vi "Run.vi"(8 "error in (no error)":errorcluster, 11 "Channel in":refnum<class "Channel.lvclass">) -> (0 "error out":errorcluster, 3 "Channel out":refnum<class "Channel.lvclass">)   [LabVIEW 2018, in "Channel.lvclass"]
uses:
  Channel.lvclass
  C:/Users/devstaff/sparc4/s4gui/Versao ZeroMQ REQ-REP/SPARC4_GUI -v1.0.9 - novo comportamento aba TEST/Device/Device.lvclass
  Channel.lvclass/Channel.ctl
  Interface/Interface.lvclass/Interface.ctl
  Device/Device.lvclass/Device.ctl
  StateMachine/State Machine.lvclass
  Interface/Interface.lvclass
  Device/Device.lvclass
panel:
  out "resp RESUME":string
  out "resp PAUSE":string
  out "x = y?":T1
  out "resposta do STATUS":string
  out "resp INIT":string
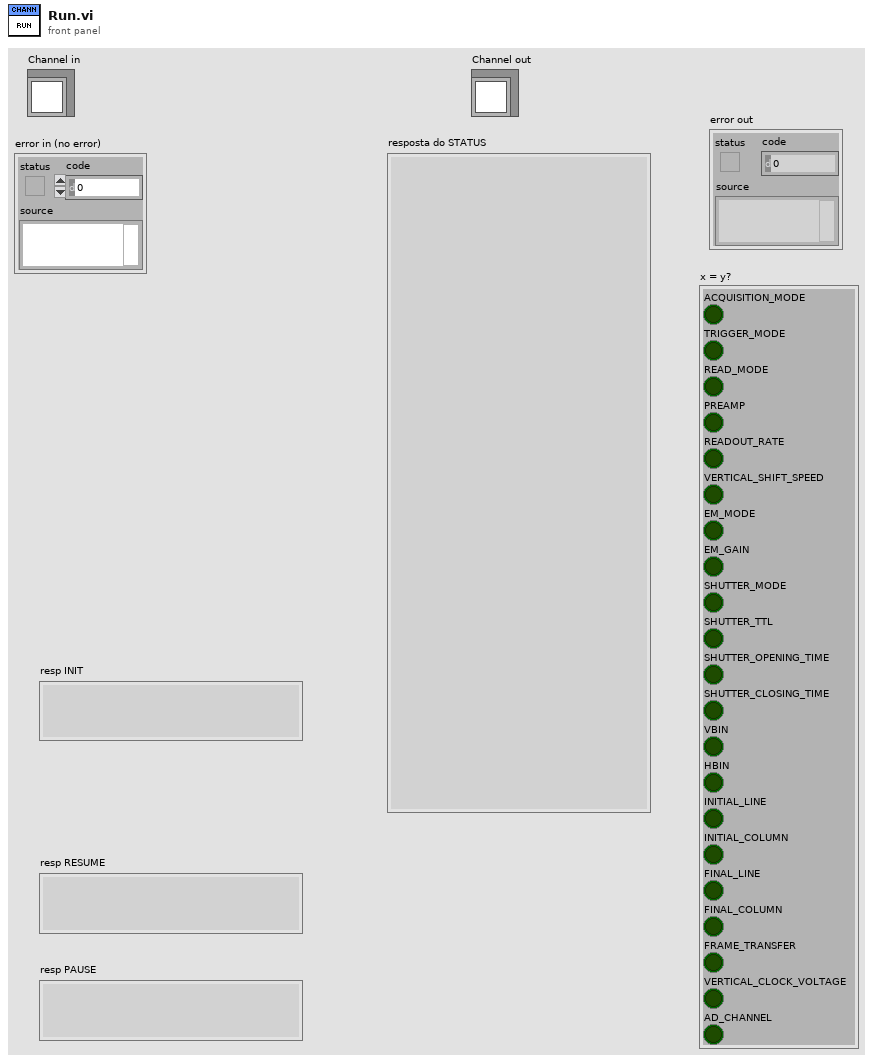
[diagram p1: front panel]
types:
  T1 = cluster{"ACQUISITION_MODE":bool, "TRIGGER_MODE":bool, "READ_MODE":bool, "PREAMP":bool, "READOUT_RATE":bool, "VERTICAL_SHIFT_SPEED":bool, "EM_MODE":bool, "EM_GAIN":bool, "SHUTTER_MODE":bool, "SHUTTER_TTL":bool, "SHUTTER_OPENING_TIME":bool, "SHUTTER_CLOSING_TIME":bool, "VBIN":bool, "HBIN":bool, "INITIAL_LINE":bool, "INITIAL_COLUMN":bool, "FINAL_LINE":bool, "FINAL_COLUMN":bool, "FRAME_TRANSFER":bool, "VERTICAL_CLOCK_VOLTAGE":bool, "AD_CHANNEL":bool}
  T2 = cluster{"TEMP":dbl, "EXPTIME":dbl, "#FRAMES":u32, "#CYCLES":u32, "#SEQS":u32, "WAVEPLATE_POS":u32, "COOLER_POWER_STATUS":dbl, "suffix":string}
  T3 = cluster{"ACQUISITION_MODE":u8, "TRIGGER_MODE":u8, "READ_MODE":u8, "PREAMP":u8, "READOUT_RATE":u8, "VERTICAL_SHIFT_SPEED":u8, "EM_MODE":u8, "EM_GAIN":u16, "SHUTTER_MODE":u8, "SHUTTER_TTL":u8, "SHUTTER_OPENING_TIME":u16, "SHUTTER_CLOSING_TIME":u16, "VBIN":u16, "HBIN":u16, "INITIAL_LINE":u16, "INITIAL_COLUMN":u16, "FINAL_LINE":u16, "FINAL_COLUMN":u16, "FRAME_TRANSFER":bool, "VERTICAL_CLOCK_VOLTAGE":u8, "AD_CHANNEL":u32}
  T4 = cluster{"Image Name":string, "Image Path":string, "#FRAMES":u32, "EXPTIME":dbl, "PREAMP":u8, "READOUT_RATE":u8, "VERTICAL_SHIFT_SPEED":u8, "ACQUISITION_MODE":u8, "READ_MODE":u8, "EM_MODE":u8, "EM_GAIN":u16, "SHUTTER_MODE":u8, "SHUTTER_TTL":u8, "SHUTTER_OPENNING_TIME":u16, "SHUTTER_CLOSING_TIME":u16, "VBIN":u16, "HBIN":u16, "INITIAL_LINE":u16, "INITIAL_COLUMN":u16, "FINAL_LINE":u16, "FINAL_COLUMN":u16, "Cooler ON/OFF":u16, "Set temperature":i8, "Exposições realizadas":u16, "Kinetic Serie Length":u32, "Number of Accumulations":u32, "Kinetic Cycle Time":u32, "FRAME_TRANSFER":bool, "VERTICAL_CLOCK_VOLTAGE":u8, "TRIGGER_MODE":u8, "Number of exp":u32, "AD_CHANNEL":u32}
  T5 = cluster{"OBSERVER":string, "OBJECT":string, "CTRLINTE":string, "PROJID":string, "SYNCMODE":string, "INSTMODE":string, "FILTER":string, "OBSTYPE":string, "CHANNEL 1":bool, "CHANNEL 2":bool, "CHANNEL 3":bool, "CHANNEL 4":bool, "TCSMODE":bool, "COMMENT":string, "broker":string, "GUIVRSN":string, "timestamp":string}
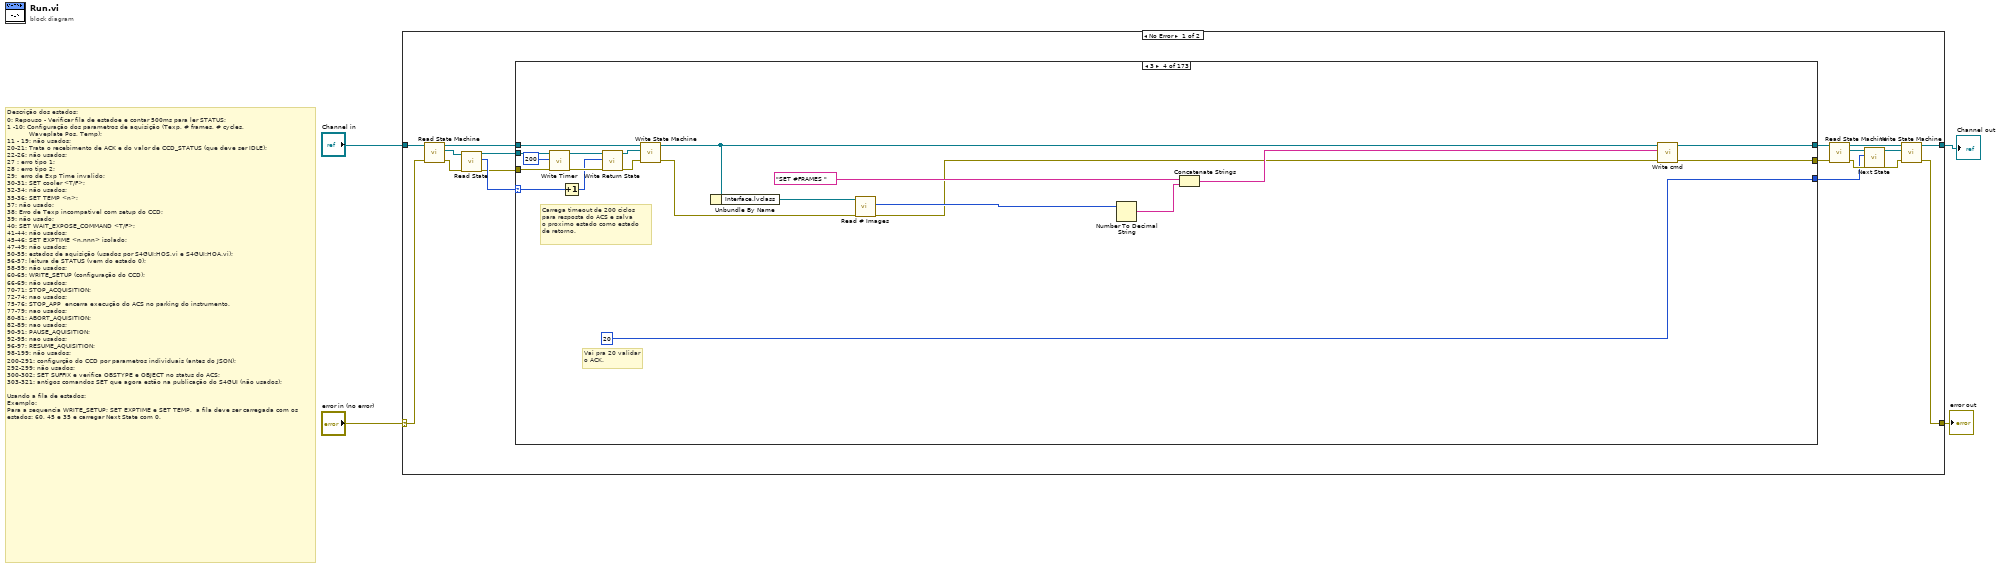
[diagram p0: block diagram]
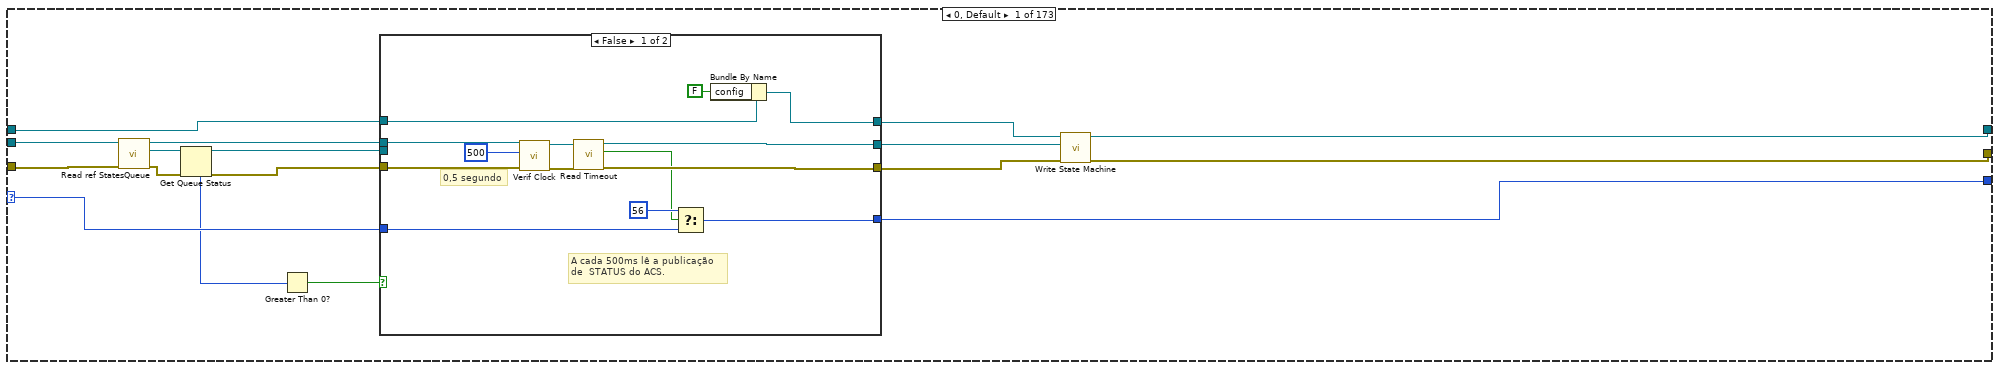
[diagram p2: hidden frame]
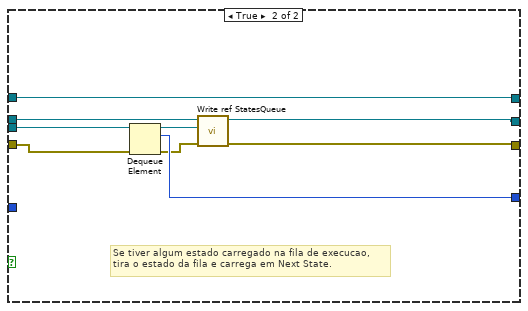
[diagram p3: hidden frame]
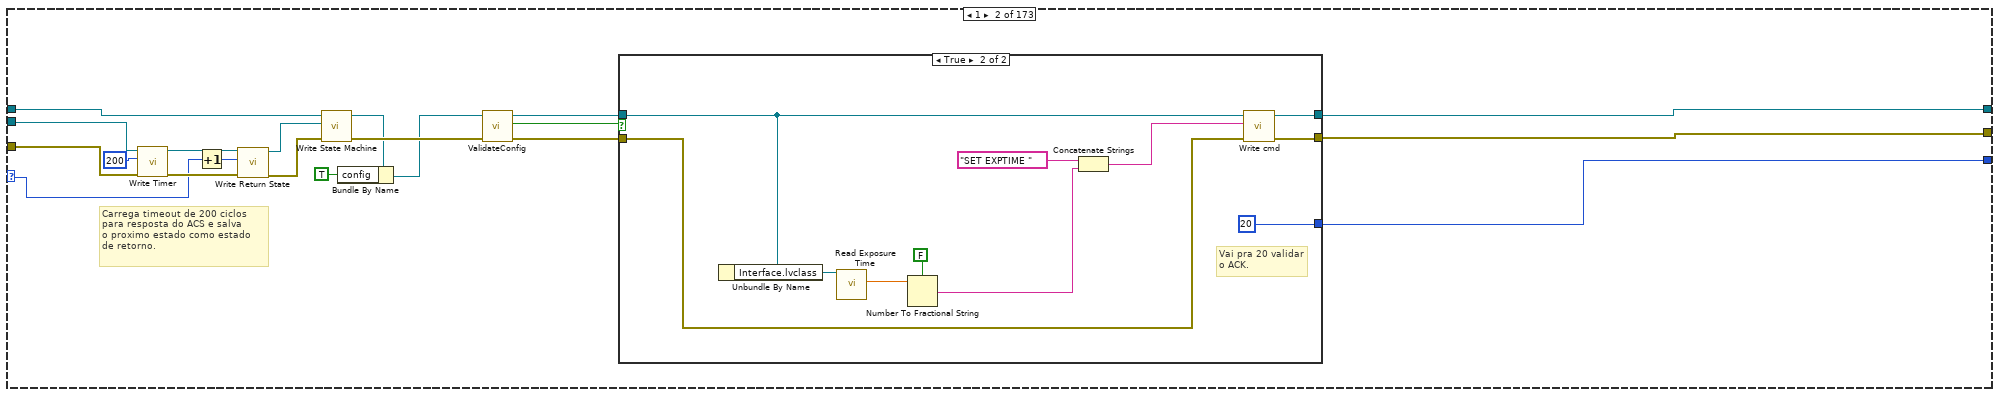
[diagram p4: hidden frame]
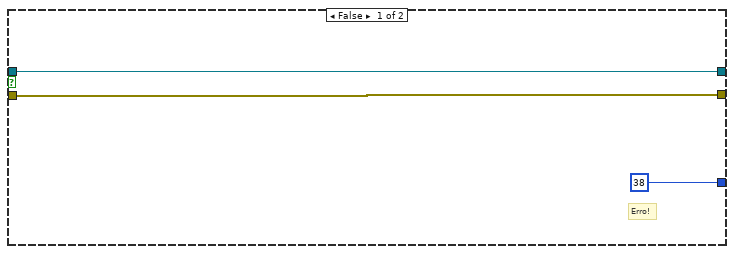
[diagram p5: hidden frame]
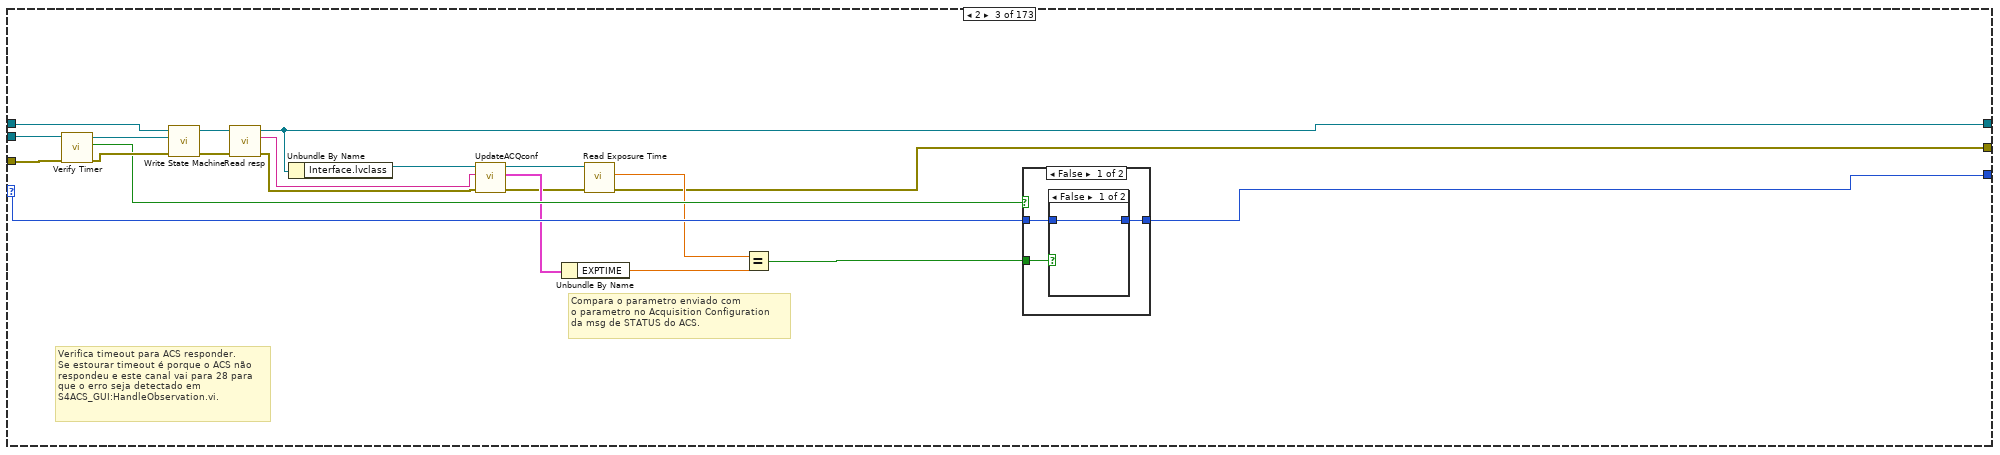
[diagram p6: hidden frame]
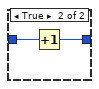
[diagram p7: hidden frame]
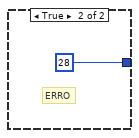
[diagram p8: hidden frame]
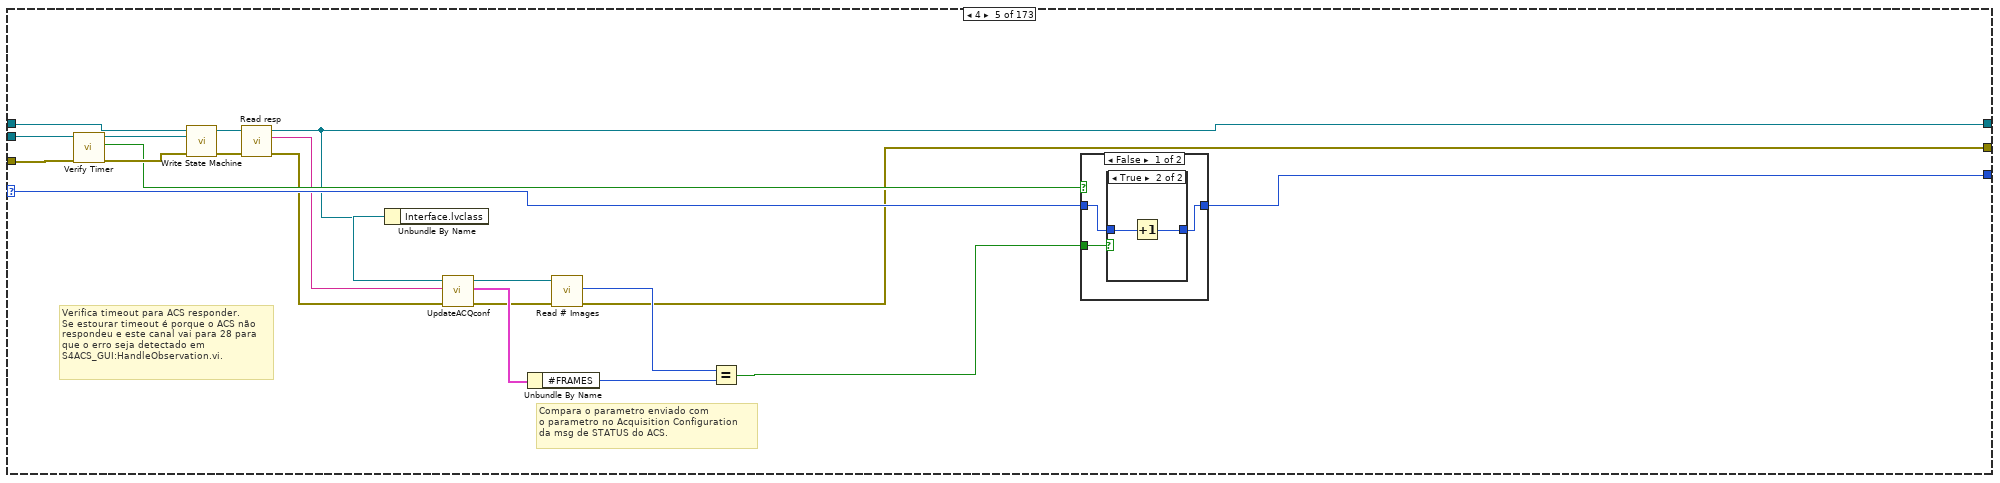
[diagram p9: hidden frame]
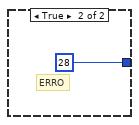
[diagram p11: hidden frame]
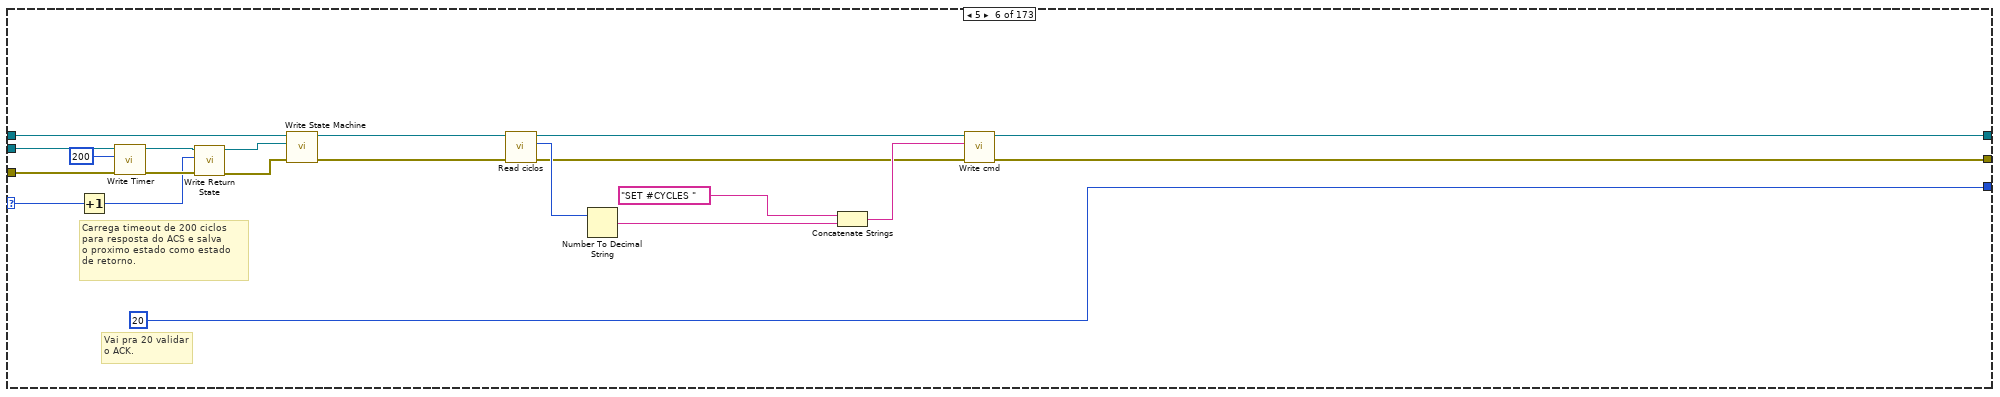
[diagram p12: hidden frame]
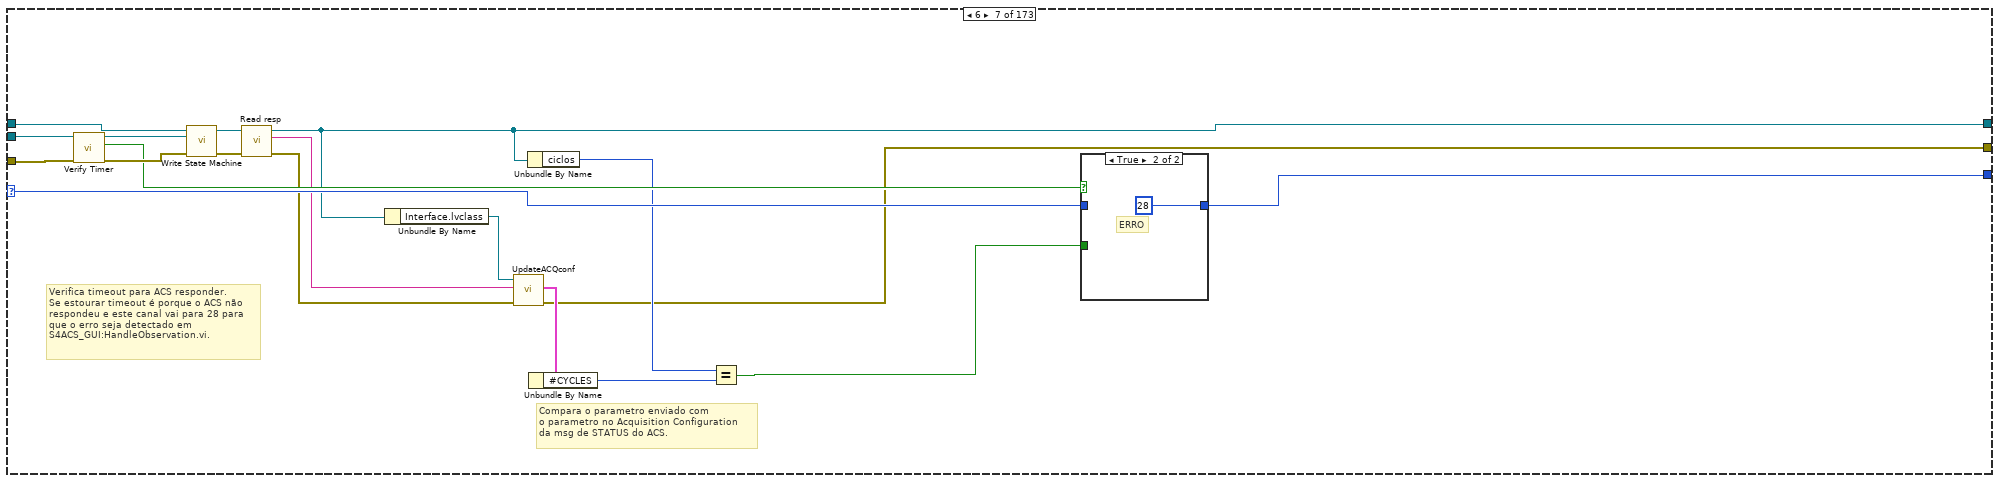
[diagram p13: hidden frame]
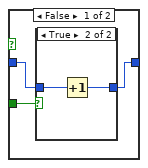
[diagram p14: hidden frame]
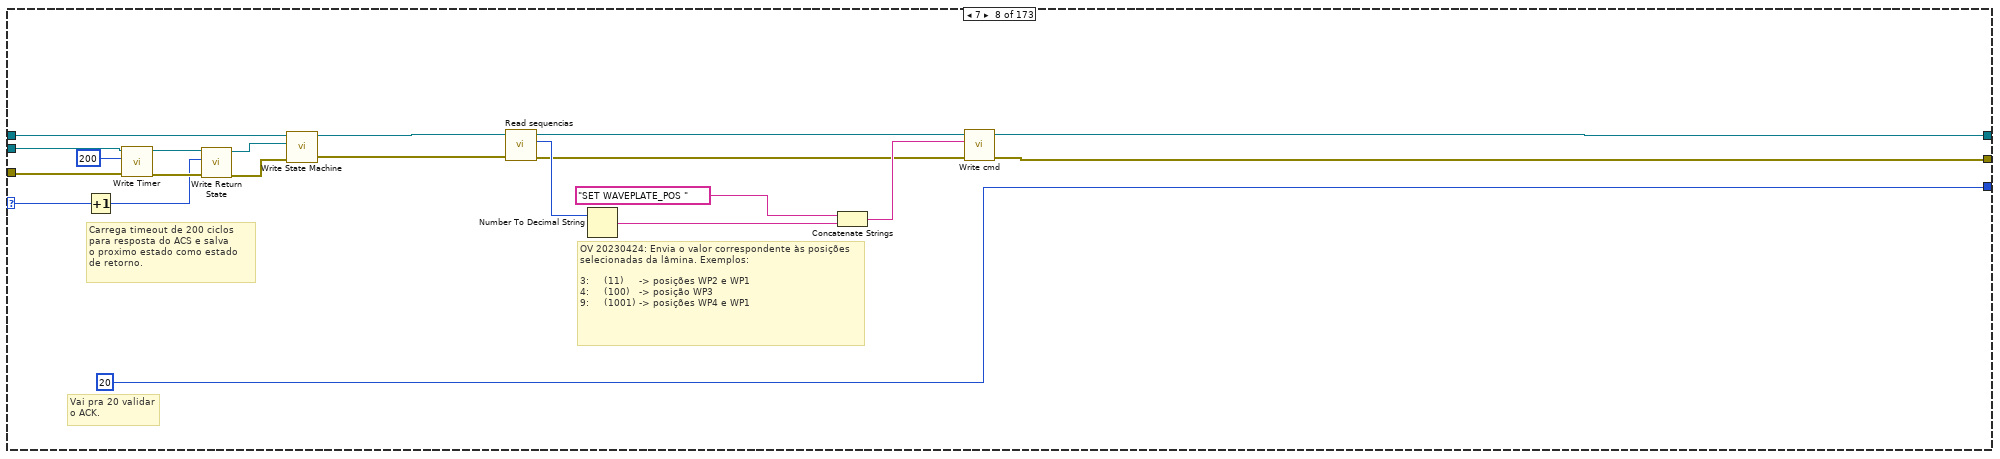
[diagram p16: hidden frame]
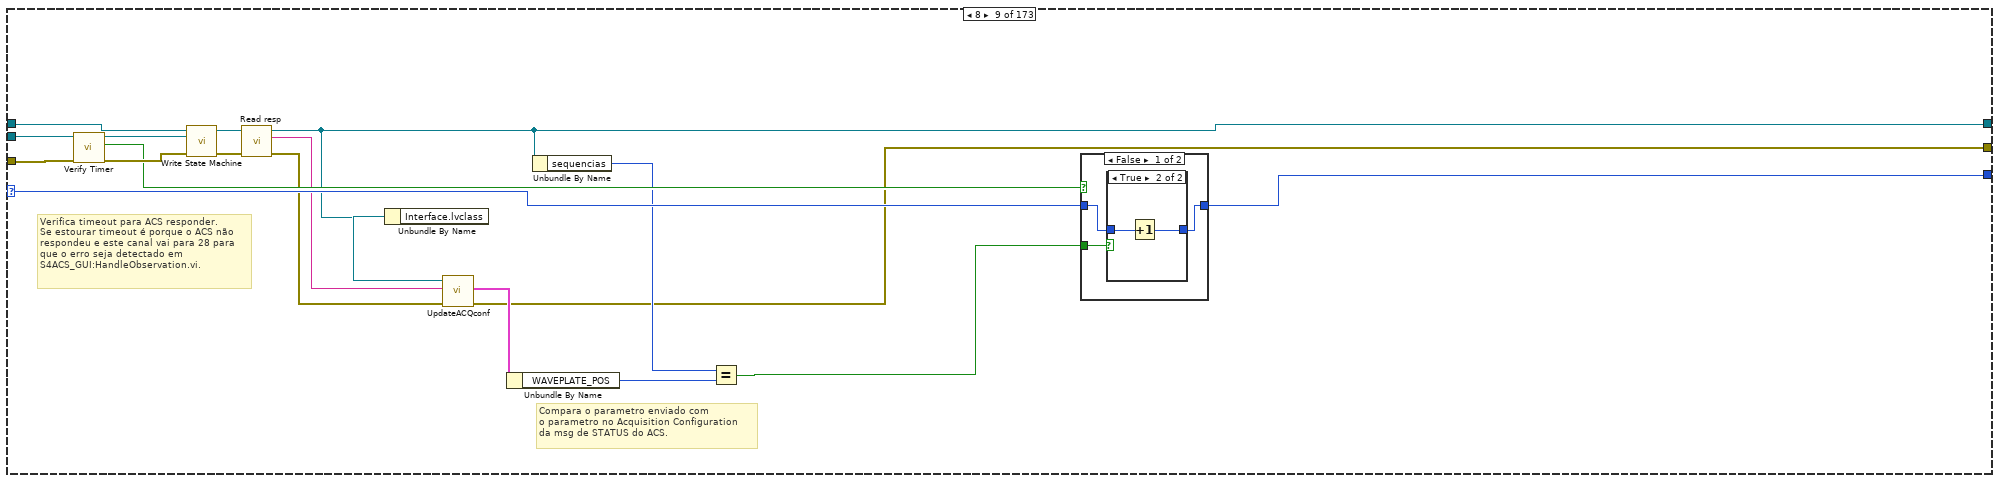
[diagram p17: hidden frame]
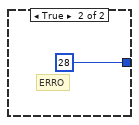
[diagram p19: hidden frame]
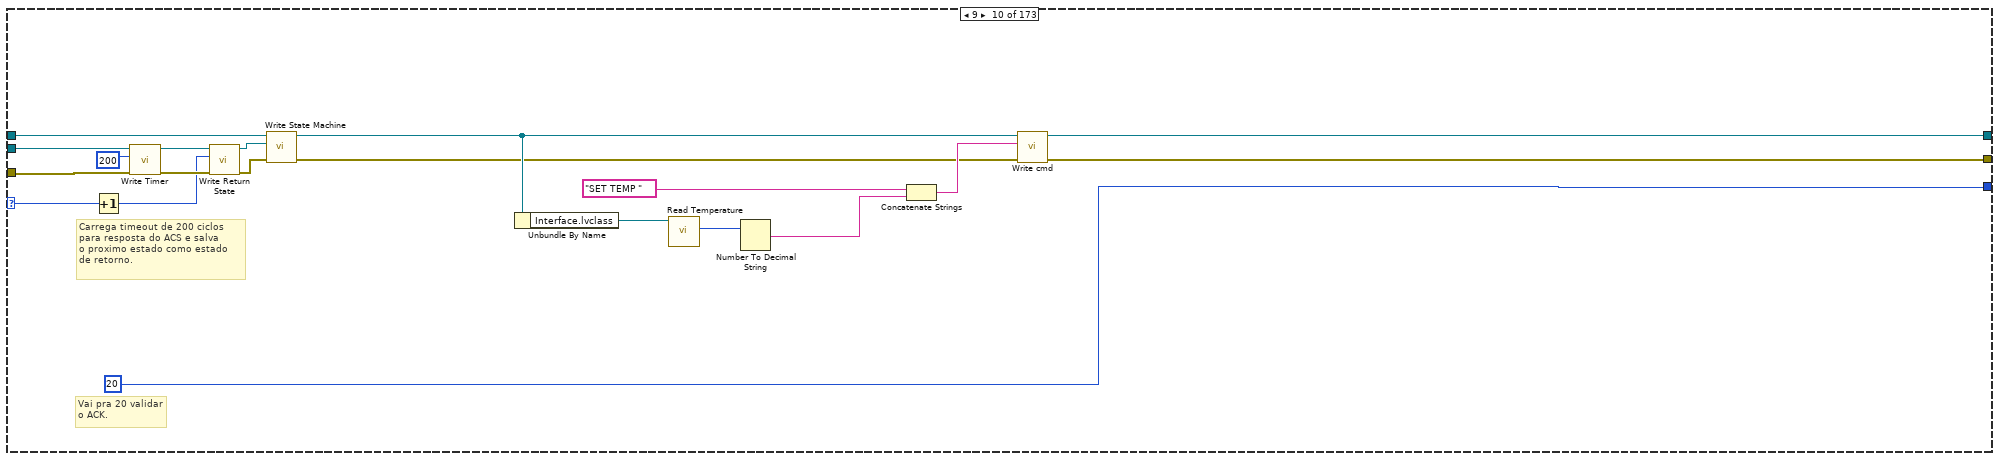
[diagram p20: hidden frame]
diagram:
  # "Descrição dos estados:\n0: Repouso - Verificar fila de estadoe e contar 500ms para ler STATUS;\n1 -10: Configuração dos parametros de aquisição (Texp, # frames, # cycles,\n           Waveplate Pos, Temp);\n11 - 19: não usados;\n20-21: Trata o recebimento de ACK e do valor de CCD_STATUS (que deve ser IDLE);\n22-26: não usados;\n27 : erro tipo 1;\n28 : erro tipo 2;\n29:  erro de Exp Time invalido;\n30-31: SET cooler <T/F>;\n32-34: não usados;\n35-36: SET TEMP <n>;\n37: não usado;\n38: Erro de Texp incompativel com setup do CCD;\n39: não usado;\n40: SET WAIT_EXPOSE_COMMAND <T/F>;\n41-44: não usados;\n45-46: SET EXPTIME <n.nnn> isolado;\n47-49: não usados;\n50-55: estados de aquisição (usados por S4GUI:HOS.vi e S4GUI:HOA.vi);\n56-57: leitura de STATUS (vem do estado 0);\n58-59: não usados;\n60-65: WRITE_SETUP (configuração do CCD);\n66-69: não usados;\n70-71: STOP_ACQUISITION;\n72-74: nao usados;\n75-76: STOP_APP  encerra execução do ACS no parking do instrumento.\n77-79: nao usados;\n80-81: ABORT_AQUISITION;\n82-89: nao usados;\n90-91: PAUSE_AQUISITION;\n92-95: nao usados;\n96-97: RESUME_AQUISITION;\n98-199: não usados;\n200-291: configurção do CCD por parametros individuais (antes do JSON);\n292-299: não usados;\n300-302: SET SUFFIX e verifica OBSTYPE e OBJECT no status do ACS;\n303-321: antigos comandos SET que agora estão na publicação do S4GUI (não usados);\n\nUsando a fila de estados:\nExemplo:\nPara a sequencia WRITE_SETUP; SET EXPTIME e SET TEMP,  a fila deve ser carregada com os \nestados: 60, 45 e 35 e carregar Next State com 0."
  n1 = case shown="No Error" "error in (no error)" {
    selector: "error in (no error)" -> [w21 w3263]
    tunnel: [w6 w3263] -> w3
    tunnel: [w11 w3262] -> w1
    tunnel: "Channel in" -> [w22 w3262]
    frame No Error {
      n2 = call-dynamic "Read State Machine.vi"("error in (no error)"=w21, "Device in"=w22) -> ("error out"=w18:errorcluster, "State Machine.lvclass"=w20:refnum<class "State Machine.lvclass">, "Device out"=w16:refnum<class "Channel.lvclass">)  [unwired: 7 in]
      n3 = call-dynamic "Read State.vi"("error in (no error)"=w18, "State Machine in"=w20) -> ("error out"=w17:errorcluster, "State"=w19:i32, "State Machine out"=w5:refnum<class "State Machine.lvclass">)  [unwired: 7 in]
      n4 = case shown="3" w19 {
        selector: w19 -> [w39 w64 w110 w127 w158 w176 w205 w221 w252 w269 w308 w330 w364 w442 w485 w528 w543 w571 w590 w603 w649 w678 _ w751 _ w790 w824 w850 w879 w890 w951 w972 w1046 w1086 w1154 _ _ w1262 w1293 w1314 w1352 w1365 w1381 w1447 w1481 w1506 w1514 w1558 w1564 w1586 w1592 w1635 _ w1660 _ w1679 w1690 w1710 w1730 w1750 w1770 w1790 w1810 w1830 w1850 _ w1870 w1878 w1891 w1904 w1920 w1928 w1941 w1955 w1967 w1975 w1988 w2001 w2013 w2021 w2034 w2047 w2059 w2067 w2080 w2093 w2105 w2113 w2126 w2139 w2151 w2159 w2172 w2185 w2197 w2205 w2218 w2231 w2243 w2251 w2264 w2277 w2293 w2301 w2314 w2327 w2339 w2347 w2360 w2373 w2385 w2393 w2406 w2419 w2431 w2439 w2452 w2465 w2477 w2485 w2498 w2511 w2523 w2531 w2544 w2557 w2569 w2577 w2590 w2603 w2615 w2623 w2636 w2649 w2661 w2669 w2682 w2695 w2707 w2715 w2728 w2741 w2753 w2761 w2774 w2787 w2803 w2811 w2824 w2837 w2849 w2859 w2872 w2885 w2899 w2907 w2920 w2933 w2953 w2986 w3007 w3025 w3054 w3079 w3092 w3121 w3127 w3153 w3165 w3190 w3202 w3227 w3239]
        tunnel: w17 -> [w32 w79 w114 w135 w161 w190 w208 w224 w255 w274 w307 w329 w363 w403 w446 w489 w535 w570 w585 w597 w647 w677 w702 w712 w765 w789 w828 w847 w872 w888 w912 w969 w1011 w1079 w1128 w1188 w1227 w1269 w1281 w1310 w1347 w1359 w1395 w1444 w1476 w1492 w1510 w1551 w1568 w1574 w1603 w1637 w1651 w1662 w1676 w1683 w1694 w1705 w1725 w1745 w1765 w1785 w1805 w1825 w1845 w1863 w1876 w1885 w1895 w1907 w1926 w1935 w1945 w1958 w1973 w1982 w1992 w2004 w2019 w2028 w2038 w2050 w2065 w2074 w2084 w2096 w2111 w2120 w2130 w2142 w2157 w2166 w2176 w2188 w2203 w2212 w2222 w2234 w2249 w2258 w2268 w2280 w2299 w2308 w2318 w2330 w2345 w2354 w2364 w2376 w2391 w2400 w2410 w2422 w2437 w2446 w2456 w2468 w2483 w2492 w2502 w2514 w2529 w2538 w2548 w2560 w2575 w2584 w2594 w2606 w2621 w2630 w2640 w2652 w2667 w2676 w2686 w2698 w2713 w2722 w2732 w2744 w2759 w2768 w2778 w2790 w2809 w2818 w2828 w2840 w2855 w2866 w2876 w2888 w2905 w2914 w2924 w2936 w2946 w2990 w3014 w3037 w3058 w3073 w3098 w3115 w3133 w3155 w3167 w3192 w3204 w3229 w3241]
        tunnel: [w35 w81 w97 w144 w146 w193 w195 w240 w242 w287 w290 w316 w359 w400 w443 w486 w547 w551 w592 w605 w657 w660 w707 w709 w769 w792 w811 w842 w866 w892 w943 w957 w1021 w1074 w1129 w1200 w1238 w1268 w1294 w1315 w1344 w1367 w1382 w1449 w1463 w1494 w1512 w1539 w1565 w1582 w1590 w1632 w1649 w1657 w1671 w1682 w1691 w1705 w1725 w1745 w1765 w1785 w1805 w1825 w1845 w1863 w1875 w1879 w1894 w1905 w1925 w1929 w1944 w1956 w1972 w1976 w1991 w2002 w2018 w2022 w2037 w2048 w2064 w2068 w2083 w2094 w2110 w2114 w2129 w2140 w2156 w2160 w2175 w2186 w2202 w2206 w2221 w2232 w2248 w2252 w2267 w2278 w2298 w2302 w2317 w2328 w2344 w2348 w2363 w2374 w2390 w2394 w2409 w2420 w2436 w2440 w2455 w2466 w2482 w2486 w2501 w2512 w2528 w2532 w2547 w2558 w2574 w2578 w2593 w2604 w2620 w2624 w2639 w2650 w2666 w2670 w2685 w2696 w2712 w2716 w2731 w2742 w2758 w2762 w2777 w2788 w2808 w2812 w2827 w2838 w2854 w2860 w2875 w2886 w2904 w2908 w2923 w2934 w2957 w2972 w3010 w3039 w3041 w3082 w3101 w3123 w3136 w3161 w3174 w3198 w3211 w3235 w3248] -> w7
        tunnel: w16 -> [w24 w77 w117 w136 w165 w191 w212 w239 w259 w280 w306 w321 w356 w402 w445 w488 w538 w569 w587 w600 w646 w676 w705 w711 w766 w787 w831 w841 w878 w889 w925 w965 w1020 w1081 w1122 w1199 w1237 w1263 w1285 w1308 w1348 w1360 w1396 w1443 w1479 w1491 w1511 w1552 w1569 w1576 w1601 w1629 w1652 w1654 w1677 w1681 w1695 w1703 w1723 w1743 w1763 w1783 w1803 w1823 w1843 w1865 w1874 w1886 w1893 w1908 w1924 w1936 w1943 w1959 w1971 w1983 w1990 w2005 w2017 w2029 w2036 w2051 w2063 w2075 w2082 w2097 w2109 w2121 w2128 w2143 w2155 w2167 w2174 w2189 w2201 w2213 w2220 w2235 w2247 w2259 w2266 w2281 w2297 w2309 w2316 w2331 w2343 w2355 w2362 w2377 w2389 w2401 w2408 w2423 w2435 w2447 w2454 w2469 w2481 w2493 w2500 w2515 w2527 w2539 w2546 w2561 w2573 w2585 w2592 w2607 w2619 w2631 w2638 w2653 w2665 w2677 w2684 w2699 w2711 w2723 w2730 w2745 w2757 w2769 w2776 w2791 w2807 w2819 w2826 w2841 w2853 w2867 w2874 w2889 w2903 w2915 w2922 w2937 w2947 w2993 w3013 w3035 w3061 w3075 w3099 w3117 w3134 w3156 w3171 w3193 w3208 w3230 w3245]
        tunnel: [w38 w82 w106 w145 w149 w194 w197 w241 w244 w281 w292 w322 w360 w441 w484 w527 w548 w552 w593 w608 w650 w662 w708 w750 w755 w793 w820 w843 w867 w893 w950 w958 w1045 w1075 w1153 w1201 w1239 w1270 w1295 w1316 w1345 w1368 w1392 w1450 w1461 w1500 w1508 w1545 w1566 w1581 w1588 w1631 w1650 w1656 w1675 w1684 w1687 w1707 w1727 w1747 w1767 w1787 w1807 w1827 w1847 w1865 w1877 w1880 w1896 w1903 w1927 w1930 w1946 w1954 w1974 w1977 w1993 w2000 w2020 w2023 w2039 w2046 w2066 w2069 w2085 w2092 w2112 w2115 w2131 w2138 w2158 w2161 w2177 w2184 w2204 w2207 w2223 w2230 w2250 w2253 w2269 w2276 w2300 w2303 w2319 w2326 w2346 w2349 w2365 w2372 w2392 w2395 w2411 w2418 w2438 w2441 w2457 w2464 w2484 w2487 w2503 w2510 w2530 w2533 w2549 w2556 w2576 w2579 w2595 w2602 w2622 w2625 w2641 w2648 w2668 w2671 w2687 w2694 w2714 w2717 w2733 w2740 w2760 w2763 w2779 w2786 w2810 w2813 w2829 w2836 w2856 w2861 w2877 w2884 w2906 w2909 w2925 w2932 w2958 w2983 w3009 w3040 w3050 w3083 w3102 w3124 w3137 w3162 w3175 w3199 w3212 w3236 w3249] -> w14
        tunnel: [w34 w80 w109 u32 20 w157 u32 20 w204 u32 20 w251 u32 20 w309 w331 w365 w442 w485 w528 w544 w572 w591 w604 w651 w679 31 ("State") w751 w762 w791 w823 w848 w880 w891 w952 w973 w1047 w1087 w1155 0 ("State") 54 ("State") w1261 w1296 w1313 w1353 w1366 w1380 w1448 w1482 w1507 w1528 w1559 w1567 w1587 w1614 w1636 0 ("State") w1661 0 ("State") w1680 w1692 w1702 w1722 w1742 w1762 w1782 w1802 w1822 w1842 u8 0 ("State") w1871 w1881 w1892 w1906 w1921 w1931 w1942 w1957 w1968 w1978 w1989 w2003 w2014 w2024 w2035 w2049 w2060 w2070 w2081 w2095 w2106 w2116 w2127 w2141 w2152 w2162 w2173 w2187 w2198 w2208 w2219 w2233 w2244 w2254 w2265 w2279 w2294 w2304 w2315 w2329 w2340 w2350 w2361 w2375 w2386 w2396 w2407 w2421 w2432 w2442 w2453 w2467 w2478 w2488 w2499 w2513 w2524 w2534 w2545 w2559 w2570 w2580 w2591 w2605 w2616 w2626 w2637 w2651 w2662 w2672 w2683 w2697 w2708 w2718 w2729 w2743 w2754 w2764 w2775 w2789 w2804 w2814 w2825 w2839 w2850 w2862 w2873 w2887 w2900 w2910 w2921 w2935 w2954 w2985 w3008 u32 20 w3053 w3080 w3090 w3122 w3125 w3160 w3166 w3197 w3203 w3234 w3237] -> w8
        tunnel: w5 -> [w33 w78 w116 w137 w166 w189 w213 w227 w260 w271 w304 w328 w362 _ _ _ w537 w567 w586 w601 w645 w674 w704 _ w767 w788 w830 w846 w876 _ w915 w970 w1013 w1083 w1127 w1189 w1228 w1265 w1286 w1311 w1349 w1362 w1397 w1445 w1480 _ _ w1553 _ w1578 w1604 _ _ _ _ _ _ _ _ _ _ _ _ _ _ _ _ _ _ _ _ _ _ _ _ _ _ _ _ _ _ _ _ _ _ _ _ _ _ _ _ _ _ _ _ _ _ _ _ _ _ _ _ _ _ _ _ _ _ _ _ _ _ _ _ _ _ _ _ _ _ _ _ _ _ _ _ _ _ _ _ _ _ _ _ _ _ _ _ _ _ _ _ _ _ _ _ _ _ _ _ _ _ _ _ _ _ _ w2949 w2992 w3015 w3036 w3060 w3071 w3096 w3114 w3131 w3154 w3168 w3191 w3205 w3228 w3242]
        frame 0, Default {
          n5 = call-dynamic "Read ref StatesQueue.vi"("error in (no error)"=w32, "State Machine in"=w33) -> ("error out"=w27:errorcluster, "ref StatesQueue"=w30:refnum<queue>, "State Machine out"=w31:refnum<class "State Machine.lvclass">)  [unwired: 7 in]
          n6 = Get Queue Status(queue=w30, error in (no error)=w27) -> (queue out=w25:refnum<queue>, error out=w26:errorcluster, # elements in queue=w29:i32)  [unwired: 1 in, 5 out]
          n7 = Greater Than 0?(x=w29) -> (x > 0?=w28:bool)
          n8 = case shown="False" w28 {
            tunnel: w39 -> [w49 _]
            tunnel: w31 -> [w48 w59]
            tunnel: w26 -> [w47 w61]
            tunnel: [w46 w55] -> w37
            tunnel: [w45 w56] -> w36
            tunnel: [w43 w60] -> w34
            tunnel: w25 -> [_ w62]
            tunnel: [w41 w54] -> w23
            tunnel: w24 -> [w42 w54]
            frame False {
              # "A cada 500ms lê a publicação \nde  STATUS do ACS."
              # "0,5 segundo"
              n9 = call-dynamic "Verif Clock.vi"("error in (no error)"=w47, "period (ms)"=u32 500 ("period"), "State Machine in"=w48) -> ("error out"=w52:errorcluster, "State Machine out"=w51:refnum<class "State Machine.lvclass">)  [unwired: 6 in, 1 out]
              n10 = call-dynamic "Read Timeout.vi"("error in (no error)"=w52, "State Machine in"=w51) -> ("error out"=w46:errorcluster, "Timeout"=w44:bool, "State Machine out"=w45:refnum<class "State Machine.lvclass">)  [unwired: 7 in]
              n11 = Select(t=56 ("State"), s=w44, f=w49) -> (s? t:f=w43:i32)
              n12 = Bundle By Name(cluster=w42, "config"=FALSE) -> (w41:refnum<class "Channel.lvclass">)
            }
            frame True {
              # "Se tiver algum estado carregado na fila de execucao,\ntira o estado da fila e carrega em Next State."
              n13 = Dequeue Element(queue=w62, error in (no error)=w61) -> (queue out=w58:refnum<queue>, element=w60:u32, error out=w57:errorcluster)  [unwired: 1 in, 1 out]
              n14 = call-dynamic "Write ref StatesQueue.vi"("error in (no error)"=w57, "ref StatesQueue"=w58, "State Machine in"=w59) -> ("error out"=w55:errorcluster, "State Machine out"=w56:refnum<class "State Machine.lvclass">)  [unwired: 7 in]
            }
          }
          n15 = call-dynamic "Write State Machine.vi"("error in (no error)"=w37, "State Machine.lvclass"=w36, "Device in"=w23) -> ("error out"=w35:errorcluster, "Device out"=w38:refnum<class "Channel.lvclass">)  [unwired: 7 in]
        }
        frame 1 {
          # "Carrega timeout de 200 ciclos\npara resposta do ACS e salva\no proximo estado como estado \nde retorno."
          n16 = call-dynamic "Write Timer.vi"("error in (no error)"=w79, "Timer"=u32 200, "State Machine in"=w78) -> ("error out"=w66:errorcluster, "State Machine out"=w68:refnum<class "State Machine.lvclass">)  [unwired: 7 in]
          n17 = Increment(x=w64) -> (x+1=w63:i32)
          n18 = call-dynamic "Write Return State.vi"("error in (no error)"=w66, "Return State"=w63, "State Machine in"=w68) -> ("error out"=w65:errorcluster, "State Machine out"=w67:refnum<class "State Machine.lvclass">)  [unwired: 7 in]
          n19 = call-dynamic "Write State Machine.vi"("error in (no error)"=w65, "State Machine.lvclass"=w67, "Device in"=w77) -> ("error out"=w75:errorcluster, "Device out"=w71:refnum<class "Channel.lvclass">)  [unwired: 7 in]
          n20 = Bundle By Name(cluster=w71, "config"=TRUE) -> (w70:refnum<class "Channel.lvclass">)
          n21 = call-dynamic "ValidateConfig.vi"("error in (no error)"=w75, "Channel in"=w70) -> ("error out"=w73:errorcluster, "valid?"=w72:bool, "Channel out"=w74:refnum<class "Channel.lvclass">)  [unwired: 7 in]
          n22 = case shown="True" w72 {
            tunnel: [w85 w96] -> w82
            tunnel: [w84 w95] -> w81
            tunnel: [38 u32 20] -> w80
            tunnel: w74 -> [w85 w88]
            tunnel: w73 -> [w84 w87]
            frame False {
              # "Erro!"
            }
            frame True {
              # "Vai pra 20 validar\no ACK."
              n23 = Unbundle By Name(w88) -> ("Interface.lvclass"=w94:refnum<class "Interface.lvclass">)
              n24 = call "Read Exposure Time.vi"("Interface in"=w94) -> ("Exposure Time"=w93:dbl)  [unwired: 8 in, 2 out]
              n25 = Number To Fractional String(use system decimal point (T)=FALSE, number=w93) -> (F-format string=w92:string)  [unwired: 2 in]
              n26 = Concatenate Strings("SET EXPTIME " ("cmd"), w92) -> (w91:string)
              n27 = call-dynamic "Write cmd.vi"("error in (no error)"=w87, "cmd"=w91, "Device in"=w88) -> ("error out"=w95:errorcluster, "Device out"=w96:refnum<class "Channel.lvclass">)  [unwired: 7 in]
            }
          }
        }
        frame 2 {
          # "Compara o parametro enviado com\no parametro no Acquisition Configuration\nda msg de STATUS do ACS."
          # "Verifica timeout para ACS responder.\nSe estourar timeout é porque o ACS não \nrespondeu e este canal vai para 28 para \nque o erro seja detectado em\nS4ACS_GUI:HandleObservation.vi."
          n28 = call "Verify Timer.vi"("error in (no error)"=w114, "State Machine in"=w116) -> ("error out"=w113:errorcluster, "timeout"=w111:bool, "State Machine out"=w115:refnum<class "State Machine.lvclass">)  [unwired: 7 in]
          n29 = call-dynamic "Write State Machine.vi"("error in (no error)"=w113, "State Machine.lvclass"=w115, "Device in"=w117) -> ("error out"=w112:errorcluster, "Device out"=w108:refnum<class "Channel.lvclass">)  [unwired: 7 in]
          n30 = call-dynamic "Read resp.vi"("error in (no error)"=w112, "Device in"=w108) -> ("error out"=w99:errorcluster, "resp"=w107:string, "Device out"=w106:refnum<class "Channel.lvclass">)  [unwired: 7 in]
          n31 = Unbundle By Name(w106) -> ("Interface.lvclass"=w105:refnum<class "Interface.lvclass">)
          n32 = call-dynamic "UpdateACQconf.vi"("error in (no error)"=w99, "status"=w107, "Interface in"=w105) -> ("error out"=w98:errorcluster, "ACQ conf rx"=w103:T2, "Interface out"=w104:refnum<class "Interface.lvclass">)  [unwired: 6 in]
          n33 = Unbundle By Name(w103) -> ("EXPTIME"=w101:dbl)
          n34 = call "Read Exposure Time.vi"("error in (no error)"=w98, "Interface in"=w104) -> ("error out"=w97:errorcluster, "Exposure Time"=w102:dbl)  [unwired: 7 in, 1 out]
          n35 = Equal?(x=w102, y=w101) -> (x = y?=w100:bool)
          n36 = case shown="False" w111 {
            tunnel: [w119 28] -> w109
            tunnel: w110 -> [w120 _]
            tunnel: w100 -> [w118 _]
            frame False {
              n37 = case shown="False" w118 {
                tunnel: [w121 w122] -> w119
                tunnel: w120 -> [w121 w123]
                frame False {
                }
                frame True {
                  n38 = Increment(x=w123) -> (x+1=w122:i32)
                }
              }
            }
            frame True {
              # "ERRO"
            }
          }
        }
        frame 3 {
          # "Vai pra 20 validar\no ACK."
          # "Carrega timeout de 200 ciclos\npara resposta do ACS e salva\no proximo estado como estado \nde retorno."
          n39 = call-dynamic "Write Timer.vi"("error in (no error)"=w135, "Timer"=u32 200, "State Machine in"=w137) -> ("error out"=w131:errorcluster, "State Machine out"=w129:refnum<class "State Machine.lvclass">)  [unwired: 7 in]
          n40 = Increment(x=w127) -> (x+1=w126:i32)
          n41 = call-dynamic "Write Return State.vi"("error in (no error)"=w131, "Return State"=w126, "State Machine in"=w129) -> ("error out"=w130:errorcluster, "State Machine out"=w128:refnum<class "State Machine.lvclass">)  [unwired: 7 in]
          n42 = call-dynamic "Write State Machine.vi"("error in (no error)"=w130, "State Machine.lvclass"=w128, "Device in"=w136) -> ("error out"=w133:errorcluster, "Device out"=w134:refnum<class "Channel.lvclass">)  [unwired: 7 in]
          n43 = Unbundle By Name(w134) -> ("Interface.lvclass"=w143:refnum<class "Interface.lvclass">)
          n44 = call-dynamic "Read # Images.vi"("error in (no error)"=w133, "Interface in"=w143) -> ("error out"=w132:errorcluster, "# Images"=w142:u32)  [unwired: 7 in, 1 out]
          n45 = Number To Decimal String(number=w142) -> (decimal integer string=w141:string)  [unwired: 1 in]
          n46 = Concatenate Strings("SET #FRAMES " ("cmd"), w141) -> (w140:string)
          n47 = call-dynamic "Write cmd.vi"("error in (no error)"=w132, "cmd"=w140, "Device in"=w134) -> ("error out"=w144:errorcluster, "Device out"=w145:refnum<class "Channel.lvclass">)  [unwired: 7 in]
        }
        frame 4 {
          # "Verifica timeout para ACS responder.\nSe estourar timeout é porque o ACS não \nrespondeu e este canal vai para 28 para \nque o erro seja detectado em\nS4ACS_GUI:HandleObservation.vi."
          # "Compara o parametro enviado com\no parametro no Acquisition Configuration\nda msg de STATUS do ACS."
          n48 = call "Verify Timer.vi"("error in (no error)"=w161, "State Machine in"=w166) -> ("error out"=w160:errorcluster, "timeout"=w159:bool, "State Machine out"=w162:refnum<class "State Machine.lvclass">)  [unwired: 7 in]
          n49 = call-dynamic "Write State Machine.vi"("error in (no error)"=w160, "State Machine.lvclass"=w162, "Device in"=w165) -> ("error out"=w163:errorcluster, "Device out"=w164:refnum<class "Channel.lvclass">)  [unwired: 7 in]
          n50 = call-dynamic "Read resp.vi"("error in (no error)"=w163, "Device in"=w164) -> ("error out"=w147:errorcluster, "resp"=w148:string, "Device out"=w149:refnum<class "Channel.lvclass">)  [unwired: 7 in]
          n51 = Unbundle By Name(w149) -> ("Interface.lvclass"=w156:refnum<class "Interface.lvclass">)
          n52 = call-dynamic "UpdateACQconf.vi"("error in (no error)"=w147, "status"=w148, "Interface in"=w156) -> ("error out"=w151:errorcluster, "ACQ conf rx"=w154:T2, "Interface out"=w155:refnum<class "Interface.lvclass">)  [unwired: 6 in]
          n53 = Unbundle By Name(w154) -> ("#FRAMES"=w152:u32)
          n54 = call-dynamic "Read # Images.vi"("error in (no error)"=w151, "Interface in"=w155) -> ("error out"=w146:errorcluster, "# Images"=w153:u32)  [unwired: 7 in, 1 out]
          n55 = Equal?(x=w153, y=w152) -> (x = y?=w150:bool)
          n56 = case shown="False" w159 {
            tunnel: [w168 28] -> w157
            tunnel: w158 -> [w169 _]
            tunnel: w150 -> [w167 _]
            frame False {
              n57 = case shown="True" w167 {
                tunnel: [w170 w171] -> w168
                tunnel: w169 -> [w170 w172]
                frame False {
                }
                frame True {
                  n58 = Increment(x=w172) -> (x+1=w171:i32)
                }
              }
            }
            frame True {
              # "ERRO"
            }
          }
        }
        frame 5 {
          # "Carrega timeout de 200 ciclos\npara resposta do ACS e salva\no proximo estado como estado \nde retorno."
          # "Vai pra 20 validar\no ACK."
          n59 = Increment(x=w176) -> (x+1=w175:i32)
          n60 = call-dynamic "Write Timer.vi"("error in (no error)"=w190, "Timer"=u32 200, "State Machine in"=w189) -> ("error out"=w178:errorcluster, "State Machine out"=w180:refnum<class "State Machine.lvclass">)  [unwired: 7 in]
          n61 = call-dynamic "Write Return State.vi"("error in (no error)"=w178, "Return State"=w175, "State Machine in"=w180) -> ("error out"=w177:errorcluster, "State Machine out"=w179:refnum<class "State Machine.lvclass">)  [unwired: 7 in]
          n62 = call-dynamic "Write State Machine.vi"("error in (no error)"=w177, "State Machine.lvclass"=w179, "Device in"=w191) -> ("error out"=w187:errorcluster, "Device out"=w188:refnum<class "Channel.lvclass">)  [unwired: 7 in]
          n63 = call-dynamic "Read ciclos.vi"("error in (no error)"=w187, "Channel in"=w188) -> ("error out"=w181:errorcluster, "ciclos"=w185:u32, "Channel out"=w186:refnum<class "Channel.lvclass">)  [unwired: 7 in]
          n64 = Number To Decimal String(number=w185) -> (decimal integer string=w183:string)  [unwired: 1 in]
          n65 = Concatenate Strings("SET #CYCLES " ("cmd"), w183) -> (w182:string)
          n66 = call-dynamic "Write cmd.vi"("error in (no error)"=w181, "cmd"=w182, "Device in"=w186) -> ("error out"=w193:errorcluster, "Device out"=w194:refnum<class "Channel.lvclass">)  [unwired: 7 in]
        }
        frame 6 {
          # "Verifica timeout para ACS responder.\nSe estourar timeout é porque o ACS não \nrespondeu e este canal vai para 28 para \nque o erro seja detectado em\nS4ACS_GUI:HandleObservation.vi."
          # "Compara o parametro enviado com\no parametro no Acquisition Configuration\nda msg de STATUS do ACS."
          n67 = call "Verify Timer.vi"("error in (no error)"=w208, "State Machine in"=w213) -> ("error out"=w207:errorcluster, "timeout"=w206:bool, "State Machine out"=w209:refnum<class "State Machine.lvclass">)  [unwired: 7 in]
          n68 = call-dynamic "Write State Machine.vi"("error in (no error)"=w207, "State Machine.lvclass"=w209, "Device in"=w212) -> ("error out"=w210:errorcluster, "Device out"=w211:refnum<class "Channel.lvclass">)  [unwired: 7 in]
          n69 = call-dynamic "Read resp.vi"("error in (no error)"=w210, "Device in"=w211) -> ("error out"=w198:errorcluster, "resp"=w199:string, "Device out"=w197:refnum<class "Channel.lvclass">)  [unwired: 7 in]
          n70 = Unbundle By Name(w197) -> ("Interface.lvclass"=w203:refnum<class "Interface.lvclass">)
          n71 = call-dynamic "UpdateACQconf.vi"("error in (no error)"=w198, "status"=w199, "Interface in"=w203) -> ("error out"=w195:errorcluster, "ACQ conf rx"=w202:T2)  [unwired: 6 in, 1 out]
          n72 = Unbundle By Name(w197) -> ("ciclos"=w196:u32)
          n73 = Unbundle By Name(w202) -> ("#CYCLES"=w201:u32)
          n74 = Equal?(x=w196, y=w201) -> (x = y?=w200:bool)
          n75 = case shown="True" w206 {
            tunnel: [w215 28] -> w204
            tunnel: w205 -> [w216 _]
            tunnel: w200 -> [w214 _]
            frame False {
              n76 = case shown="True" w214 {
                tunnel: [w217 w218] -> w215
                tunnel: w216 -> [w217 w219]
                frame False {
                }
                frame True {
                  n77 = Increment(x=w219) -> (x+1=w218:i32)
                }
              }
            }
            frame True {
              # "ERRO"
            }
          }
        }
        frame 7 {
          # "Vai pra 20 validar\no ACK."
          # "Carrega timeout de 200 ciclos\npara resposta do ACS e salva\no proximo estado como estado \nde retorno."
          # "OV 20230424: Envia o valor correspondente às posições\nselecionadas da lâmina. Exemplos:\n\n3:     (11)     -> posições WP2 e WP1\n4:     (100)   -> posição WP3\n9:     (1001) -> posições WP4 e WP1"
          n78 = Increment(x=w221) -> (x+1=w228:i32)
          n79 = call-dynamic "Write Timer.vi"("error in (no error)"=w224, "Timer"=u32 200, "State Machine in"=w227) -> ("error out"=w229:errorcluster, "State Machine out"=w226:refnum<class "State Machine.lvclass">)  [unwired: 7 in]
          n80 = call-dynamic "Write Return State.vi"("error in (no error)"=w229, "Return State"=w228, "State Machine in"=w226) -> ("error out"=w223:errorcluster, "State Machine out"=w225:refnum<class "State Machine.lvclass">)  [unwired: 7 in]
          n81 = call-dynamic "Write State Machine.vi"("error in (no error)"=w223, "State Machine.lvclass"=w225, "Device in"=w239) -> ("error out"=w237:errorcluster, "Device out"=w238:refnum<class "Channel.lvclass">)  [unwired: 7 in]
          n82 = call-dynamic "Read sequencias.vi"("error in (no error)"=w237, "Channel in"=w238) -> ("error out"=w231:errorcluster, "sequencias"=w235:u32, "Channel out"=w236:refnum<class "Channel.lvclass">)  [unwired: 7 in]
          n83 = Number To Decimal String(number=w235) -> (decimal integer string=w233:string)  [unwired: 1 in]
          n84 = Concatenate Strings("SET WAVEPLATE_POS " ("cmd"), w233) -> (w232:string)
          n85 = call-dynamic "Write cmd.vi"("error in (no error)"=w231, "cmd"=w232, "Device in"=w236) -> ("error out"=w240:errorcluster, "Device out"=w241:refnum<class "Channel.lvclass">)  [unwired: 7 in]
        }
        frame 8 {
          # "Verifica timeout para ACS responder.\nSe estourar timeout é porque o ACS não \nrespondeu e este canal vai para 28 para \nque o erro seja detectado em\nS4ACS_GUI:HandleObservation.vi."
          # "Compara o parametro enviado com\no parametro no Acquisition Configuration\nda msg de STATUS do ACS."
          n86 = call "Verify Timer.vi"("error in (no error)"=w255, "State Machine in"=w260) -> ("error out"=w254:errorcluster, "timeout"=w253:bool, "State Machine out"=w256:refnum<class "State Machine.lvclass">)  [unwired: 7 in]
          n87 = call-dynamic "Write State Machine.vi"("error in (no error)"=w254, "State Machine.lvclass"=w256, "Device in"=w259) -> ("error out"=w257:errorcluster, "Device out"=w258:refnum<class "Channel.lvclass">)  [unwired: 7 in]
          n88 = call-dynamic "Read resp.vi"("error in (no error)"=w257, "Device in"=w258) -> ("error out"=w245:errorcluster, "resp"=w246:string, "Device out"=w244:refnum<class "Channel.lvclass">)  [unwired: 7 in]
          n89 = Unbundle By Name(w244) -> ("Interface.lvclass"=w250:refnum<class "Interface.lvclass">)
          n90 = call-dynamic "UpdateACQconf.vi"("error in (no error)"=w245, "status"=w246, "Interface in"=w250) -> ("error out"=w242:errorcluster, "ACQ conf rx"=w249:T2)  [unwired: 6 in, 1 out]
          n91 = Unbundle By Name(w249) -> ("WAVEPLATE_POS"=w248:u32)
          n92 = Unbundle By Name(w244) -> ("sequencias"=w243:u32)
          n93 = Equal?(x=w243, y=w248) -> (x = y?=w247:bool)
          n94 = case shown="False" w253 {
            tunnel: [w262 28] -> w251
            tunnel: w252 -> [w263 _]
            tunnel: w247 -> [w261 _]
            frame False {
              n95 = case shown="True" w261 {
                tunnel: [w264 w265] -> w262
                tunnel: w263 -> [w264 w266]
                frame False {
                }
                frame True {
                  n96 = Increment(x=w266) -> (x+1=w265:i32)
                }
              }
            }
            frame True {
              # "ERRO"
            }
          }
        }
        frame 9 {
          # "Vai pra 20 validar\no ACK."
          # "Carrega timeout de 200 ciclos\npara resposta do ACS e salva\no proximo estado como estado \nde retorno."
          n97 = Increment(x=w269) -> (x+1=w275:i32)
          n98 = call-dynamic "Write Timer.vi"("error in (no error)"=w274, "Timer"=u32 200, "State Machine in"=w271) -> ("error out"=w276:errorcluster, "State Machine out"=w270:refnum<class "State Machine.lvclass">)  [unwired: 7 in]
          n99 = call-dynamic "Write Return State.vi"("error in (no error)"=w276, "Return State"=w275, "State Machine in"=w270) -> ("error out"=w273:errorcluster, "State Machine out"=w272:refnum<class "State Machine.lvclass">)  [unwired: 7 in]
          n100 = call-dynamic "Write State Machine.vi"("error in (no error)"=w273, "State Machine.lvclass"=w272, "Device in"=w280) -> ("error out"=w278:errorcluster, "Device out"=w279:refnum<class "Channel.lvclass">)  [unwired: 7 in]
          n101 = Unbundle By Name(w279) -> ("Interface.lvclass"=w286:refnum<class "Interface.lvclass">)
          n102 = call-dynamic "Read Temperature.vi"("Interface in"=w286) -> ("Temperature"=w283:i8)  [unwired: 8 in, 2 out]
          n103 = Number To Decimal String(number=w283) -> (decimal integer string=w282:string)  [unwired: 1 in]
          n104 = Concatenate Strings("SET TEMP " ("cmd"), w282) -> (w285:string)
          n105 = call-dynamic "Write cmd.vi"("error in (no error)"=w278, "cmd"=w285, "Device in"=w279) -> ("error out"=w287:errorcluster, "Device out"=w281:refnum<class "Channel.lvclass">)  [unwired: 7 in]
        }
        frame 10 {
          # "Verifica timeout para ACS responder.\nSe estourar timeout é porque o ACS não \nrespondeu e este canal vai para 28 para \nque o erro seja detectado em\nS4ACS_GUI:HandleObservation.vi."
          n106 = call "Verify Timer.vi"("error in (no error)"=w307, "State Machine in"=w304) -> ("error out"=w302:errorcluster, "timeout"=w300:bool, "State Machine out"=w303:refnum<class "State Machine.lvclass">)  [unwired: 7 in]
          n107 = call-dynamic "Write State Machine.vi"("error in (no error)"=w302, "State Machine.lvclass"=w303, "Device in"=w306) -> ("error out"=w301:errorcluster, "Device out"=w305:refnum<class "Channel.lvclass">)  [unwired: 7 in]
          n108 = call-dynamic "Read resp.vi"("error in (no error)"=w301, "Device in"=w305) -> ("error out"=w291:errorcluster, "resp"=w293:string, "Device out"=w292:refnum<class "Channel.lvclass">)  [unwired: 7 in]
          n109 = Unbundle By Name(w292) -> ("Interface.lvclass"=w299:refnum<class "Interface.lvclass">)
          n110 = call-dynamic "UpdateACQconf.vi"("error in (no error)"=w291, "status"=w293, "Interface in"=w299) -> ("error out"=w295:errorcluster, "ACQ conf rx"=w298:T2, "Interface out"=w296:refnum<class "Interface.lvclass">)  [unwired: 6 in]
          n111 = Unbundle By Name(w298) -> ("TEMP"=w289:dbl)
          n112 = call-dynamic "Read Temperature.vi"("error in (no error)"=w295, "Interface in"=w296) -> ("error out"=w290:errorcluster, "Temperature"=w294:i8)  [unwired: 7 in, 1 out]
          n113 = To Byte Integer(number=w289) -> (8bit integer=w288:i8)
          n114 = Equal?(x=w294, y=w288) -> (x = y?=w297:bool)
          n115 = case shown="False" w300 {
            tunnel: w297 -> [w312 _]
            tunnel: [w311 28 ("State")] -> w309
            tunnel: w308 -> [w310 _]
            frame False {
              n116 = case shown="True" w312 {
                tunnel: [w313 0 ("State")] -> w311
                tunnel: w310 -> [w313 _]
                frame False {
                }
                frame True {
                  # "OV 2024-04-2: Apenas seta a temperatura, pois \ncooler já está ligado. Fim do setup inicial para aquisição."
                }
              }
            }
            frame True {
              # "ERRO"
              # "Estourou timeour e ACS não recebeu\no valor da temperatura desejada.\nAborta o processo com erro de \nconfiguração"
            }
          }
        }
        frame 20 {
          w323 = "ACK" ("regular expression")
          # "Verifica timeout para o ACS responder ACK. Se estourar timeout é porque o ACS não respondeu e este canal vai para 28 para \nque o erro seja detectado em \nS4ACS_GUI:HandleObservation.vi."
          n117 = call "Verify Timer.vi"("error in (no error)"=w329, "State Machine in"=w328) -> ("error out"=w318:errorcluster, "timeout"=w327:bool, "State Machine out"=w319:refnum<class "State Machine.lvclass">)  [unwired: 7 in]
          n118 = call-dynamic "Write State Machine.vi"("error in (no error)"=w318, "State Machine.lvclass"=w319, "Device in"=w321) -> ("error out"=w317:errorcluster, "Device out"=w320:refnum<class "Channel.lvclass">)  [unwired: 7 in]
          n119 = call-dynamic "Read resp.vi"("error in (no error)"=w317, "Device in"=w320) -> ("error out"=w316:errorcluster, "resp"=w325:string, "Device out"=w322:refnum<class "Channel.lvclass">)  [unwired: 7 in]
          n120 = Match Pattern(string=w325, regular expression=w323) -> (match substring=w324:string)  [unwired: 1 in, 3 out]
          n121 = Equal?(x=w324, y=w323) -> (x = y?=w326:bool)
          n122 = case shown="False" w327 {
            tunnel: w326 -> [w334 _]
            tunnel: [w333 28 ("State")] -> w331
            tunnel: w330 -> [w332 _]
            frame False {
              n123 = case shown="True" w334 {
                tunnel: [w335 w336] -> w333
                tunnel: w332 -> [w335 w337]
                frame False {
                  # "2025.07.28: Esperando o ACK...."
                }
                frame True {
                  # "ACK recebido. Vai para proximo estado verificar se CCD_STATUS = IDLE."
                  n124 = Increment(x=w337) -> (x+1=w336:i32)
                }
              }
            }
            frame True {
              # "ERRO"
              # "225.07.28: Estourou timeout e o ACS não respondeu ACK.\nAborta o processo com erro de configuração."
            }
          }
        }
        frame 21 {
          # "Verifica timeout para o ACS responder ACK. Se estourar timeout é porque o ACS não respondeu e este canal vai para 28 para \nque o erro seja detectado em \nS4ACS_GUI:HandleObservation.vi."
          n125 = call "Verify Timer.vi"("error in (no error)"=w363, "State Machine in"=w362) -> ("error out"=w355:errorcluster, "timeout"=w361:bool, "State Machine out"=w354:refnum<class "State Machine.lvclass">)  [unwired: 7 in]
          n126 = call-dynamic "Read resp.vi"("error in (no error)"=w355, "Device in"=w356) -> ("error out"=w352:errorcluster, "resp"=w349:string, "Device out"=w353:refnum<class "Channel.lvclass">)  [unwired: 7 in]
          n127 = call-dynamic "Read Interface.vi"("error in (no error)"=w352, "Channel in"=w353) -> ("error out"=w350:errorcluster, "Interface.lvclass"=w351:refnum<class "Interface.lvclass">, "Channel out"=w346:refnum<class "Channel.lvclass">)  [unwired: 7 in]
          n128 = call-dynamic "UpdateStatus.vi"("error in (no error)"=w350, "status"=w349, "Interface in"=w351) -> ("error out"=w347:errorcluster, "Interface out"=w348:refnum<class "Interface.lvclass">)  [unwired: 7 in]
          n129 = call-dynamic "Read Acq_Status.vi"("error in (no error)"=w347, "Interface in"=w348) -> ("error out"=w344:errorcluster, "Acq_Status"=w339:string, "Interface out"=w345:refnum<class "Interface.lvclass">)  [unwired: 7 in]
          n130 = call-dynamic "Write Interface.vi"("error in (no error)"=w344, "Interface.lvclass"=w345, "Channel in"=w346) -> ("error out"=w343:errorcluster, "Channel out"=w342:refnum<class "Channel.lvclass">)  [unwired: 7 in]
          n131 = String Length(string=w339) -> (length=w341:i32)
          n132 = Greater Than 0?(x=w341) -> (x > 0?=w340:bool)
          n133 = case shown="False" w361 {
            tunnel: w340 -> [w373 _]
            tunnel: [w372 28 ("State")] -> w365
            tunnel: w364 -> [w371 _]
            tunnel: w354 -> [w370 w398]
            tunnel: [w369 w398] -> w358
            tunnel: w343 -> [w367 w397]
            tunnel: [w368 w397] -> w357
            tunnel: w339 -> [w366 _]
            frame False {
              n134 = case shown="True" w373 {
                tunnel: [w376 w383] -> w372
                tunnel: w371 -> [w376 _]
                tunnel: w370 -> [w375 w385]
                tunnel: [w375 w382] -> w369
                tunnel: [w374 w381] -> w368
                tunnel: w367 -> [w374 w384]
                tunnel: w366 -> [_ w377]
                frame False {
                  # "2025.07.28: Esperando recebimento do status do ACS."
                }
                frame True {
                  w379 = "IDLE" ("regular expression")
                  n135 = Match Pattern(string=w377, regular expression=w379) -> (match substring=w380:string)  [unwired: 1 in, 3 out]
                  n136 = Equal?(x=w380, y=w379) -> (x = y?=w378:bool)
                  n137 = case shown="True" w378 {
                    tunnel: w385 -> [w387 w393]
                    tunnel: w384 -> [w386 w392]
                    tunnel: [28 ("Return State") w391] -> w383
                    tunnel: [w387 w390] -> w382
                    tunnel: [w386 w389] -> w381
                    frame False {
                      # "ERRO"
                      # "ACS não está em repouso.\nO comando SET  foi ignorado pelo ACS:  ERRO."
                    }
                    frame True {
                      # "2025.07.28: CCD_STATUS=IDLE. Comando validado, volta\npara o estado de retorno para comparar o parâmetro enviado com o valor contido  \nno status do ACS ."
                      n138 = call-dynamic "Read Return State.vi"("error in (no error)"=w392, "State Machine in"=w393) -> ("error out"=w396:errorcluster, "Return State"=w391:i32, "State Machine out"=w395:refnum<class "State Machine.lvclass">)  [unwired: 7 in]
                      n139 = call-dynamic "Write Timer.vi"("error in (no error)"=w396, "Timer"=u32 200, "State Machine in"=w395) -> ("error out"=w389:errorcluster, "State Machine out"=w390:refnum<class "State Machine.lvclass">)  [unwired: 7 in]
                    }
                  }
                }
              }
            }
            frame True {
              # "ERRO"
              # "225.07.28: Estourou timeout e o ACS não respondeu status.\nAborta o processo com erro de configuração."
            }
          }
          n140 = call-dynamic "Write State Machine.vi"("error in (no error)"=w357, "State Machine.lvclass"=w358, "Device in"=w342) -> ("error out"=w359:errorcluster, "Device out"=w360:refnum<class "Channel.lvclass">)  [unwired: 7 in]
        }
        frame 27 {
          # "sinaliza que não está mais configurando CCD"
          # "ESTADO DE ERRO: Falha na configuração do CCD ou sufixo: vide estados  65,  300 e 301. Fica aqui só atualizando STATUS"
          # "Status.Texp = Current frame exptime\nlastStatus = cam status (acquiring, idle, writing, reading, ...)\nStatus.Nimages = frames done\nStatus.CubesDone = ciclos realizados pelo ACS\nStatus.SequesDone = sequencias realizadas pelo ACS.\nStatus.UsedDiskSpace = espaco usado no disco.\nStatus.Error = Se TRUE, houve erro na aquisção do canal."
          # "Extrair todos os parametros da respsota de STATUS e\natualizar a informação na classe Channel."
          n141 = call-dynamic "Read resp.vi"("error in (no error)"=w403, "Device in"=w402) -> ("error out"=w436:errorcluster, "resp"=w437:string, "Device out"=w440:refnum<class "Channel.lvclass">)  [unwired: 7 in]
          n142 = call-dynamic "Read Interface.vi"("error in (no error)"=w436, "Channel in"=w440) -> ("error out"=w435:errorcluster, "Interface.lvclass"=w438:refnum<class "Interface.lvclass">, "Channel out"=w439:refnum<class "Channel.lvclass">)  [unwired: 7 in]
          n143 = call-dynamic "UpdateStatus.vi"("error in (no error)"=w435, "status"=w437, "Interface in"=w438) -> ("error out"=w407:errorcluster, "Interface out"=w409:refnum<class "Interface.lvclass">)  [unwired: 7 in]
          n144 = call-dynamic "Read Error.vi"("error in (no error)"=w407, "Interface in"=w409) -> ("error out"=w406:errorcluster, "Error"=w405:bool, "Interface out"=w408:refnum<class "Interface.lvclass">)  [unwired: 7 in]
          n145 = call-dynamic "Read Exposições realizadas.vi"("error in (no error)"=w406, "Interface in"=w408) -> ("error out"=w423:errorcluster, "Exposições realizadas"=w424:dbl, "Interface out"=w425:refnum<class "Interface.lvclass">)  [unwired: 7 in]
          n146 = call-dynamic "Read Cam_Status.vi"("error in (no error)"=w423, "Interface in"=w425) -> ("error out"=w432:errorcluster, "Cam_Status"=w421:string, "Interface out"=w434:refnum<class "Interface.lvclass">)  [unwired: 7 in]
          n147 = call-dynamic "Read %Acquired.vi"("error in (no error)"=w432, "Interface in"=w434) -> ("error out"=w431:errorcluster, "% Acquired"=w428:dbl, "Interface out"=w433:refnum<class "Interface.lvclass">)  [unwired: 7 in]
          n148 = call "Read Exposure Time.vi"("error in (no error)"=w431, "Interface in"=w433) -> ("error out"=w419:errorcluster, "Exposure Time"=w430:dbl, "Interface out"=w420:refnum<class "Interface.lvclass">)  [unwired: 7 in]
          n149 = call-dynamic "Read Number of Cycles.vi"("error in (no error)"=w419, "Interface in"=w420) -> ("error out"=w416:errorcluster, "Number of Cycles"=w418:u32, "Interface out"=w417:refnum<class "Interface.lvclass">)  [unwired: 7 in]
          n150 = call-dynamic "Read Number of Sequences.vi"("error in (no error)"=w416, "Interface in"=w417) -> ("error out"=w412:errorcluster, "Number of Sequences"=w415:u32, "Interface out"=w414:refnum<class "Interface.lvclass">)  [unwired: 7 in]
          n151 = call-dynamic "Read Ocupacao do disco.vi"("error in (no error)"=w412, "Interface in"=w414) -> ("error out"=w411:errorcluster, "Ocupacao do disco"=w410:u16, "Interface out"=w413:refnum<class "Interface.lvclass">)  [unwired: 7 in]
          n152 = call-dynamic "Write Interface.vi"("error in (no error)"=w411, "Interface.lvclass"=w413, "Channel in"=w439) -> ("error out"=w400:errorcluster, "Channel out"=w401:refnum<class "Channel.lvclass">)  [unwired: 7 in]
          n153 = Divide(x=w428, y=100.0) -> (x/y=w426:dbl)
          n154 = To Unsigned Long Integer(number=w424) -> (unsigned 32bit integer=w422:u32)
          n155 = Multiply(x=w430, y=w426) -> (x*y=w429:dbl)
          n156 = Bundle By Name(cluster=w401, "Texp"=w429, "lastStatus"=w421, "Nimages"=w422, "CyclesDone"=w418, "SequesDone"=w415, "UsedDiskSpace"=w410, "Error"=w405, "config"=FALSE) -> (w441:refnum<class "Channel.lvclass">)
        }
        frame 28 {
          # "ESTADO DE ERRO: Fica aqui ATUALIZANDO STATUS até que S4GUI:HandleObservationSync.vi ou S4GUI:HandleObservationAsync.vi ou os botões START, STOP, ABORT mandem para outro estado."
          # "sinaliza que não está mais configurando CCD"
          # "Status.Texp = Current frame exptime\nlastStatus = cam status (acquiring, idle, writing, reading, ...)\nStatus.Nimages = frames done\nStatus.CubesDone = ciclos realizados pelo ACS\nStatus.SequesDone = sequencias realizadas pelo ACS.\nStatus.UsedDiskSpace = espaco usado no disco.\nStatus.Error = Se TRUE, houve erro na aquisção do canal."
          # "Extrair todos os parametros da respsota de STATUS e\natualizar a informação na classe Channel."
          n157 = call-dynamic "Read resp.vi"("error in (no error)"=w446, "Device in"=w445) -> ("error out"=w479:errorcluster, "resp"=w480:string, "Device out"=w483:refnum<class "Channel.lvclass">)  [unwired: 7 in]
          n158 = call-dynamic "Read Interface.vi"("error in (no error)"=w479, "Channel in"=w483) -> ("error out"=w478:errorcluster, "Interface.lvclass"=w481:refnum<class "Interface.lvclass">, "Channel out"=w482:refnum<class "Channel.lvclass">)  [unwired: 7 in]
          n159 = call-dynamic "UpdateStatus.vi"("error in (no error)"=w478, "status"=w480, "Interface in"=w481) -> ("error out"=w450:errorcluster, "Interface out"=w452:refnum<class "Interface.lvclass">)  [unwired: 7 in]
          n160 = call-dynamic "Read Error.vi"("error in (no error)"=w450, "Interface in"=w452) -> ("error out"=w449:errorcluster, "Error"=w448:bool, "Interface out"=w451:refnum<class "Interface.lvclass">)  [unwired: 7 in]
          n161 = call-dynamic "Read Exposições realizadas.vi"("error in (no error)"=w449, "Interface in"=w451) -> ("error out"=w466:errorcluster, "Exposições realizadas"=w467:dbl, "Interface out"=w468:refnum<class "Interface.lvclass">)  [unwired: 7 in]
          n162 = call-dynamic "Read Cam_Status.vi"("error in (no error)"=w466, "Interface in"=w468) -> ("error out"=w475:errorcluster, "Cam_Status"=w464:string, "Interface out"=w477:refnum<class "Interface.lvclass">)  [unwired: 7 in]
          n163 = call-dynamic "Read %Acquired.vi"("error in (no error)"=w475, "Interface in"=w477) -> ("error out"=w474:errorcluster, "% Acquired"=w471:dbl, "Interface out"=w476:refnum<class "Interface.lvclass">)  [unwired: 7 in]
          n164 = call "Read Exposure Time.vi"("error in (no error)"=w474, "Interface in"=w476) -> ("error out"=w462:errorcluster, "Exposure Time"=w473:dbl, "Interface out"=w463:refnum<class "Interface.lvclass">)  [unwired: 7 in]
          n165 = call-dynamic "Read Number of Cycles.vi"("error in (no error)"=w462, "Interface in"=w463) -> ("error out"=w459:errorcluster, "Number of Cycles"=w461:u32, "Interface out"=w460:refnum<class "Interface.lvclass">)  [unwired: 7 in]
          n166 = call-dynamic "Read Number of Sequences.vi"("error in (no error)"=w459, "Interface in"=w460) -> ("error out"=w455:errorcluster, "Number of Sequences"=w458:u32, "Interface out"=w457:refnum<class "Interface.lvclass">)  [unwired: 7 in]
          n167 = call-dynamic "Read Ocupacao do disco.vi"("error in (no error)"=w455, "Interface in"=w457) -> ("error out"=w454:errorcluster, "Ocupacao do disco"=w453:u16, "Interface out"=w456:refnum<class "Interface.lvclass">)  [unwired: 7 in]
          n168 = call-dynamic "Write Interface.vi"("error in (no error)"=w454, "Interface.lvclass"=w456, "Channel in"=w482) -> ("error out"=w443:errorcluster, "Channel out"=w444:refnum<class "Channel.lvclass">)  [unwired: 7 in]
          n169 = Divide(x=w471, y=100.0) -> (x/y=w469:dbl)
          n170 = To Unsigned Long Integer(number=w467) -> (unsigned 32bit integer=w465:u32)
          n171 = Multiply(x=w473, y=w469) -> (x*y=w472:dbl)
          n172 = Bundle By Name(cluster=w444, "Texp"=w472, "lastStatus"=w464, "Nimages"=w465, "CyclesDone"=w461, "SequesDone"=w458, "UsedDiskSpace"=w453, "Error"=w448, "config"=FALSE) -> (w484:refnum<class "Channel.lvclass">)
        }
        frame 29 {
          # "ESTADO DE ERRO:  Exp Time inválido! Fica parado aqui só ATUALZIANDO STATUS"
          # "sinaliza que não está mais configurando CCD"
          # "Status.Texp = Current frame exptime\nlastStatus = cam status (acquiring, idle, writing, reading, ...)\nStatus.Nimages = frames done\nStatus.CubesDone = ciclos realizados pelo ACS\nStatus.SequesDone = sequencias realizadas pelo ACS.\nStatus.UsedDiskSpace = espaco usado no disco.\nStatus.Error = Se TRUE, houve erro na aquisção do canal."
          # "Extrair todos os parametros da respsota de STATUS e\natualizar a informação na classe Channel."
          n173 = call-dynamic "Read resp.vi"("error in (no error)"=w489, "Device in"=w488) -> ("error out"=w522:errorcluster, "resp"=w523:string, "Device out"=w526:refnum<class "Channel.lvclass">)  [unwired: 7 in]
          n174 = call-dynamic "Read Interface.vi"("error in (no error)"=w522, "Channel in"=w526) -> ("error out"=w521:errorcluster, "Interface.lvclass"=w524:refnum<class "Interface.lvclass">, "Channel out"=w525:refnum<class "Channel.lvclass">)  [unwired: 7 in]
          n175 = call-dynamic "UpdateStatus.vi"("error in (no error)"=w521, "status"=w523, "Interface in"=w524) -> ("error out"=w493:errorcluster, "Interface out"=w495:refnum<class "Interface.lvclass">)  [unwired: 7 in]
          n176 = call-dynamic "Read Error.vi"("error in (no error)"=w493, "Interface in"=w495) -> ("error out"=w492:errorcluster, "Error"=w491:bool, "Interface out"=w494:refnum<class "Interface.lvclass">)  [unwired: 7 in]
          n177 = call-dynamic "Read Exposições realizadas.vi"("error in (no error)"=w492, "Interface in"=w494) -> ("error out"=w509:errorcluster, "Exposições realizadas"=w510:dbl, "Interface out"=w511:refnum<class "Interface.lvclass">)  [unwired: 7 in]
          n178 = call-dynamic "Read Cam_Status.vi"("error in (no error)"=w509, "Interface in"=w511) -> ("error out"=w518:errorcluster, "Cam_Status"=w507:string, "Interface out"=w520:refnum<class "Interface.lvclass">)  [unwired: 7 in]
          n179 = call-dynamic "Read %Acquired.vi"("error in (no error)"=w518, "Interface in"=w520) -> ("error out"=w517:errorcluster, "% Acquired"=w514:dbl, "Interface out"=w519:refnum<class "Interface.lvclass">)  [unwired: 7 in]
          n180 = call "Read Exposure Time.vi"("error in (no error)"=w517, "Interface in"=w519) -> ("error out"=w505:errorcluster, "Exposure Time"=w516:dbl, "Interface out"=w506:refnum<class "Interface.lvclass">)  [unwired: 7 in]
          n181 = call-dynamic "Read Number of Cycles.vi"("error in (no error)"=w505, "Interface in"=w506) -> ("error out"=w502:errorcluster, "Number of Cycles"=w504:u32, "Interface out"=w503:refnum<class "Interface.lvclass">)  [unwired: 7 in]
          n182 = call-dynamic "Read Number of Sequences.vi"("error in (no error)"=w502, "Interface in"=w503) -> ("error out"=w498:errorcluster, "Number of Sequences"=w501:u32, "Interface out"=w500:refnum<class "Interface.lvclass">)  [unwired: 7 in]
          n183 = call-dynamic "Read Ocupacao do disco.vi"("error in (no error)"=w498, "Interface in"=w500) -> ("error out"=w497:errorcluster, "Ocupacao do disco"=w496:u16, "Interface out"=w499:refnum<class "Interface.lvclass">)  [unwired: 7 in]
          n184 = call-dynamic "Write Interface.vi"("error in (no error)"=w497, "Interface.lvclass"=w499, "Channel in"=w525) -> ("error out"=w486:errorcluster, "Channel out"=w487:refnum<class "Channel.lvclass">)  [unwired: 7 in]
          n185 = Divide(x=w514, y=100.0) -> (x/y=w512:dbl)
          n186 = To Unsigned Long Integer(number=w510) -> (unsigned 32bit integer=w508:u32)
          n187 = Multiply(x=w516, y=w512) -> (x*y=w515:dbl)
          n188 = Bundle By Name(cluster=w487, "Texp"=w515, "lastStatus"=w507, "Nimages"=w508, "CyclesDone"=w504, "SequesDone"=w501, "UsedDiskSpace"=w496, "Error"=w491, "config"=FALSE) -> (w527:refnum<class "Channel.lvclass">)
        }
        frame 30 {
          # "OV20241125: Valor de COOLER é o target:\nSe =1  manda ligar,\nSe =0  manda desligar."
          n189 = call-dynamic "Write Timer.vi"("error in (no error)"=w535, "Timer"=u32 50, "State Machine in"=w537) -> ("error out"=w534:errorcluster, "State Machine out"=w536:refnum<class "State Machine.lvclass">)  [unwired: 7 in]
          n190 = call-dynamic "Write State Machine.vi"("error in (no error)"=w534, "State Machine.lvclass"=w536, "Device in"=w538) -> ("error out"=w533:errorcluster, "Device out"=w531:refnum<class "Channel.lvclass">)  [unwired: 7 in]
          n191 = Bundle By Name(cluster=w531, "config"=TRUE) -> (w530:refnum<class "Channel.lvclass">)
          n192 = Unbundle By Name(w530) -> ("Interface.lvclass"=w546:refnum<class "Interface.lvclass">)
          n193 = call-dynamic "Read Cooler ON_OFF.vi"("error in (no error)"=w533, "Interface in"=w546) -> ("error out"=w532:errorcluster, "Cooler ON/OFF"=w541:i16)  [unwired: 7 in, 1 out]
          n194 = case shown="0" w541 {
            tunnel: ["0" "1"] -> w540
            frame 0 {
              (unwired) "OFF"
            }
            frame 1, Default {
              (unwired) "ON"
            }
          }
          n195 = Concatenate Strings("SET COOLER_POWER_STATUS " ("cmd"), w540) -> (w545:string)
          n196 = call-dynamic "Write cmd.vi"("error in (no error)"=w532, "cmd"=w545, "Device in"=w530) -> ("error out"=w547:errorcluster, "Device out"=w548:refnum<class "Channel.lvclass">)  [unwired: 7 in]
          n197 = Increment(x=w543) -> (x+1=w544:i32)
        }
        frame 31 {
          n198 = call "Verify Timer.vi"("error in (no error)"=w570, "State Machine in"=w567) -> ("error out"=w565:errorcluster, "timeout"=w563:bool, "State Machine out"=w566:refnum<class "State Machine.lvclass">)  [unwired: 7 in]
          n199 = call-dynamic "Write State Machine.vi"("error in (no error)"=w565, "State Machine.lvclass"=w566, "Device in"=w569) -> ("error out"=w564:errorcluster, "Device out"=w568:refnum<class "Channel.lvclass">)  [unwired: 7 in]
          n200 = call-dynamic "Read resp.vi"("error in (no error)"=w564, "Device in"=w568) -> ("error out"=w553:errorcluster, "resp"=w554:string, "Device out"=w552:refnum<class "Channel.lvclass">)  [unwired: 7 in]
          n201 = Unbundle By Name(w552) -> ("Interface.lvclass"=w562:refnum<class "Interface.lvclass">)
          n202 = call-dynamic "UpdateACQconf.vi"("error in (no error)"=w553, "status"=w554, "Interface in"=w562) -> ("error out"=w559:errorcluster, "ACQ conf rx"=w561:T2, "Interface out"=w560:refnum<class "Interface.lvclass">)  [unwired: 6 in]
          n203 = Unbundle By Name(w561) -> ("COOLER_POWER_STATUS"=w557:dbl)
          n204 = call-dynamic "Read Cooler ON_OFF.vi"("error in (no error)"=w559, "Interface in"=w560) -> ("error out"=w551:errorcluster, "Cooler ON/OFF"=w558:i16)  [unwired: 7 in, 1 out]
          n205 = To Word Integer(number=w557) -> (16bit integer=w556:i16)
          n206 = Equal?(x=w558, y=w556) -> (x = y?=w555:bool)
          n207 = case shown="False" w563 {
            tunnel: w555 -> [w575 _]
            tunnel: [w574 w578] -> w572
            tunnel: w571 -> [w573 _]
            frame False {
              n208 = case shown="True" w575 {
                tunnel: [w576 0 ("State")] -> w574
                tunnel: w573 -> [w576 _]
                frame False {
                }
                frame True {
                }
              }
            }
            frame True {
              n209 = disable-structure shown="Enabled" {
                disable-tunnel: [0 ("State") 28 ("State")] -> w578
                frame Disabled {
                }
                frame Enabled {
                  # "erro"
                }
              }
            }
          }
        }
        frame 32 {
          # "Este estado não é mais usado!!"
          n210 = call-dynamic "Write Timer.vi"("error in (no error)"=w585, "Timer"=u32 50, "State Machine in"=w586) -> ("error out"=w588:errorcluster, "State Machine out"=w583:refnum<class "State Machine.lvclass">)  [unwired: 7 in]
          n211 = call-dynamic "Write State Machine.vi"("error in (no error)"=w588, "State Machine.lvclass"=w583, "Device in"=w587) -> ("error out"=w581:errorcluster, "Device out"=w582:refnum<class "Channel.lvclass">)  [unwired: 7 in]
          n212 = call-dynamic "Write cmd.vi"("error in (no error)"=w581, "cmd"="GET COOLER_POWER_STATUS ", "Device in"=w582) -> ("error out"=w592:errorcluster, "Device out"=w593:refnum<class "Channel.lvclass">)  [unwired: 7 in]
          n213 = Increment(x=w590) -> (x+1=w591:i32)
        }
        frame 33 {
          # "Este estado não é mais usado!!"
          n214 = call "Verify Timer.vi"("error in (no error)"=w597, "State Machine in"=w601) -> ("error out"=w596:errorcluster, "timeout"=w595:bool, "State Machine out"=w598:refnum<class "State Machine.lvclass">)  [unwired: 7 in]
          n215 = call-dynamic "Write State Machine.vi"("error in (no error)"=w596, "State Machine.lvclass"=w598, "Device in"=w600) -> ("error out"=w594:errorcluster, "Device out"=w599:refnum<class "Channel.lvclass">)  [unwired: 7 in]
          n216 = call-dynamic "Read resp.vi"("error in (no error)"=w594, "Device in"=w599) -> ("error out"=w606:errorcluster, "resp"=w602:string, "Device out"=w607:refnum<class "Channel.lvclass">)  [unwired: 7 in]
          n217 = case shown="False" w595 {
            tunnel: [w615 w636] -> w608
            tunnel: w607 -> [w614 w636]
            tunnel: w606 -> [w613 w635]
            tunnel: [w612 w635] -> w605
            tunnel: [w611 w634] -> w604
            tunnel: w603 -> [w610 _]
            tunnel: w602 -> [w609 _]
            frame False {
              n218 = case shown="\"0\", \"1\"" w609 {
                selector: w609 -> [_ w627]
                tunnel: [w618 w623] -> w615
                tunnel: w614 -> [w618 w631]
                tunnel: w613 -> [w617 w629]
                tunnel: [w617 w621] -> w612
                tunnel: [w616 w628] -> w611
                tunnel: w610 -> [w616 _]
                frame Default {
                }
                frame "0", "1" {
                  n219 = Decimal String To Number(string=w627) -> (number=w626:i32)  [unwired: 2 in, 1 out]
                  n220 = Unbundle By Name(w631) -> ("Interface.lvclass"=w630:refnum<class "Interface.lvclass">)
                  n221 = To Word Integer(number=w626) -> (16bit integer=w625:i16)
                  n222 = call-dynamic "Write Cooler ON_OFF.vi"("error in (no error)"=w629, "Cooler ON/OFF"=w625, "Interface in"=w630) -> ("error out"=w622:errorcluster, "Interface out"=w620:refnum<class "Interface.lvclass">)  [unwired: 7 in]
                  n223 = Bundle By Name(cluster=w631, "Interface.lvclass"=w620) -> (w624:refnum<class "Channel.lvclass">)
                  n224 = disable-structure shown="Enabled" {
                    disable-tunnel: [0 ("State") 45 ("State")] -> w628
                    frame Disabled {
                    }
                    frame Enabled {
                      (unwired) 300 ("State")
                      # "40: configura os\nparametros por comando\nSET TEXP e WAIT EXPOSE"
                    }
                  }
                  n225 = call-dynamic "Save Temp.vi"("error in (no error)"=w622, "temp file"="lasttemp.cfg", "Channel in"=w624) -> ("error out"=w621:errorcluster, "Channel out"=w623:refnum<class "Channel.lvclass">)  [unwired: 7 in]
                }
              }
            }
            frame True {
              n226 = disable-structure shown="Enabled" {
                disable-tunnel: [0 ("State") 45 ("State")] -> w634
                frame Disabled {
                }
                frame Enabled {
                  (unwired) 300 ("State")
                  # "45: configura os\nparametros por comando\nSET TEXP e WAIT EXPOSE"
                }
              }
            }
          }
        }
        frame 35 {
          # "Carrega timeout de 50 ciclos\n50 x 20ms = 1s\npara resposta do ACS"
          n227 = call-dynamic "Write Timer.vi"("error in (no error)"=w647, "Timer"=u32 50, "State Machine in"=w645) -> ("error out"=w643:errorcluster, "State Machine out"=w644:refnum<class "State Machine.lvclass">)  [unwired: 7 in]
          n228 = call-dynamic "Write State Machine.vi"("error in (no error)"=w643, "State Machine.lvclass"=w644, "Device in"=w646) -> ("error out"=w642:errorcluster, "Device out"=w641:refnum<class "Channel.lvclass">)  [unwired: 7 in]
          n229 = Bundle By Name(cluster=w641, "config"=TRUE) -> (w640:refnum<class "Channel.lvclass">)
          n230 = Unbundle By Name(w640) -> ("Interface.lvclass"=w656:refnum<class "Interface.lvclass">)
          n231 = call-dynamic "Read Temperature.vi"("Interface in"=w656) -> ("Temperature"=w653:i8)  [unwired: 8 in, 2 out]
          n232 = Number To Decimal String(number=w653) -> (decimal integer string=w652:string)  [unwired: 1 in]
          n233 = Concatenate Strings("SET TEMP " ("cmd"), w652) -> (w655:string)
          n234 = call-dynamic "Write cmd.vi"("error in (no error)"=w642, "cmd"=w655, "Device in"=w640) -> ("error out"=w657:errorcluster, "Device out"=w650:refnum<class "Channel.lvclass">)  [unwired: 7 in]
          n235 = Increment(x=w649) -> (x+1=w651:i32)
        }
        frame 36 {
          n236 = call "Verify Timer.vi"("error in (no error)"=w677, "State Machine in"=w674) -> ("error out"=w672:errorcluster, "timeout"=w670:bool, "State Machine out"=w673:refnum<class "State Machine.lvclass">)  [unwired: 7 in]
          n237 = call-dynamic "Write State Machine.vi"("error in (no error)"=w672, "State Machine.lvclass"=w673, "Device in"=w676) -> ("error out"=w671:errorcluster, "Device out"=w675:refnum<class "Channel.lvclass">)  [unwired: 7 in]
          n238 = call-dynamic "Read resp.vi"("error in (no error)"=w671, "Device in"=w675) -> ("error out"=w661:errorcluster, "resp"=w663:string, "Device out"=w662:refnum<class "Channel.lvclass">)  [unwired: 7 in]
          n239 = Unbundle By Name(w662) -> ("Interface.lvclass"=w669:refnum<class "Interface.lvclass">)
          n240 = call-dynamic "UpdateACQconf.vi"("error in (no error)"=w661, "status"=w663, "Interface in"=w669) -> ("error out"=w665:errorcluster, "ACQ conf rx"=w668:T2, "Interface out"=w666:refnum<class "Interface.lvclass">)  [unwired: 6 in]
          n241 = Unbundle By Name(w668) -> ("TEMP"=w659:dbl)
          n242 = call-dynamic "Read Temperature.vi"("error in (no error)"=w665, "Interface in"=w666) -> ("error out"=w660:errorcluster, "Temperature"=w664:i8)  [unwired: 7 in, 1 out]
          n243 = To Byte Integer(number=w659) -> (8bit integer=w658:i8)
          n244 = Equal?(x=w664, y=w658) -> (x = y?=w667:bool)
          n245 = case shown="False" w670 {
            tunnel: w667 -> [w682 _]
            tunnel: [w681 w689] -> w679
            tunnel: w678 -> [w680 _]
            frame False {
              n246 = case shown="True" w682 {
                tunnel: [w683 w684] -> w681
                tunnel: w680 -> [w683 w685]
                frame False {
                }
                frame True {
                  # "OV 2022-11-16: Ao setar a temperatura, liga \nautomaticamente o COLLER."
                  n247 = disable-structure shown="Enabled" {
                    disable-tunnel: w685 -> [w687 _]
                    disable-tunnel: [w686 0] -> w684
                    frame Disabled {
                      n248 = Increment(x=w687) -> (x+1=w686:i32)
                    }
                    frame Enabled {
                    }
                  }
                }
              }
            }
            frame True {
              n249 = disable-structure shown="Enabled" {
                disable-tunnel: [0 ("State") 28 ("State")] -> w689
                frame Disabled {
                }
                frame Enabled {
                  (unwired) 300 ("State")
                  (unwired) 45 ("State")
                  # "erro"
                  # "45: configura os\nparametros por comando\nSET SUFFIX e\nWAIT_EXPOSE_COMMAND"
                }
              }
            }
          }
        }
        frame 37 {
          w696 = i16 1 items=["Cooler OFF", "Cooler ON"] ("Cooler ON/OFF")
          # "Liga COOLER"
          n250 = call-dynamic "Write Timer.vi"("error in (no error)"=w702, "Timer"=u32 50, "State Machine in"=w704) -> ("error out"=w701:errorcluster, "State Machine out"=w703:refnum<class "State Machine.lvclass">)  [unwired: 7 in]
          n251 = call-dynamic "Write State Machine.vi"("error in (no error)"=w701, "State Machine.lvclass"=w703, "Device in"=w705) -> ("error out"=w697:errorcluster, "Device out"=w694:refnum<class "Channel.lvclass">)  [unwired: 7 in]
          n252 = Unbundle By Name(w694) -> ("Interface.lvclass"=w698:refnum<class "Interface.lvclass">)
          n253 = call-dynamic "Write Cooler ON_OFF.vi"("error in (no error)"=w697, "Cooler ON/OFF"=w696, "Interface in"=w698) -> ("error out"=w695:errorcluster, "Interface out"=w693:refnum<class "Interface.lvclass">)  [unwired: 7 in]
          n254 = Bundle By Name(cluster=w694, "Interface.lvclass"=w693) -> (w692:refnum<class "Channel.lvclass">)
          n255 = call-dynamic "Write cmd.vi"("error in (no error)"=w695, "cmd"="SET COOLER_POWER_STATUS 1", "Device in"=w692) -> ("error out"=w707:errorcluster, "Device out"=w708:refnum<class "Channel.lvclass">)  [unwired: 7 in]
        }
        frame 38 {
          # "ESTADO DE ERRO: Texp incompativel com a configuração do CCD (vem do estado 1 quando Valid Conf? retorna false) ;\nFica aqui até que S4GUI:HandleObservationSync.vi ou S4GUI:HandleObservationAsync.vi ou os botões START, STOP, ABORT mandem para outro estado."
          # "sinaliza que não está mais configurando CCD"
          # "Status.Texp = Current frame exptime\nlastStatus = cam status (acquiring, idle, writing, reading, ...)\nStatus.Nimages = frames done\nStatus.CubesDone = ciclos realizados pelo ACS\nStatus.SequesDone = sequencias realizadas pelo ACS.\nStatus.UsedDiskSpace = espaco usado no disco.\nStatus.Error = Se TRUE, houve erro na aquisção do canal."
          # "Extrair todos os parametros da respsota de STATUS e\natualizar a informação na classe Channel."
          n256 = call-dynamic "Read resp.vi"("error in (no error)"=w712, "Device in"=w711) -> ("error out"=w745:errorcluster, "resp"=w746:string, "Device out"=w749:refnum<class "Channel.lvclass">)  [unwired: 7 in]
          n257 = call-dynamic "Read Interface.vi"("error in (no error)"=w745, "Channel in"=w749) -> ("error out"=w744:errorcluster, "Interface.lvclass"=w747:refnum<class "Interface.lvclass">, "Channel out"=w748:refnum<class "Channel.lvclass">)  [unwired: 7 in]
          n258 = call-dynamic "UpdateStatus.vi"("error in (no error)"=w744, "status"=w746, "Interface in"=w747) -> ("error out"=w716:errorcluster, "Interface out"=w718:refnum<class "Interface.lvclass">)  [unwired: 7 in]
          n259 = call-dynamic "Read Error.vi"("error in (no error)"=w716, "Interface in"=w718) -> ("error out"=w715:errorcluster, "Error"=w714:bool, "Interface out"=w717:refnum<class "Interface.lvclass">)  [unwired: 7 in]
          n260 = call-dynamic "Read Exposições realizadas.vi"("error in (no error)"=w715, "Interface in"=w717) -> ("error out"=w732:errorcluster, "Exposições realizadas"=w733:dbl, "Interface out"=w734:refnum<class "Interface.lvclass">)  [unwired: 7 in]
          n261 = call-dynamic "Read Cam_Status.vi"("error in (no error)"=w732, "Interface in"=w734) -> ("error out"=w741:errorcluster, "Cam_Status"=w730:string, "Interface out"=w743:refnum<class "Interface.lvclass">)  [unwired: 7 in]
          n262 = call-dynamic "Read %Acquired.vi"("error in (no error)"=w741, "Interface in"=w743) -> ("error out"=w740:errorcluster, "% Acquired"=w737:dbl, "Interface out"=w742:refnum<class "Interface.lvclass">)  [unwired: 7 in]
          n263 = call "Read Exposure Time.vi"("error in (no error)"=w740, "Interface in"=w742) -> ("error out"=w728:errorcluster, "Exposure Time"=w739:dbl, "Interface out"=w729:refnum<class "Interface.lvclass">)  [unwired: 7 in]
          n264 = call-dynamic "Read Number of Cycles.vi"("error in (no error)"=w728, "Interface in"=w729) -> ("error out"=w725:errorcluster, "Number of Cycles"=w727:u32, "Interface out"=w726:refnum<class "Interface.lvclass">)  [unwired: 7 in]
          n265 = call-dynamic "Read Number of Sequences.vi"("error in (no error)"=w725, "Interface in"=w726) -> ("error out"=w721:errorcluster, "Number of Sequences"=w724:u32, "Interface out"=w723:refnum<class "Interface.lvclass">)  [unwired: 7 in]
          n266 = call-dynamic "Read Ocupacao do disco.vi"("error in (no error)"=w721, "Interface in"=w723) -> ("error out"=w720:errorcluster, "Ocupacao do disco"=w719:u16, "Interface out"=w722:refnum<class "Interface.lvclass">)  [unwired: 7 in]
          n267 = call-dynamic "Write Interface.vi"("error in (no error)"=w720, "Interface.lvclass"=w722, "Channel in"=w748) -> ("error out"=w709:errorcluster, "Channel out"=w710:refnum<class "Channel.lvclass">)  [unwired: 7 in]
          n268 = Divide(x=w737, y=100.0) -> (x/y=w735:dbl)
          n269 = To Unsigned Long Integer(number=w733) -> (unsigned 32bit integer=w731:u32)
          n270 = Multiply(x=w739, y=w735) -> (x*y=w738:dbl)
          n271 = Bundle By Name(cluster=w710, "Texp"=w738, "lastStatus"=w730, "Nimages"=w731, "CyclesDone"=w727, "SequesDone"=w724, "UsedDiskSpace"=w719, "Error"=w714, "config"=FALSE) -> (w750:refnum<class "Channel.lvclass">)
        }
        frame 40 {
          n272 = disable-structure shown="Disabled" {
            disable-tunnel: [w776 w778] -> w768
            disable-tunnel: w767 -> [w774 w778]
            disable-tunnel: w765 -> [w773 w777]
            disable-tunnel: [w772 w777] -> w764
            frame Disabled {
              # "Carrega timeout de 10 ciclos\npara resposta do ACS"
              n273 = call-dynamic "Write Timer.vi"("error in (no error)"=w773, "Timer"=u32 10, "State Machine in"=w774) -> ("error out"=w772:errorcluster, "State Machine out"=w776:refnum<class "State Machine.lvclass">)  [unwired: 7 in]
            }
            frame Enabled {
            }
          }
          n274 = call-dynamic "Write State Machine.vi"("error in (no error)"=w764, "State Machine.lvclass"=w768, "Device in"=w766) -> ("error out"=w763:errorcluster, "Device out"=w754:refnum<class "Channel.lvclass">)  [unwired: 7 in]
          n275 = Bundle By Name(cluster=w754, "config"=TRUE) -> (w753:refnum<class "Channel.lvclass">)
          n276 = Unbundle By Name(w753) -> ("wait_expose"=w760:bool)
          n277 = Select(t="ON", s=w760, f="OFF") -> (s? t:f=w757:string)
          n278 = Concatenate Strings("WAIT_EXPOSE_COMMAND " ("cmd"), w757) -> (w756:string)
          n279 = call-dynamic "Write cmd.vi"("error in (no error)"=w763, "cmd"=w756, "Device in"=w753) -> ("error out"=w769:errorcluster, "Device out"=w755:refnum<class "Channel.lvclass">)  [unwired: 7 in]
          n280 = disable-structure shown="Enabled" {
            disable-tunnel: [0 ("State") 45 ("State")] -> w762
            frame Enabled {
            }
            frame Disabled {
              # "Termina o processo, \nconfigurando a Texp \ndos canais."
            }
          }
        }
        frame 45 {
          # "Carrega timeout de 200 ciclos\npara resposta do ACS"
          n281 = call-dynamic "Write Timer.vi"("error in (no error)"=w789, "Timer"=u32 200, "State Machine in"=w788) -> ("error out"=w784:errorcluster, "State Machine out"=w786:refnum<class "State Machine.lvclass">)  [unwired: 7 in]
          n282 = call-dynamic "Write State Machine.vi"("error in (no error)"=w784, "State Machine.lvclass"=w786, "Device in"=w787) -> ("error out"=w782:errorcluster, "Device out"=w783:refnum<class "Channel.lvclass">)  [unwired: 7 in]
          n283 = call-dynamic "ValidateConfig.vi"("error in (no error)"=w782, "Channel in"=w783) -> ("error out"=w780:errorcluster, "valid?"=w779:bool, "Channel out"=w781:refnum<class "Channel.lvclass">)  [unwired: 7 in]
          n284 = case shown="True" w779 {
            tunnel: [w796 w810] -> w793
            tunnel: [w795 w809] -> w792
            tunnel: [29 w808] -> w791
            tunnel: w790 -> [_ w807]
            tunnel: w781 -> [w796 w799]
            tunnel: w780 -> [w795 w800]
            frame False {
              # "Erro!"
            }
            frame True {
              n285 = Bundle By Name(cluster=w799, "config"=TRUE) -> (w798:refnum<class "Channel.lvclass">)
              n286 = Unbundle By Name(w798) -> ("Interface.lvclass"=w806:refnum<class "Interface.lvclass">)
              n287 = call "Read Exposure Time.vi"("Interface in"=w806) -> ("Exposure Time"=w805:dbl)  [unwired: 8 in, 2 out]
              n288 = Number To Fractional String(use system decimal point (T)=FALSE, number=w805) -> (F-format string=w804:string)  [unwired: 2 in]
              n289 = Concatenate Strings("SET EXPTIME " ("cmd"), w804) -> (w803:string)
              n290 = Increment(x=w807) -> (x+1=w808:i32)
              n291 = call-dynamic "Write cmd.vi"("error in (no error)"=w800, "cmd"=w803, "Device in"=w798) -> ("error out"=w809:errorcluster, "Device out"=w810:refnum<class "Channel.lvclass">)  [unwired: 7 in]
            }
          }
        }
        frame 46 {
          # "Compara o parametro enviado com\no parametro no Acquisition Configuration\nda msg de STATUS do ACS."
          # "Verifica timeout para ACS responder.\nSe estourar timeout é porque o ACS não \nrespondeu e este canal vai para 28 para \nque o erro seja detectado em\nS4ACS_GUI:HandleObservation.vi."
          n292 = call "Verify Timer.vi"("error in (no error)"=w828, "State Machine in"=w830) -> ("error out"=w827:errorcluster, "timeout"=w825:bool, "State Machine out"=w829:refnum<class "State Machine.lvclass">)  [unwired: 7 in]
          n293 = call-dynamic "Write State Machine.vi"("error in (no error)"=w827, "State Machine.lvclass"=w829, "Device in"=w831) -> ("error out"=w826:errorcluster, "Device out"=w822:refnum<class "Channel.lvclass">)  [unwired: 7 in]
          n294 = call-dynamic "Read resp.vi"("error in (no error)"=w826, "Device in"=w822) -> ("error out"=w813:errorcluster, "resp"=w821:string, "Device out"=w820:refnum<class "Channel.lvclass">)  [unwired: 7 in]
          n295 = Unbundle By Name(w820) -> ("Interface.lvclass"=w819:refnum<class "Interface.lvclass">)
          n296 = call-dynamic "UpdateACQconf.vi"("error in (no error)"=w813, "status"=w821, "Interface in"=w819) -> ("error out"=w812:errorcluster, "ACQ conf rx"=w817:T2, "Interface out"=w818:refnum<class "Interface.lvclass">)  [unwired: 6 in]
          n297 = Unbundle By Name(w817) -> ("EXPTIME"=w815:dbl)
          n298 = call "Read Exposure Time.vi"("error in (no error)"=w812, "Interface in"=w818) -> ("error out"=w811:errorcluster, "Exposure Time"=w816:dbl)  [unwired: 7 in, 1 out]
          n299 = Equal?(x=w816, y=w815) -> (x = y?=w814:bool)
          n300 = case shown="True" w825 {
            tunnel: [w833 29] -> w823
            tunnel: w824 -> [w834 _]
            tunnel: w814 -> [w832 _]
            frame False {
              n301 = case shown="True" w832 {
                tunnel: [w835 0 ("State")] -> w833
                tunnel: w834 -> [w835 _]
                frame False {
                }
                frame True {
                  (unwired) 40 ("State")
                  # "Ajusta WAIT_\nEXPOSE_\nCOMMAND"
                }
              }
            }
            frame True {
              # "ERRO"
            }
          }
        }
        frame 50 {
          # "Durante a exposição, garantir config=F"
          n302 = Bundle By Name(cluster=w841, "stopping"=FALSE, "config"=FALSE) -> (w840:refnum<class "Channel.lvclass">)
          n303 = call-dynamic "Write cmd.vi"("error in (no error)"=w847, "cmd"="EXPOSE", "Device in"=w840) -> ("error out"=w844:errorcluster, "Device out"=w845:refnum<class "Channel.lvclass">)  [unwired: 7 in]
          n304 = disable-structure shown="Enabled" {
            disable-tunnel: w850 -> [w854 w857]
            disable-tunnel: [w851 w855] -> w848
            disable-tunnel: w846 -> [_ w864]
            disable-tunnel: w845 -> [w853 w862]
            disable-tunnel: w844 -> [w852 w860]
            disable-tunnel: [w853 w861] -> w843
            disable-tunnel: [w852 w858] -> w842
            frame Disabled {
              # "OV 2024-03-12:\nVai para a pausa antes\ndo pedido de STATUS"
              n305 = Increment(x=w854) -> (x+1=w851:i32)
            }
            frame Enabled {
              # "Força a recarga do Ticks com\no valor do relógio do PC.\n\n2024-03-20: Nao precisa mais \npedir STATUS, pois ACS o publica\na cada 1s."
              n306 = call-dynamic "Verif Clock.vi"("error in (no error)"=w860, "period (ms)"=u32 1 ("period"), "State Machine in"=w864) -> ("error out"=w859:errorcluster, "State Machine out"=w863:refnum<class "State Machine.lvclass">)  [unwired: 6 in, 1 out]
              n307 = Add(x=w857, y=3) -> (x+y=w855:i32)
              n308 = call-dynamic "Write State Machine.vi"("error in (no error)"=w859, "State Machine.lvclass"=w863, "Device in"=w862) -> ("error out"=w858:errorcluster, "Device out"=w861:refnum<class "Channel.lvclass">)  [unwired: 7 in]
            }
          }
        }
        frame 51 {
          # "ESTADO OPCIONAL:\nEspera estourar o timeout (200ms).\nApós o timeout vai para o próximo estado enviar STATUS para confirmar\nse o ACS  foi para ACTIVE."
          n309 = call-dynamic "Verif Clock.vi"("error in (no error)"=w872, "period (ms)"=u32 200 ("period"), "State Machine in"=w876) -> ("error out"=w871:errorcluster, "State Machine out"=w875:refnum<class "State Machine.lvclass">)  [unwired: 6 in, 1 out]
          n310 = call-dynamic "Read Timeout.vi"("error in (no error)"=w871, "State Machine in"=w875) -> ("error out"=w870:errorcluster, "Timeout"=w873:bool, "State Machine out"=w874:refnum<class "State Machine.lvclass">)  [unwired: 7 in]
          n311 = call-dynamic "Write State Machine.vi"("error in (no error)"=w870, "State Machine.lvclass"=w874, "Device in"=w878) -> ("error out"=w869:errorcluster, "Device out"=w868:refnum<class "Channel.lvclass">)  [unwired: 7 in]
          n312 = case shown="True" w873 {
            tunnel: [w883 w886] -> w880
            tunnel: w879 -> [w883 w887]
            tunnel: w869 -> [w881 w884]
            tunnel: w868 -> [w882 w885]
            tunnel: [w882 w885] -> w867
            tunnel: [w881 w884] -> w866
            frame False {
            }
            frame True {
              n313 = Increment(x=w887) -> (x+1=w886:i32)
            }
          }
        }
        frame 52 {
          n314 = disable-structure shown="Enabled" {
            disable-tunnel: [w898 w900] -> w893
            disable-tunnel: [w897 w899] -> w892
            disable-tunnel: w889 -> [w895 w900]
            disable-tunnel: w888 -> [w894 w899]
            frame Disabled {
              n315 = call-dynamic "Write cmd.vi"("error in (no error)"=w894, "cmd"="STATUS", "Device in"=w895) -> ("error out"=w897:errorcluster, "Device out"=w898:refnum<class "Channel.lvclass">)  [unwired: 7 in]
            }
            frame Enabled {
              # "ACS publica STATUS"
            }
          }
          n316 = Increment(x=w890) -> (x+1=w891:i32)
        }
        frame 53 {
          # "OV 2024.11.04: \nSe detectou ACTIVE, vai direto para estado 55, \npois o estado 54 foi eliminado.\nSe o ACTIVE for muito rápido e STATUS voltar para IDLE ou WAITING..., \nS4GUI:HandleObservationSync.vi detecta o incremento do CyclesDone.\nO mesmo para S4GUI:HandleObservationAsync.vi."
          # "Status.Texp = Current frame exptime\nlastStatus = cam status (acquiring, idle, writing, reading, ...)\nStatus.Nimages = frames done\nStatus.CubesDone = ciclos realizados pelo ACS\nStatus.SequesDone = sequencias realizadas pelo ACS.\nStatus.UsedDiskSpace = espaco usado no disco.\nStatus.Error = Se TRUE, houve erro na aquisição do canal."
          # "Verifica timeout para ACS iniciar exposição.\nSe estourar timeout é porque o ACS não \nrecebeu o EXPOSE e então volta para 50\npara enviar novo EXPOSE."
          # "Extrair todos os parametros da respsota de STATUS e\natualizar a informação na classe Channel."
          n317 = call-dynamic "Verif Clock.vi"("error in (no error)"=w912, "period (ms)"=u32 500 ("period"), "State Machine in"=w915) -> ("error out"=w913:errorcluster, "State Machine out"=w914:refnum<class "State Machine.lvclass">)  [unwired: 6 in, 1 out]
          n318 = call-dynamic "Read Timeout.vi"("error in (no error)"=w913, "State Machine in"=w914) -> ("error out"=w926:errorcluster, "Timeout"=w916:bool, "State Machine out"=w927:refnum<class "State Machine.lvclass">)  [unwired: 7 in]
          n319 = call-dynamic "Write State Machine.vi"("error in (no error)"=w926, "State Machine.lvclass"=w927, "Device in"=w925) -> ("error out"=w923:errorcluster, "Device out"=w924:refnum<class "Channel.lvclass">)  [unwired: 7 in]
          n320 = call-dynamic "Read resp.vi"("error in (no error)"=w923, "Device in"=w924) -> ("error out"=w945:errorcluster, "resp"=w946:string, "Device out"=w949:refnum<class "Channel.lvclass">)  [unwired: 7 in]
          "resposta do STATUS" <- w946
          n321 = call-dynamic "Read Interface.vi"("error in (no error)"=w945, "Channel in"=w949) -> ("error out"=w944:errorcluster, "Interface.lvclass"=w947:refnum<class "Interface.lvclass">, "Channel out"=w948:refnum<class "Channel.lvclass">)  [unwired: 7 in]
          n322 = call-dynamic "UpdateStatus.vi"("error in (no error)"=w944, "status"=w946, "Interface in"=w947) -> ("error out"=w903:errorcluster, "Interface out"=w905:refnum<class "Interface.lvclass">)  [unwired: 7 in]
          n323 = call-dynamic "Read Error.vi"("error in (no error)"=w903, "Interface in"=w905) -> ("error out"=w902:errorcluster, "Error"=w901:bool, "Interface out"=w904:refnum<class "Interface.lvclass">)  [unwired: 7 in]
          n324 = call-dynamic "Read Exposições realizadas.vi"("error in (no error)"=w902, "Interface in"=w904) -> ("error out"=w932:errorcluster, "Exposições realizadas"=w933:dbl, "Interface out"=w934:refnum<class "Interface.lvclass">)  [unwired: 7 in]
          n325 = call-dynamic "Read Cam_Status.vi"("error in (no error)"=w932, "Interface in"=w934) -> ("error out"=w940:errorcluster, "Cam_Status"=w928:string, "Interface out"=w941:refnum<class "Interface.lvclass">)  [unwired: 7 in]
          n326 = call-dynamic "Read %Acquired.vi"("error in (no error)"=w940, "Interface in"=w941) -> ("error out"=w921:errorcluster, "% Acquired"=w937:dbl, "Interface out"=w922:refnum<class "Interface.lvclass">)  [unwired: 7 in]
          n327 = call-dynamic "Read Number of Cycles.vi"("error in (no error)"=w921, "Interface in"=w922) -> ("error out"=w918:errorcluster, "Number of Cycles"=w920:u32, "Interface out"=w919:refnum<class "Interface.lvclass">)  [unwired: 7 in]
          n328 = call-dynamic "Read Number of Sequences.vi"("error in (no error)"=w918, "Interface in"=w919) -> ("error out"=w908:errorcluster, "Number of Sequences"=w917:u32, "Interface out"=w910:refnum<class "Interface.lvclass">)  [unwired: 7 in]
          n329 = call-dynamic "Read Ocupacao do disco.vi"("error in (no error)"=w908, "Interface in"=w910) -> ("error out"=w907:errorcluster, "Ocupacao do disco"=w906:u16, "Interface out"=w909:refnum<class "Interface.lvclass">)  [unwired: 7 in]
          n330 = call "Read Exposure Time.vi"("error in (no error)"=w907, "Interface in"=w909) -> ("error out"=w930:errorcluster, "Exposure Time"=w939:dbl, "Interface out"=w929:refnum<class "Interface.lvclass">)  [unwired: 7 in]
          n331 = call-dynamic "Write Interface.vi"("error in (no error)"=w930, "Interface.lvclass"=w929, "Channel in"=w948) -> ("error out"=w943:errorcluster, "Channel out"=w942:refnum<class "Channel.lvclass">)  [unwired: 7 in]
          n332 = case shown="\"ACTIVE\"" w928 {
            tunnel: [w953 w956] -> w952
            tunnel: w951 -> [w955 w956]
            tunnel: w916 -> [_ _]
            frame "ACTIVE" {
              n333 = Increment(x=w955) -> (x+1=w954:i32)
              n334 = Increment(x=w954) -> (x+1=w953:i32)
            }
            frame Default {
              # "Não usa o timeout. Deixa o \nS4GUI:HandleObservationSync.vi  e ..Async.vi\ndetectarem o timeout no estado 53 ou incremento de CyclesDone."
            }
          }
          n335 = To Unsigned Long Integer(number=w933) -> (unsigned 32bit integer=w931:u32)
          n336 = Divide(x=w937, y=100.0) -> (x/y=w935:dbl)
          n337 = Multiply(x=w939, y=w935) -> (x*y=w938:dbl)
          n338 = Bundle By Name(cluster=w942, "Texp"=w938, "lastStatus"=w928, "Nimages"=w931, "CyclesDone"=w920, "SequesDone"=w917, "UsedDiskSpace"=w906, "Error"=w901) -> (w950:refnum<class "Channel.lvclass">)
        }
        frame 54 {
          # "OV 2024.11.04: Este estado não é mais utilizado."
          # "Verifica o timeout de 5s para enviar\ntelemetria para o ACS."
          n339 = call-dynamic "Verif Clock 2.vi"("error in (no error)"=w969, "period (ms)"=u32 5000 ("period"), "State Machine in"=w970) -> ("error out"=w967:errorcluster, "State Machine out"=w968:refnum<class "State Machine.lvclass">)  [unwired: 6 in, 1 out]
          n340 = call-dynamic "Read Timeout 2.vi"("error in (no error)"=w967, "State Machine in"=w968) -> ("error out"=w963:errorcluster, "Timeout 2"=w966:bool, "State Machine out"=w964:refnum<class "State Machine.lvclass">)  [unwired: 7 in]
          n341 = call-dynamic "Write State Machine.vi"("error in (no error)"=w963, "State Machine.lvclass"=w964, "Device in"=w965) -> ("error out"=w962:errorcluster, "Device out"=w961:refnum<class "Channel.lvclass">)  [unwired: 7 in]
          n342 = case shown="True" w966 {
            tunnel: [w986 w995] -> w960
            tunnel: [w985 w996] -> w959
            tunnel: [w984 w997] -> w973
            tunnel: w972 -> [w983 w994]
            tunnel: w961 -> [w982 w995]
            tunnel: w962 -> [w981 w996]
            frame False {
              n343 = disable-structure shown="Enabled" {
                disable-tunnel: [w991 w993] -> w986
                disable-tunnel: [w990 w992] -> w985
                disable-tunnel: w982 -> [w988 w993]
                disable-tunnel: w981 -> [w987 w992]
                frame Disabled {
                  n344 = call-dynamic "Write cmd.vi"("error in (no error)"=w987, "cmd"="STATUS", "Device in"=w988) -> ("error out"=w990:errorcluster, "Device out"=w991:refnum<class "Channel.lvclass">)  [unwired: 7 in]
                }
                frame Enabled {
                  # "2024_03_20: Nao pede mais STATUS,\npois ACS o publica a cada 1s."
                }
              }
              n345 = Increment(x=w983) -> (x+1=w984:i32)
            }
            frame True {
              n346 = disable-structure shown="Enabled" {
                disable-tunnel: [59 w999] -> w997
                disable-tunnel: w994 -> [_ w999]
                frame Disabled {
                  # "Estourou timeout de 5s:\nDesvia para enviar dados de \nTELEMETRIA a cada 5s (estado 59)"
                }
                frame Enabled {
                  # "2024-03020: Não evia mais dados\nda TELEMETRIA, pois ACS assina\nas publicacoes do S4GUI, TCS, etc."
                }
              }
            }
          }
          n347 = disable-structure shown="Disabled" {
            disable-tunnel: w960 -> [w977 w980]
            disable-tunnel: w959 -> [w976 w979]
            disable-tunnel: [w975 w980] -> w958
            disable-tunnel: [w974 w979] -> w957
            frame Disabled {
              n348 = call "Write connected.vi"("error in (no error)"=w976, "connected"=FALSE, "Device in"=w977) -> ("error out"=w974:errorcluster, "Device out"=w975:refnum<class "Channel.lvclass">)  [unwired: 7 in]
            }
            frame Enabled {
            }
          }
        }
        frame 55 {
          # "OV 2024.11.04: Não há mais Timeout neste estado.\nFica em 55 até ocorrer um Abort do usuário ou um status desconhecido."
          # "Status.Texp = Current frame exptime\nlastStatus = cam status (acquiring, idle, writing, reading, ...)\nStatus.Nimages = frames done\nStatus.CubesDone = ciclos realizados pelo ACS\nStatus.SequesDone = sequencias realizadas pelo ACS.\nStatus.UsedDiskSpace = espaco usado no disco.\nStatus.Error = Se TRUE, houve erro na aquisição do canal."
          # "Extrair todos os parametros da respsota de STATUS e\natualizar a informação na classe Channel."
          n349 = disable-structure shown="Enabled" {
            disable-tunnel: w1013 -> [w1055 w1058]
            disable-tunnel: [w1053 w1058] -> w1012
            disable-tunnel: w1011 -> [w1052 w1057]
            disable-tunnel: [w1050 FALSE ("Timeout")] -> _
            disable-tunnel: [w1049 w1057] -> w1010
            frame Disabled {
              n350 = call-dynamic "Verif Clock.vi"("error in (no error)"=w1052, "period (ms)"=u32 500 ("period"), "State Machine in"=w1055) -> ("error out"=w1051:errorcluster, "State Machine out"=w1054:refnum<class "State Machine.lvclass">)  [unwired: 6 in, 1 out]
              n351 = call-dynamic "Read Timeout.vi"("error in (no error)"=w1051, "State Machine in"=w1054) -> ("error out"=w1049:errorcluster, "Timeout"=w1050:bool, "State Machine out"=w1053:refnum<class "State Machine.lvclass">)  [unwired: 7 in]
            }
            frame Enabled {
            }
          }
          n352 = call-dynamic "Read resp.vi"("error in (no error)"=w1010, "Device in"=w1020) -> ("error out"=w1040:errorcluster, "resp"=w1041:string, "Device out"=w1044:refnum<class "Channel.lvclass">)  [unwired: 7 in]
          n353 = call-dynamic "Read Interface.vi"("error in (no error)"=w1040, "Channel in"=w1044) -> ("error out"=w1039:errorcluster, "Interface.lvclass"=w1042:refnum<class "Interface.lvclass">, "Channel out"=w1043:refnum<class "Channel.lvclass">)  [unwired: 7 in]
          n354 = call-dynamic "UpdateStatus.vi"("error in (no error)"=w1039, "status"=w1041, "Interface in"=w1042) -> ("error out"=w1002:errorcluster, "Interface out"=w1004:refnum<class "Interface.lvclass">)  [unwired: 7 in]
          n355 = call-dynamic "Read Error.vi"("error in (no error)"=w1002, "Interface in"=w1004) -> ("error out"=w1001:errorcluster, "Error"=w1000:bool, "Interface out"=w1003:refnum<class "Interface.lvclass">)  [unwired: 7 in]
          n356 = call-dynamic "Read Exposições realizadas.vi"("error in (no error)"=w1001, "Interface in"=w1003) -> ("error out"=w1027:errorcluster, "Exposições realizadas"=w1028:dbl, "Interface out"=w1029:refnum<class "Interface.lvclass">)  [unwired: 7 in]
          n357 = call-dynamic "Read Cam_Status.vi"("error in (no error)"=w1027, "Interface in"=w1029) -> ("error out"=w1036:errorcluster, "Cam_Status"=w1025:string, "Interface out"=w1038:refnum<class "Interface.lvclass">)  [unwired: 7 in]
          n358 = call-dynamic "Read %Acquired.vi"("error in (no error)"=w1036, "Interface in"=w1038) -> ("error out"=w1035:errorcluster, "% Acquired"=w1032:dbl, "Interface out"=w1037:refnum<class "Interface.lvclass">)  [unwired: 7 in]
          n359 = call "Read Exposure Time.vi"("error in (no error)"=w1035, "Interface in"=w1037) -> ("error out"=w1018:errorcluster, "Exposure Time"=w1034:dbl, "Interface out"=w1019:refnum<class "Interface.lvclass">)  [unwired: 7 in]
          n360 = call-dynamic "Read Number of Cycles.vi"("error in (no error)"=w1018, "Interface in"=w1019) -> ("error out"=w1015:errorcluster, "Number of Cycles"=w1017:u32, "Interface out"=w1016:refnum<class "Interface.lvclass">)  [unwired: 7 in]
          n361 = call-dynamic "Read Number of Sequences.vi"("error in (no error)"=w1015, "Interface in"=w1016) -> ("error out"=w1008:errorcluster, "Number of Sequences"=w1014:u32, "Interface out"=w1009:refnum<class "Interface.lvclass">)  [unwired: 7 in]
          n362 = call-dynamic "Read Ocupacao do disco.vi"("error in (no error)"=w1008, "Interface in"=w1009) -> ("error out"=w1007:errorcluster, "Ocupacao do disco"=w1005:u16, "Interface out"=w1006:refnum<class "Interface.lvclass">)  [unwired: 7 in]
          n363 = call-dynamic "Write Interface.vi"("error in (no error)"=w1007, "Interface.lvclass"=w1006, "Channel in"=w1043) -> ("error out"=w1024:errorcluster, "Channel out"=w1023:refnum<class "Channel.lvclass">)  [unwired: 7 in]
          n364 = case shown="\"ACQUISITION_ABORTED\", Default" w1025 {
            tunnel: [0 ("State") w1073] -> w1047
            tunnel: w1046 -> [_ w1073]
            tunnel: w1024 -> [w1065 w1069]
            tunnel: [w1062 w1071] -> w1022
            tunnel: w1023 -> [w1063 w1072]
            tunnel: [w1059 w1068] -> w1021
            tunnel: w1012 -> [w1066 w1070]
            frame "ACQUISITION_ABORTED", Default {
              # "OVJ 20230704"
              # "ABORTED ou STATUS desconhecido."
              # "250x20ms=5s"
              n365 = call-dynamic "Write Timer.vi"("error in (no error)"=w1065, "Timer"=u32 250, "State Machine in"=w1066) -> ("error out"=w1060:errorcluster, "State Machine out"=w1061:refnum<class "State Machine.lvclass">)  [unwired: 7 in]
              n366 = call-dynamic "Write State Machine.vi"("error in (no error)"=w1060, "State Machine.lvclass"=w1061, "Device in"=w1063) -> ("error out"=w1059:errorcluster, "Device out"=w1062:refnum<class "Channel.lvclass">)  [unwired: 7 in]
            }
            frame "ACTIVE", "IDLE", "WAITING_EXPOSE_COMMAND" {
              # "STATUS DETECTOR = ACTIVE or WAITING EXPOSE COMMAND"
              n367 = call-dynamic "Write State Machine.vi"("error in (no error)"=w1069, "State Machine.lvclass"=w1070, "Device in"=w1072) -> ("error out"=w1068:errorcluster, "Device out"=w1071:refnum<class "Channel.lvclass">)  [unwired: 7 in]
            }
          }
          n368 = To Unsigned Long Integer(number=w1028) -> (unsigned 32bit integer=w1026:u32)
          n369 = Divide(x=w1032, y=100.0) -> (x/y=w1030:dbl)
          n370 = Multiply(x=w1034, y=w1030) -> (x*y=w1033:dbl)
          n371 = Bundle By Name(cluster=w1022, "Texp"=w1033, "lastStatus"=w1025, "Nimages"=w1026, "CyclesDone"=w1017, "SequesDone"=w1014, "UsedDiskSpace"=w1005, "Error"=w1000) -> (w1045:refnum<class "Channel.lvclass">)
        }
        frame 56 {
          # "Pedido de STATUS para verificar conexão com ACS"
          # "Carrega timeout de 10 ciclos \n(20 x 20ms = 0.4s) \npara resposta do ACS"
          n372 = call-dynamic "Write Timer.vi"("error in (no error)"=w1079, "Timer"=u32 20, "State Machine in"=w1083) -> ("error out"=w1084:errorcluster, "State Machine out"=w1085:refnum<class "State Machine.lvclass">)  [unwired: 7 in]
          n373 = call-dynamic "Write State Machine.vi"("error in (no error)"=w1084, "State Machine.lvclass"=w1085, "Device in"=w1081) -> ("error out"=w1078:errorcluster, "Device out"=w1080:refnum<class "Channel.lvclass">)  [unwired: 7 in]
          n374 = disable-structure shown="Enabled" {
            disable-tunnel: w1080 -> [w1098 w1101]
            disable-tunnel: w1078 -> [w1097 w1100]
            disable-tunnel: [w1096 w1101] -> w1077
            disable-tunnel: [w1095 w1100] -> w1076
            frame Disabled {
              n375 = call-dynamic "Write cmd.vi"("error in (no error)"=w1097, "cmd"="STATUS", "Device in"=w1098) -> ("error out"=w1095:errorcluster, "Device out"=w1096:refnum<class "Channel.lvclass">)  [unwired: 7 in]
            }
            frame Enabled {
              # "2024-03-20: Não envia mais pedido\nde STATUS, pois o ACS publica seu\nSTATUS a cada 1s."
            }
          }
          n376 = Increment(x=w1086) -> (x+1=w1087:i32)
          n377 = disable-structure shown="Disabled" {
            disable-tunnel: w1077 -> [w1092 w1094]
            disable-tunnel: w1076 -> [w1091 w1093]
            disable-tunnel: [w1090 w1094] -> w1075
            disable-tunnel: [w1089 w1093] -> w1074
            frame Disabled {
              # "2024.05.16\ncausa bug de\nfalsa queda na\ncomunicação \ncom ACS"
              n378 = call "Write connected.vi"("error in (no error)"=w1091, "connected"=FALSE, "Device in"=w1092) -> ("error out"=w1089:errorcluster, "Device out"=w1090:refnum<class "Channel.lvclass">)  [unwired: 7 in]
            }
            frame Enabled {
            }
          }
        }
        frame 57 {
          # "Status.Texp = Current frame exptime\nlastStatus = cam status (acquiring, idle, writing, reading, ...)\nStatus.Nimages = frames done\nStatus.CubesDone = ciclos realizados pelo ACS\nStatus.SequesDone = sequencias realizadas pelo ACS.\nStatus.UsedDiskSpace = espaco usado no disco.\nStatus.Error = Se TRUE, houve erro na aquisção do canal."
          # "Extrair todos os parametros da respsota de STATUS e\natualizar a informação na classe Channel."
          n379 = call "Verify Timer.vi"("error in (no error)"=w1128, "State Machine in"=w1127) -> ("error out"=w1124:errorcluster, "State Machine out"=w1126:refnum<class "State Machine.lvclass">)  [unwired: 7 in, 1 out]
          n380 = call-dynamic "Read Timeout.vi"("error in (no error)"=w1124, "State Machine in"=w1126) -> ("error out"=w1119:errorcluster, "Timeout"=w1123:bool, "State Machine out"=w1125:refnum<class "State Machine.lvclass">)  [unwired: 7 in]
          n381 = call "Read connected.vi"("error in (no error)"=w1119, "Device in"=w1122) -> ("error out"=w1120:errorcluster, "connected"=w1118:bool, "Device out"=w1121:refnum<class "Channel.lvclass">)  [unwired: 7 in]
          n382 = call-dynamic "Read resp.vi"("error in (no error)"=w1120, "Device in"=w1121) -> ("error out"=w1148:errorcluster, "resp"=w1149:string, "Device out"=w1152:refnum<class "Channel.lvclass">)  [unwired: 7 in]
          n383 = call-dynamic "Read Interface.vi"("error in (no error)"=w1148, "Channel in"=w1152) -> ("error out"=w1147:errorcluster, "Interface.lvclass"=w1150:refnum<class "Interface.lvclass">, "Channel out"=w1151:refnum<class "Channel.lvclass">)  [unwired: 7 in]
          n384 = call-dynamic "UpdateStatus.vi"("error in (no error)"=w1147, "status"=w1149, "Interface in"=w1150) -> ("error out"=w1104:errorcluster, "Interface out"=w1106:refnum<class "Interface.lvclass">)  [unwired: 7 in]
          n385 = call-dynamic "Read Error.vi"("error in (no error)"=w1104, "Interface in"=w1106) -> ("error out"=w1103:errorcluster, "Error"=w1102:bool, "Interface out"=w1105:refnum<class "Interface.lvclass">)  [unwired: 7 in]
          n386 = call-dynamic "Read Exposições realizadas.vi"("error in (no error)"=w1103, "Interface in"=w1105) -> ("error out"=w1135:errorcluster, "Exposições realizadas"=w1136:dbl, "Interface out"=w1137:refnum<class "Interface.lvclass">)  [unwired: 7 in]
          n387 = call-dynamic "Read Cam_Status.vi"("error in (no error)"=w1135, "Interface in"=w1137) -> ("error out"=w1144:errorcluster, "Cam_Status"=w1133:string, "Interface out"=w1146:refnum<class "Interface.lvclass">)  [unwired: 7 in]
          n388 = call-dynamic "Read %Acquired.vi"("error in (no error)"=w1144, "Interface in"=w1146) -> ("error out"=w1143:errorcluster, "% Acquired"=w1140:dbl, "Interface out"=w1145:refnum<class "Interface.lvclass">)  [unwired: 7 in]
          n389 = call "Read Exposure Time.vi"("error in (no error)"=w1143, "Interface in"=w1145) -> ("error out"=w1116:errorcluster, "Exposure Time"=w1142:dbl, "Interface out"=w1117:refnum<class "Interface.lvclass">)  [unwired: 7 in]
          n390 = call-dynamic "Read Number of Cycles.vi"("error in (no error)"=w1116, "Interface in"=w1117) -> ("error out"=w1113:errorcluster, "Number of Cycles"=w1115:u32, "Interface out"=w1114:refnum<class "Interface.lvclass">)  [unwired: 7 in]
          n391 = call-dynamic "Read Number of Sequences.vi"("error in (no error)"=w1113, "Interface in"=w1114) -> ("error out"=w1109:errorcluster, "Number of Sequences"=w1112:u32, "Interface out"=w1111:refnum<class "Interface.lvclass">)  [unwired: 7 in]
          n392 = call-dynamic "Read Ocupacao do disco.vi"("error in (no error)"=w1109, "Interface in"=w1111) -> ("error out"=w1108:errorcluster, "Ocupacao do disco"=w1107:u16, "Interface out"=w1110:refnum<class "Interface.lvclass">)  [unwired: 7 in]
          n393 = call-dynamic "Write Interface.vi"("error in (no error)"=w1108, "Interface.lvclass"=w1110, "Channel in"=w1151) -> ("error out"=w1132:errorcluster, "Channel out"=w1131:refnum<class "Channel.lvclass">)  [unwired: 7 in]
          n394 = case shown="False" w1118 {
            tunnel: [w1158 w1175] -> w1155
            tunnel: w1154 -> [w1159 w1176]
            tunnel: w1132 -> [w1156 w1173]
            tunnel: [w1161 w1170] -> w1130
            tunnel: w1131 -> [w1162 w1174]
            tunnel: [w1160 w1167] -> w1129
            tunnel: w1125 -> [w1157 w1172]
            tunnel: w1123 -> [_ w1166]
            frame True {
              # "Conneted=T\nACS respondeu"
              n395 = disable-structure shown="Enabled" {
                disable-tunnel: w1159 -> [w1164 _]
                disable-tunnel: [w1163 0] -> w1158
                frame Disabled {
                  n396 = Increment(x=w1164) -> (x+1=w1163:i32)
                }
                frame Enabled {
                }
              }
              n397 = call-dynamic "Write State Machine.vi"("error in (no error)"=w1156, "State Machine.lvclass"=w1157, "Device in"=w1162) -> ("error out"=w1160:errorcluster, "Device out"=w1161:refnum<class "Channel.lvclass">)  [unwired: 7 in]
            }
            frame False {
              # "Conneted=F\nACS não resp."
              n398 = case shown="False" w1166 {
                tunnel: w1176 -> [w1177 _]
                tunnel: [w1177 0] -> w1175
                tunnel: w1174 -> [w1180 w1183]
                tunnel: [w1180 w1183] -> w1171
                tunnel: w1173 -> [w1179 w1184]
                tunnel: [w1179 w1181] -> w1168
                tunnel: w1172 -> [w1178 w1186]
                tunnel: [w1178 w1182] -> w1169
                frame False {
                }
                frame True {
                  n399 = call-dynamic "Write Timer.vi"("error in (no error)"=w1184, "Timer"=u32 250, "State Machine in"=w1186) -> ("error out"=w1181:errorcluster, "State Machine out"=w1182:refnum<class "State Machine.lvclass">)  [unwired: 7 in]
                }
              }
              n400 = call-dynamic "Write State Machine.vi"("error in (no error)"=w1168, "State Machine.lvclass"=w1169, "Device in"=w1171) -> ("error out"=w1167:errorcluster, "Device out"=w1170:refnum<class "Channel.lvclass">)  [unwired: 7 in]
            }
          }
          n401 = Divide(x=w1140, y=100.0) -> (x/y=w1138:dbl)
          n402 = To Unsigned Long Integer(number=w1136) -> (unsigned 32bit integer=w1134:u32)
          n403 = Multiply(x=w1142, y=w1138) -> (x*y=w1141:dbl)
          n404 = Bundle By Name(cluster=w1130, "Texp"=w1141, "lastStatus"=w1133, "Nimages"=w1134, "CyclesDone"=w1115, "SequesDone"=w1112, "UsedDiskSpace"=w1107, "Error"=w1102) -> (w1153:refnum<class "Channel.lvclass">)
        }
        frame 58 {
          w1192 = "}" ("regular expression")
          # "Passa valores da telemetria adquiridos do TCS"
          n405 = call-dynamic "Write State Machine.vi"("error in (no error)"=w1188, "State Machine.lvclass"=w1189, "Device in"=w1199) -> ("error out"=w1196:errorcluster, "Device out"=w1198:refnum<class "Channel.lvclass">)  [unwired: 7 in]
          n406 = Unbundle By Name(w1198) -> ("TCS telemetry"=w1193:string, "Filter"=w1195:u8)
          n407 = Match Pattern(string=w1193, regular expression=w1192) -> (before substring=w1191:string, match substring=w1190:string)  [unwired: 1 in, 2 out]
          n408 = Equal?(x=w1190, y=w1192) -> (x = y?=w1194:bool)
          n409 = case shown="True" w1194 {
            tunnel: [w1203 w1213] -> w1201
            tunnel: [w1202 w1212] -> w1200
            tunnel: w1198 -> [w1203 w1211]
            tunnel: w1196 -> [w1202 w1208]
            tunnel: w1195 -> [_ w1207]
            tunnel: w1191 -> [_ w1206]
            tunnel: w1190 -> [_ w1205]
            frame False {
            }
            frame True {
              (unwired) "\"CTRLINTE\":\"S4GUI\"}" ("string")
              (unwired) "\"FILTER\":\"" ("string")
              n410 = case shown="5" w1207 {
                tunnel: ["CLEAR\"," ("string") "U\"," ("string") "B\"," ("string") "V\"," ("string") "R\"," ("string") "S\"," ("string")] -> _
                frame 0, Default {
                }
                frame 1 {
                }
                frame 2 {
                }
                frame 3 {
                }
                frame 4 {
                }
                frame 5 {
                }
              }
              n411 = Concatenate Strings(w1206, w1205) -> (w1204:string)
              n412 = Concatenate Strings("WRITE_HEADER_DATA " ("cmd"), w1204) -> (w1209:string)
              n413 = disable-structure shown="Enabled" {
                disable-tunnel: [w1218 w1220] -> w1213
                disable-tunnel: [w1217 w1219] -> w1212
                disable-tunnel: w1211 -> [w1216 w1220]
                disable-tunnel: w1209 -> [w1215 _]
                disable-tunnel: w1208 -> [w1214 w1219]
                frame Disabled {
                  n414 = call-dynamic "Write cmd.vi"("error in (no error)"=w1214, "cmd"=w1215, "Device in"=w1216) -> ("error out"=w1217:errorcluster, "Device out"=w1218:refnum<class "Channel.lvclass">)  [unwired: 7 in]
                }
                frame Enabled {
                  # "Não existe mais\neste comando."
                }
              }
            }
          }
        }
        frame 59 {
          w1231 = "}" ("regular expression")
          # "Passa valores da telemetria adquiridos do TCS durante a aquisição do canal (estados 54 e 55)"
          n415 = call-dynamic "Write State Machine.vi"("error in (no error)"=w1227, "State Machine.lvclass"=w1228, "Device in"=w1237) -> ("error out"=w1234:errorcluster, "Device out"=w1236:refnum<class "Channel.lvclass">)  [unwired: 7 in]
          n416 = Unbundle By Name(w1236) -> ("TCS telemetry"=w1232:string)
          n417 = Match Pattern(string=w1232, regular expression=w1231) -> (before substring=w1230:string, match substring=w1229:string)  [unwired: 1 in, 2 out]
          n418 = Equal?(x=w1229, y=w1231) -> (x = y?=w1233:bool)
          n419 = case shown="True" w1233 {
            tunnel: [w1241 w1250] -> w1239
            tunnel: [w1240 w1249] -> w1238
            tunnel: w1236 -> [w1241 w1248]
            tunnel: w1234 -> [w1240 w1245]
            tunnel: w1230 -> [_ w1244]
            tunnel: w1229 -> [_ w1243]
            frame False {
            }
            frame True {
              n420 = Concatenate Strings(w1244, w1243) -> (w1242:string)
              n421 = Concatenate Strings("WRITE_HEADER_DATA " ("cmd"), w1242) -> (w1246:string)
              n422 = disable-structure shown="Enabled" {
                disable-tunnel: [w1255 w1257] -> w1250
                disable-tunnel: [w1254 w1256] -> w1249
                disable-tunnel: w1248 -> [w1253 w1257]
                disable-tunnel: w1246 -> [w1252 _]
                disable-tunnel: w1245 -> [w1251 w1256]
                frame Disabled {
                  n423 = call-dynamic "Write cmd.vi"("error in (no error)"=w1251, "cmd"=w1252, "Device in"=w1253) -> ("error out"=w1254:errorcluster, "Device out"=w1255:refnum<class "Channel.lvclass">)  [unwired: 7 in]
                }
                frame Enabled {
                  # "Não existe mais\neste comando."
                }
              }
            }
          }
        }
        frame 60 {
          # "Carrega timeout de 5 ciclos\npara resposta do ACS"
          n424 = call-dynamic "Write Timer.vi"("Timer"=u32 5, "State Machine in"=w1265) -> ("error out"=w1266:errorcluster, "State Machine out"=w1264:refnum<class "State Machine.lvclass">)  [unwired: 8 in]
          n425 = call-dynamic "Write State Machine.vi"("error in (no error)"=w1266, "State Machine.lvclass"=w1264, "Device in"=w1263) -> ("Device out"=w1260:refnum<class "Channel.lvclass">)  [unwired: 7 in, 1 out]
          n426 = Bundle By Name(cluster=w1260, "config"=TRUE) -> (w1259:refnum<class "Channel.lvclass">)
          n427 = disable-structure shown="Enabled" {
            disable-tunnel: [w1277 w1279] -> w1270
            disable-tunnel: w1269 -> [w1276 w1278]
            disable-tunnel: [w1275 w1278] -> w1268
            disable-tunnel: w1259 -> [w1273 w1279]
            disable-tunnel: w1262 -> [w1272 _]
            disable-tunnel: [w1271 62] -> w1261
            frame Disabled {
              n428 = Increment(x=w1272) -> (x+1=w1271:i32)
              n429 = call-dynamic "Write cmd.vi"("error in (no error)"=w1276, "cmd"="INIT", "Device in"=w1273) -> ("error out"=w1275:errorcluster, "Device out"=w1277:refnum<class "Channel.lvclass">)  [unwired: 7 in]
            }
            frame Enabled {
            }
          }
        }
        frame 61 {
          w1290 = "INITIALIZATION"
          # "Verifica timeout para ACS responder.\nSe estourar timeout é porque o ACS não \nrespondeu e este canal volta para o estado 0\npara não \"travar\" os outros canais no \nS4ACS_GUI:HandleObservation.vi."
          n430 = call "Verify Timer.vi"("error in (no error)"=w1281, "State Machine in"=w1286) -> ("error out"=w1287:errorcluster, "timeout"=w1282:bool, "State Machine out"=w1288:refnum<class "State Machine.lvclass">)  [unwired: 7 in]
          n431 = call-dynamic "Write State Machine.vi"("error in (no error)"=w1287, "State Machine.lvclass"=w1288, "Device in"=w1285) -> ("error out"=w1283:errorcluster, "Device out"=w1284:refnum<class "Channel.lvclass">)  [unwired: 7 in]
          n432 = call-dynamic "Read resp.vi"("error in (no error)"=w1283, "Device in"=w1284) -> ("error out"=w1294:errorcluster, "resp"=w1292:string, "Device out"=w1295:refnum<class "Channel.lvclass">)  [unwired: 7 in]
          "resp INIT" <- w1292
          n433 = Match Pattern(string=w1292, regular expression=w1290) -> (match substring=w1291:string)  [unwired: 1 in, 3 out]
          n434 = Equal?(x=w1291, y=w1290) -> (x = y?=w1289:bool)
          n435 = case shown="True" w1289 {
            tunnel: [w1297 w1302] -> w1296
            tunnel: w1293 -> [w1298 w1303]
            tunnel: w1282 -> [w1299 _]
            frame False {
              n436 = case shown="False" w1299 {
                tunnel: [w1300 0 ("State")] -> w1297
                tunnel: w1298 -> [w1300 _]
                frame False {
                }
                frame True {
                }
              }
            }
            frame True {
              n437 = disable-structure shown="Enabled" {
                disable-tunnel: w1303 -> [w1305 _]
                disable-tunnel: [w1304 54] -> w1302
                frame Disabled {
                  n438 = Increment(x=w1305) -> (x+1=w1304:i32)
                }
                frame Enabled {
                  # "debug:\nNão deve enviar\n WRITE_SETUP para o \nACS antigo"
                }
              }
            }
          }
        }
        frame 62 {
          # "Aguarda para reconfigurar.\n(o timer deve ser recarregado \nquando SM:NextState.vi recebe 62).\n\nIsso foi inserido para dar tempo\ndas VIs de ZMQ estarem prontas\npara enviar e receber mensagens \ndos ACS após o S4GUI:Initialize.vi."
          n439 = call "Verify Timer.vi"("error in (no error)"=w1310, "State Machine in"=w1311) -> ("error out"=w1307:errorcluster, "timeout"=w1312:bool, "State Machine out"=w1309:refnum<class "State Machine.lvclass">)  [unwired: 7 in]
          n440 = case shown="True" w1312 {
            tunnel: [w1320 w1343] -> w1316
            tunnel: [w1321 w1342] -> w1315
            tunnel: w1314 -> [w1322 w1340]
            tunnel: [w1322 w1334] -> w1313
            tunnel: w1307 -> [w1317 w1325]
            tunnel: w1309 -> [w1319 w1327]
            tunnel: w1308 -> [w1318 w1329]
            frame False {
              n441 = call-dynamic "Write State Machine.vi"("error in (no error)"=w1317, "State Machine.lvclass"=w1319, "Device in"=w1318) -> ("error out"=w1321:errorcluster, "Device out"=w1320:refnum<class "Channel.lvclass">)  [unwired: 7 in]
            }
            frame True {
              # "Salta para estado 65\npara tratar a próxima\npublicação de STATUS\n do ACS."
              n442 = call-dynamic "Write Timer.vi"("error in (no error)"=w1325, "Timer"=u32 50, "State Machine in"=w1327) -> ("error out"=w1324:errorcluster, "State Machine out"=w1326:refnum<class "State Machine.lvclass">)  [unwired: 7 in]
              n443 = call-dynamic "Write State Machine.vi"("error in (no error)"=w1324, "State Machine.lvclass"=w1326, "Device in"=w1329) -> ("error out"=w1323:errorcluster, "Device out"=w1328:refnum<class "Channel.lvclass">)  [unwired: 7 in]
              n444 = call-dynamic "Read target cluster.vi"("error in (no error)"=w1323, "Channel in"=w1328) -> ("error out"=w1332:errorcluster, "target cluster"=w1333:T3, "Channel out"=w1331:refnum<class "Channel.lvclass">)  [unwired: 7 in]
              n445 = Increment(x=w1340) -> (x+1=w1341:i32)
              n446 = Flatten To JSON(anything=w1333, error in (no error)=w1332) -> (JSON string=w1337:string, 11:w1336:errorcluster)  [unwired: 1 in]
              n447 = Increment(x=w1341) -> (x+1=w1335:i32)
              n448 = Increment(x=w1335) -> (x+1=w1334:i32)
              n449 = Concatenate Strings("WRITE_SETUP " ("cmd"), w1337) -> (w1338:string)
              n450 = call-dynamic "Write cmd.vi"("error in (no error)"=w1336, "cmd"=w1338, "Device in"=w1331) -> ("error out"=w1342:errorcluster, "Device out"=w1343:refnum<class "Channel.lvclass">)  [unwired: 7 in]
            }
          }
        }
        frame 63 {
          # "Não há resposta para o comando WRTITE_SETUP\nQuando estourar timeout vai para o estado 64 para \nobter o STATUS do ACS."
          n451 = call "Verify Timer.vi"("error in (no error)"=w1347, "State Machine in"=w1349) -> ("error out"=w1350:errorcluster, "timeout"=w1346:bool, "State Machine out"=w1351:refnum<class "State Machine.lvclass">)  [unwired: 7 in]
          n452 = call-dynamic "Write State Machine.vi"("error in (no error)"=w1350, "State Machine.lvclass"=w1351, "Device in"=w1348) -> ("error out"=w1344:errorcluster, "Device out"=w1345:refnum<class "Channel.lvclass">)  [unwired: 7 in]
          n453 = case shown="True" w1346 {
            tunnel: [w1354 w1355] -> w1353
            tunnel: w1352 -> [w1354 w1356]
            frame False {
            }
            frame True {
              n454 = Increment(x=w1356) -> (x+1=w1355:i32)
            }
          }
        }
        frame 64 {
          # "Carrega timeout de 50 ciclos\npara resposta do ACS"
          n455 = call-dynamic "Write Timer.vi"("error in (no error)"=w1359, "Timer"=u32 50, "State Machine in"=w1362) -> ("error out"=w1363:errorcluster, "State Machine out"=w1361:refnum<class "State Machine.lvclass">)  [unwired: 7 in]
          n456 = call-dynamic "Write State Machine.vi"("error in (no error)"=w1363, "State Machine.lvclass"=w1361, "Device in"=w1360) -> ("error out"=w1357:errorcluster, "Device out"=w1358:refnum<class "Channel.lvclass">)  [unwired: 7 in]
          n457 = disable-structure shown="Enabled" {
            disable-tunnel: [w1373 w1375] -> w1368
            disable-tunnel: [w1372 w1374] -> w1367
            disable-tunnel: w1358 -> [w1371 w1375]
            disable-tunnel: w1357 -> [w1369 w1374]
            frame Disabled {
              n458 = call-dynamic "Write cmd.vi"("error in (no error)"=w1369, "cmd"="READ_SETUP ", "Device in"=w1371) -> ("error out"=w1372:errorcluster, "Device out"=w1373:refnum<class "Channel.lvclass">)  [unwired: 7 in]
            }
            frame Enabled {
            }
          }
          n459 = Increment(x=w1365) -> (x+1=w1366:i32)
        }
        frame 65 {
          n460 = call "Verify Timer.vi"("error in (no error)"=w1395, "State Machine in"=w1397) -> ("error out"=w1398:errorcluster, "timeout"=w1384:bool, "State Machine out"=w1399:refnum<class "State Machine.lvclass">)  [unwired: 7 in]
          n461 = call-dynamic "Write State Machine.vi"("error in (no error)"=w1398, "State Machine.lvclass"=w1399, "Device in"=w1396) -> ("error out"=w1393:errorcluster, "Device out"=w1394:refnum<class "Channel.lvclass">)  [unwired: 7 in]
          n462 = call-dynamic "Read resp.vi"("error in (no error)"=w1393, "Device in"=w1394) -> ("error out"=w1389:errorcluster, "resp"=w1379:string, "Device out"=w1376:refnum<class "Channel.lvclass">)  [unwired: 7 in]
          n463 = disable-structure shown="Enabled" {
            disable-tunnel: w1376 -> [w1400 w1415]
            disable-tunnel: [w1407 w1410] -> w1391
            disable-tunnel: [w1406 w1412] -> w1390
            disable-tunnel: w1389 -> [w1404 w1413]
            disable-tunnel: [w1403 w1409] -> w1388
            disable-tunnel: w1379 -> [w1402 w1414]
            disable-tunnel: [w1401 w1408] -> w1378
            disable-tunnel: [w1400 w1411] -> w1377
            frame Disabled {
              n464 = Unbundle By Name(w1400) -> ("Interface.lvclass"=w1405:refnum<class "Interface.lvclass">)
              n465 = call-dynamic "UpdateCCDconf.vi"("error in (no error)"=w1404, "status"=w1402, "Interface in"=w1405) -> ("error out"=w1406:errorcluster, "CCD conf rx"=w1403:T3, "Cluster comparison"=w1401:T1, "Interface out"=w1407:refnum<class "Interface.lvclass">)  [unwired: 5 in]
            }
            frame Enabled {
              n466 = call-dynamic "Check CCD Config.vi"("error in (no error)"=w1413, "Status"=w1414, "Channel in"=w1415) -> ("error out"=w1412:errorcluster, "cluster RX"=w1409:T3, "Cluster COMPARE"=w1408:T1, "Channel out"=w1411:refnum<class "Channel.lvclass">)  [unwired: 5 in]
              n467 = Unbundle By Name(w1411) -> ("Interface.lvclass"=w1410:refnum<class "Interface.lvclass">)
            }
          }
          n468 = case shown="True" w1384 {
            tunnel: w1391 -> [w1418 w1433]
            tunnel: w1390 -> [w1417 w1432]
            tunnel: w1388 -> [_ w1428]
            tunnel: [w1418 w1431] -> w1386
            tunnel: [w1417 w1430] -> w1387
            tunnel: [w1419 w1427] -> w1385
            tunnel: w1381 -> [w1416 w1429]
            tunnel: [w1416 w1424] -> w1380
            tunnel: w1378 -> [_ w1427]
            frame False {
              n469 = disable-structure shown="Enabled" {
                disable-tunnel: [T1 {"ACQUISITION_MODE"=FALSE, "TRIGGER_MODE"=FALSE, "READ_MODE"=FALSE, "PREAMP"=FALSE, "READOUT_RATE"=FALSE, "VERTICAL_SHIFT_SPEED"=FALSE, "EM_MODE"=FALSE, "EM_GAIN"=FALSE, "SHUTTER_MODE"=FALSE, "SHUTTER_TTL"=FALSE, "SHUTTER_OPENING_TIME"=FALSE, "SHUTTER_CLOSING_TIME"=FALSE, "VBIN"=FALSE, "HBIN"=FALSE, "INITIAL_LINE"=FALSE, "INITIAL_COLUMN"=FALSE, "FINAL_LINE"=FALSE, "FINAL_COLUMN"=FALSE, "FRAME_TRANSFER"=FALSE, "VERTICAL_CLOCK_VOLTAGE"=FALSE, "AD_CHANNEL"=FALSE} ("x = y?") T1 {"ACQUISITION_MODE"=TRUE, "TRIGGER_MODE"=TRUE, "READ_MODE"=TRUE, "PREAMP"=TRUE, "READOUT_RATE"=TRUE, "VERTICAL_SHIFT_SPEED"=TRUE, "EM_MODE"=TRUE, "EM_GAIN"=TRUE, "SHUTTER_MODE"=TRUE, "SHUTTER_TTL"=TRUE, "SHUTTER_OPENING_TIME"=TRUE, "SHUTTER_CLOSING_TIME"=TRUE, "VBIN"=TRUE, "HBIN"=TRUE, "INITIAL_LINE"=TRUE, "INITIAL_COLUMN"=TRUE, "FINAL_LINE"=TRUE, "FINAL_COLUMN"=TRUE, "FRAME_TRANSFER"=TRUE, "VERTICAL_CLOCK_VOLTAGE"=TRUE, "AD_CHANNEL"=TRUE} ("x = y?")] -> w1419
                frame Disabled {
                }
                frame Enabled {
                }
              }
            }
            frame True {
              n470 = disable-structure shown="Enabled" {
                disable-tunnel: w1429 -> [w1435 _]
                disable-tunnel: [w1434 0] -> w1422
                frame Disabled {
                  n471 = Increment(x=w1435) -> (x+1=w1434:i32)
                }
                frame Enabled {
                }
              }
              n472 = Not Equal?(x=T1 {"ACQUISITION_MODE"=TRUE, "TRIGGER_MODE"=TRUE, "READ_MODE"=TRUE, "PREAMP"=TRUE, "READOUT_RATE"=TRUE, "VERTICAL_SHIFT_SPEED"=TRUE, "EM_MODE"=TRUE, "EM_GAIN"=TRUE, "SHUTTER_MODE"=TRUE, "SHUTTER_TTL"=TRUE, "SHUTTER_OPENING_TIME"=TRUE, "SHUTTER_CLOSING_TIME"=TRUE, "VBIN"=TRUE, "HBIN"=TRUE, "INITIAL_LINE"=TRUE, "INITIAL_COLUMN"=TRUE, "FINAL_LINE"=TRUE, "FINAL_COLUMN"=TRUE, "FRAME_TRANSFER"=TRUE, "VERTICAL_CLOCK_VOLTAGE"=TRUE, "AD_CHANNEL"=TRUE}, y=w1427) -> (x != y?=w1425:bool)
              n473 = call-dynamic "Set CCD_Config.vi"("error in (no error)"=w1432, "input cluster"=w1428, "Interface in"=w1433) -> ("error out"=w1430:errorcluster, "Interface out"=w1431:refnum<class "Interface.lvclass">)  [unwired: 7 in]
              n474 = Select(t=27 ("f"), s=w1425, f=w1422) -> (s? t:f=w1424:i32)
            }
          }
          "x = y?" <- w1385
          n475 = call "Write Checked Params.vi"("error in (no error)"=w1387, "Checked Params"=w1385, "Interface in"=w1386) -> ("error out"=w1382:errorcluster, "Interface out"=w1383:refnum<class "Interface.lvclass">)  [unwired: 7 in]
          n476 = Bundle By Name(cluster=w1377, "Interface.lvclass"=w1383) -> (w1392:refnum<class "Channel.lvclass">)
        }
        frame 66 {
          # "O valor do COOLER aqui\nfoi carregado no Acquistion:Init.vi"
          # "Se COOLER=0\n        SET COLLERPOWER_STATUS 0\n        AVANÇA ESTADO\n        VAI PRA 0\nSe COOLER=1:\n      DESVIA PARA Estado 35"
          # "Carrega timeout de 50 ciclos\npara resposta do ACS"
          n477 = call-dynamic "Write Timer.vi"("error in (no error)"=w1444, "Timer"=u32 50, "State Machine in"=w1445) -> ("error out"=w1442:errorcluster, "State Machine out"=w1441:refnum<class "State Machine.lvclass">)  [unwired: 7 in]
          n478 = call-dynamic "Write State Machine.vi"("error in (no error)"=w1442, "State Machine.lvclass"=w1441, "Device in"=w1443) -> ("error out"=w1440:errorcluster, "Device out"=w1439:refnum<class "Channel.lvclass">)  [unwired: 7 in]
          n479 = Unbundle By Name(w1439) -> ("Interface.lvclass"=w1438:refnum<class "Interface.lvclass">)
          n480 = call-dynamic "Read Cooler ON_OFF.vi"("Interface in"=w1438) -> ("Cooler ON/OFF"=w1437:i16)  [unwired: 8 in, 2 out]
          n481 = case shown="0, Default" w1437 {
            tunnel: [w1453 w1460] -> w1450
            tunnel: [w1452 w1459] -> w1449
            tunnel: [35 w1458] -> w1448
            tunnel: w1447 -> [_ w1457]
            tunnel: w1440 -> [w1452 w1455]
            tunnel: w1439 -> [w1453 w1454]
            frame 1 {
              # "Se COOLER foi carregado com 1 na inicialização.\ndesvia para 35 para setar a temperatura e ligar o COOLER."
            }
            frame 0, Default {
              n482 = Increment(x=w1457) -> (x+1=w1458:i32)
              n483 = call-dynamic "Write cmd.vi"("error in (no error)"=w1455, "cmd"="SET COOLER_POWER_STATUS 0", "Device in"=w1454) -> ("error out"=w1459:errorcluster, "Device out"=w1460:refnum<class "Channel.lvclass">)  [unwired: 7 in]
            }
          }
        }
        frame 67 {
          # "Compara o parametro enviado com\no parametro no Acquisition Configuration\nda msg de STATUS do ACS."
          n484 = call "Verify Timer.vi"("error in (no error)"=w1476, "State Machine in"=w1480) -> ("error out"=w1475:errorcluster, "timeout"=w1473:bool, "State Machine out"=w1477:refnum<class "State Machine.lvclass">)  [unwired: 7 in]
          n485 = call-dynamic "Write State Machine.vi"("error in (no error)"=w1475, "State Machine.lvclass"=w1477, "Device in"=w1479) -> ("error out"=w1474:errorcluster, "Device out"=w1478:refnum<class "Channel.lvclass">)  [unwired: 7 in]
          n486 = call-dynamic "Read resp.vi"("error in (no error)"=w1474, "Device in"=w1478) -> ("error out"=w1465:errorcluster, "resp"=w1466:string, "Device out"=w1461:refnum<class "Channel.lvclass">)  [unwired: 7 in]
          n487 = Unbundle By Name(w1461) -> ("Interface.lvclass"=w1472:refnum<class "Interface.lvclass">)
          n488 = call-dynamic "UpdateACQconf.vi"("error in (no error)"=w1465, "status"=w1466, "Interface in"=w1472) -> ("error out"=w1467:errorcluster, "ACQ conf rx"=w1470:T2, "Interface out"=w1471:refnum<class "Interface.lvclass">)  [unwired: 6 in]
          n489 = Unbundle By Name(w1470) -> ("COOLER_POWER_STATUS"=w1468:dbl)
          n490 = call-dynamic "Read Cooler ON_OFF.vi"("error in (no error)"=w1467, "Interface in"=w1471) -> ("error out"=w1463:errorcluster, "Cooler ON/OFF"=w1469:i16)  [unwired: 7 in, 1 out]
          n491 = To Word Integer(number=w1468) -> (16bit integer=w1462:i16)
          n492 = Equal?(x=w1469, y=w1462) -> (x = y?=w1464:bool)
          n493 = case shown="True" w1464 {
            tunnel: [w1483 w1488] -> w1482
            tunnel: w1481 -> [w1484 _]
            tunnel: w1473 -> [w1485 _]
            frame False {
              n494 = case shown="True" w1485 {
                tunnel: [w1486 300 ("State")] -> w1483
                tunnel: w1484 -> [w1486 _]
                frame False {
                }
                frame True {
                  (unwired) 40 ("State")
                  # "2024.07.01:\nConfigura\nsuffix e  \nExp mode."
                }
              }
            }
            frame True {
              n495 = disable-structure shown="Enabled" {
                disable-tunnel: [54 ("State") 300 ("State")] -> w1488
                frame Disabled {
                }
                frame Enabled {
                  # "Fim. Vai para 300\nsetar Suffix e\nhabilitar WAIT_\nEXPOSE_COMMAND"
                }
              }
            }
          }
        }
        frame 70 {
          w1493 = "" ("resp")
          n496 = call-dynamic "Write cmd.vi"("error in (no error)"=w1492, "cmd"="STOP_ACQUISITION", "Device in"=w1491) -> ("error out"=w1503:errorcluster, "Device out"=w1504:refnum<class "Channel.lvclass">)  [unwired: 7 in]
          n497 = call-dynamic "Write resp.vi"("error in (no error)"=w1503, "resp"=w1493, "Device in"=w1504) -> ("error out"=w1499:errorcluster, "Device out"=w1502:refnum<class "Channel.lvclass">)  [unwired: 7 in]
          n498 = call-dynamic "Read Interface.vi"("error in (no error)"=w1499, "Channel in"=w1502) -> ("error out"=w1498:errorcluster, "Interface.lvclass"=w1497:refnum<class "Interface.lvclass">, "Channel out"=w1501:refnum<class "Channel.lvclass">)  [unwired: 7 in]
          n499 = call-dynamic "UpdateStatus.vi"("error in (no error)"=w1498, "status"=w1493, "Interface in"=w1497) -> ("error out"=w1495:errorcluster, "Interface out"=w1496:refnum<class "Interface.lvclass">)  [unwired: 7 in]
          n500 = call-dynamic "Write Interface.vi"("error in (no error)"=w1495, "Interface.lvclass"=w1496, "Channel in"=w1501) -> ("error out"=w1494:errorcluster, "Channel out"=w1500:refnum<class "Channel.lvclass">)  [unwired: 7 in]
          n501 = Increment(x=w1506) -> (x+1=w1507:i32)
        }
        frame 71 {
          w1516 = "IDLE" ("regular expression")
          # "2025.07.28: Fica aguardando aqui (sem limite) até que CCD_STATUS = IDLE.\nPara encerrar a aquisição imediatamente, deve-se clicar ABORT no painel."
          n502 = call-dynamic "Read resp.vi"("error in (no error)"=w1510, "Device in"=w1511) -> ("error out"=w1526:errorcluster, "resp"=w1518:string, "Device out"=w1527:refnum<class "Channel.lvclass">)  [unwired: 7 in]
          n503 = call-dynamic "Read Interface.vi"("error in (no error)"=w1526, "Channel in"=w1527) -> ("error out"=w1524:errorcluster, "Interface.lvclass"=w1525:refnum<class "Interface.lvclass">, "Channel out"=w1521:refnum<class "Channel.lvclass">)  [unwired: 7 in]
          n504 = call-dynamic "UpdateStatus.vi"("error in (no error)"=w1524, "status"=w1518, "Interface in"=w1525) -> ("error out"=w1522:errorcluster, "Interface out"=w1523:refnum<class "Interface.lvclass">)  [unwired: 7 in]
          n505 = call-dynamic "Read Acq_Status.vi"("error in (no error)"=w1522, "Interface in"=w1523) -> ("error out"=w1519:errorcluster, "Acq_Status"=w1515:string, "Interface out"=w1520:refnum<class "Interface.lvclass">)  [unwired: 7 in]
          n506 = call-dynamic "Write Interface.vi"("error in (no error)"=w1519, "Interface.lvclass"=w1520, "Channel in"=w1521) -> ("error out"=w1512:errorcluster, "Channel out"=w1509:refnum<class "Channel.lvclass">)  [unwired: 7 in]
          n507 = Match Pattern(string=w1515, regular expression=w1516) -> (match substring=w1517:string)  [unwired: 1 in, 3 out]
          n508 = Equal?(x=w1517, y=w1516) -> (x = y?=w1513:bool)
          n509 = case shown="True" w1513 {
            tunnel: [w1530 u32 0 ("Timer")] -> w1528
            tunnel: w1514 -> [w1530 _]
            tunnel: w1509 -> [w1529 w1532]
            tunnel: [w1529 w1531] -> w1508
            frame False {
            }
            frame True {
              # "2025.07.28: Sinaliza para S4GUI:\nHandleObservationque a aquisição \nfoi cancelada."
              n510 = Bundle By Name(cluster=w1532, "stopping"=TRUE) -> (w1531:refnum<class "Channel.lvclass">)
            }
          }
        }
        frame 75 {
          w1538 = "" ("resp")
          # "Encerra execução do ACS após o parking do intrumento. Vide estado 230 de S4GUI:HandleObservationSync.vi"
          # "Carrega timeout de 5 ciclos\npara resposta do ACS"
          n511 = call-dynamic "Write Timer.vi"("error in (no error)"=w1551, "Timer"=u32 5, "State Machine in"=w1553) -> ("error out"=w1555:errorcluster, "State Machine out"=w1554:refnum<class "State Machine.lvclass">)  [unwired: 7 in]
          n512 = call-dynamic "Write State Machine.vi"("error in (no error)"=w1555, "State Machine.lvclass"=w1554, "Device in"=w1552) -> ("error out"=w1550:errorcluster, "Device out"=w1537:refnum<class "Channel.lvclass">)  [unwired: 7 in]
          n513 = Bundle By Name(cluster=w1537, "stopping"=TRUE) -> (w1535:refnum<class "Channel.lvclass">)
          n514 = call-dynamic "Write cmd.vi"("error in (no error)"=w1550, "cmd"="STOP_APP", "Device in"=w1535) -> ("error out"=w1548:errorcluster, "Device out"=w1549:refnum<class "Channel.lvclass">)  [unwired: 7 in]
          n515 = call-dynamic "Write resp.vi"("error in (no error)"=w1548, "resp"=w1538, "Device in"=w1549) -> ("error out"=w1544:errorcluster, "Device out"=w1547:refnum<class "Channel.lvclass">)  [unwired: 7 in]
          n516 = call-dynamic "Read Interface.vi"("error in (no error)"=w1544, "Channel in"=w1547) -> ("error out"=w1543:errorcluster, "Interface.lvclass"=w1542:refnum<class "Interface.lvclass">, "Channel out"=w1546:refnum<class "Channel.lvclass">)  [unwired: 7 in]
          n517 = call-dynamic "UpdateStatus.vi"("error in (no error)"=w1543, "status"=w1538, "Interface in"=w1542) -> ("error out"=w1540:errorcluster, "Interface out"=w1541:refnum<class "Interface.lvclass">)  [unwired: 7 in]
          n518 = call-dynamic "Write Interface.vi"("error in (no error)"=w1540, "Interface.lvclass"=w1541, "Channel in"=w1546) -> ("error out"=w1539:errorcluster, "Channel out"=w1545:refnum<class "Channel.lvclass">)  [unwired: 7 in]
          n519 = Increment(x=w1558) -> (x+1=w1559:i32)
        }
        frame 76 {
          w1561 = "DONE"
          n520 = call-dynamic "Read resp.vi"("error in (no error)"=w1568, "Device in"=w1569) -> ("error out"=w1565:errorcluster, "resp"=w1563:string, "Device out"=w1566:refnum<class "Channel.lvclass">)  [unwired: 7 in]
          n521 = Match Pattern(string=w1563, regular expression=w1561) -> (match substring=w1562:string)  [unwired: 1 in, 3 out]
          n522 = Equal?(x=w1562, y=w1561) -> ()  [unwired: 1 out]
          n523 = case shown="True" TRUE {
            tunnel: [w1570 0 ("State")] -> w1567
            tunnel: w1564 -> [w1570 _]
            frame False {
            }
            frame True {
            }
          }
        }
        frame 80 {
          n524 = call-dynamic "Write Timer.vi"("error in (no error)"=w1574, "Timer"=u32 200, "State Machine in"=w1578) -> ("error out"=w1573:errorcluster, "State Machine out"=w1577:refnum<class "State Machine.lvclass">)  [unwired: 7 in]
          n525 = call-dynamic "Write State Machine.vi"("error in (no error)"=w1573, "State Machine.lvclass"=w1577, "Device in"=w1576) -> ("error out"=w1572:errorcluster, "Device out"=w1575:refnum<class "Channel.lvclass">)  [unwired: 7 in]
          n526 = call-dynamic "Write cmd.vi"("error in (no error)"=w1572, "cmd"="ABORT_ACQUISITION", "Device in"=w1575) -> ("error out"=w1583:errorcluster, "Device out"=w1584:refnum<class "Channel.lvclass">)  [unwired: 7 in]
          n527 = Increment(x=w1586) -> (x+1=w1587:i32)
          n528 = call-dynamic "Write resp.vi"("error in (no error)"=w1583, "resp"="", "Device in"=w1584) -> ("error out"=w1582:errorcluster, "Device out"=w1581:refnum<class "Channel.lvclass">)  [unwired: 7 in]
        }
        frame 81 {
          w1594 = "IDLE" ("regular expression")
          n529 = call "Verify Timer.vi"("error in (no error)"=w1603, "State Machine in"=w1604) -> ("error out"=w1599:errorcluster, "timeout"=w1597:bool, "State Machine out"=w1602:refnum<class "State Machine.lvclass">)  [unwired: 7 in]
          n530 = call-dynamic "Write State Machine.vi"("error in (no error)"=w1599, "State Machine.lvclass"=w1602, "Device in"=w1601) -> ("error out"=w1598:errorcluster, "Device out"=w1600:refnum<class "Channel.lvclass">)  [unwired: 7 in]
          n531 = call-dynamic "Read resp.vi"("error in (no error)"=w1598, "Device in"=w1600) -> ("error out"=w1612:errorcluster, "resp"=w1596:string, "Device out"=w1613:refnum<class "Channel.lvclass">)  [unwired: 7 in]
          n532 = call-dynamic "Read Interface.vi"("error in (no error)"=w1612, "Channel in"=w1613) -> ("error out"=w1610:errorcluster, "Interface.lvclass"=w1611:refnum<class "Interface.lvclass">, "Channel out"=w1607:refnum<class "Channel.lvclass">)  [unwired: 7 in]
          n533 = call-dynamic "UpdateStatus.vi"("error in (no error)"=w1610, "status"=w1596, "Interface in"=w1611) -> ("error out"=w1608:errorcluster, "Interface out"=w1609:refnum<class "Interface.lvclass">)  [unwired: 7 in]
          n534 = call-dynamic "Read Acq_Status.vi"("error in (no error)"=w1608, "Interface in"=w1609) -> ("error out"=w1605:errorcluster, "Acq_Status"=w1593:string, "Interface out"=w1606:refnum<class "Interface.lvclass">)  [unwired: 7 in]
          n535 = call-dynamic "Write Interface.vi"("error in (no error)"=w1605, "Interface.lvclass"=w1606, "Channel in"=w1607) -> ("error out"=w1590:errorcluster, "Channel out"=w1589:refnum<class "Channel.lvclass">)  [unwired: 7 in]
          n536 = Match Pattern(string=w1593, regular expression=w1594) -> (match substring=w1595:string)  [unwired: 1 in, 3 out]
          n537 = Equal?(x=w1595, y=w1594) -> (x = y?=w1591:bool)
          n538 = case shown="True" w1597 {
            tunnel: [w1618 u32 28 ("State")] -> w1614
            tunnel: w1592 -> [w1617 _]
            tunnel: w1591 -> [w1619 _]
            tunnel: w1589 -> [w1616 w1626]
            tunnel: [w1615 w1626] -> w1588
            frame False {
              n539 = case shown="False" w1619 {
                tunnel: [w1621 u32 0 ("Timer")] -> w1618
                tunnel: w1617 -> [w1621 _]
                tunnel: w1616 -> [w1620 w1623]
                tunnel: [w1620 w1622] -> w1615
                frame False {
                }
                frame True {
                  # "2025.07.28: Sinaliza para S4GUI:\nHandleObservationque a aquisição \nfoi abortada."
                  n540 = Bundle By Name(cluster=w1623, "stopping"=TRUE) -> (w1622:refnum<class "Channel.lvclass">)
                }
              }
            }
            frame True {
              # "ERRO"
            }
          }
        }
        frame 90 {
          n541 = Unbundle By Name(w1629) -> ("wait_expose"=w1628:bool)
          n542 = case shown="False" w1628 {
            tunnel: w1637 -> [w1642 w1643]
            tunnel: w1629 -> [w1641 w1644]
            tunnel: [w1640 w1644] -> w1634
            tunnel: [w1639 w1643] -> w1633
            frame False {
              # "20240710: Se o ACS não estiver\nesperando EXPOSE, manda pausar a\naquisição."
              n543 = call-dynamic "Write cmd.vi"("error in (no error)"=w1642, "cmd"="PAUSE_ACQUISITION", "Device in"=w1641) -> ("error out"=w1639:errorcluster, "Device out"=w1640:refnum<class "Channel.lvclass">)  [unwired: 7 in]
            }
            frame True {
            }
          }
          n544 = call-dynamic "Write resp.vi"("error in (no error)"=w1633, "resp"="", "Device in"=w1634) -> ("error out"=w1632:errorcluster, "Device out"=w1631:refnum<class "Channel.lvclass">)  [unwired: 7 in]
          n545 = Increment(x=w1635) -> (x+1=w1636:i32)
        }
        frame 91 {
          w1646 = "DONE"
          # "Volta pra repouso para que os indicadores de progresso da aquisição sejam atualizados na GUI."
          n546 = call-dynamic "Read resp.vi"("error in (no error)"=w1651, "Device in"=w1652) -> ("error out"=w1649:errorcluster, "resp"=w1648:string, "Device out"=w1650:refnum<class "Channel.lvclass">)  [unwired: 7 in]
          "resp PAUSE" <- w1648
          n547 = Match Pattern(string=w1648, regular expression=w1646) -> (match substring=w1647:string)  [unwired: 1 in, 3 out]
          n548 = Equal?(x=w1647, y=w1646) -> ()  [unwired: 1 out]
        }
        frame 96 {
          n549 = Unbundle By Name(w1654) -> ("wait_expose"=w1653:bool)
          n550 = case shown="False" w1653 {
            tunnel: w1662 -> [w1667 w1668]
            tunnel: w1654 -> [w1666 w1669]
            tunnel: [w1665 w1669] -> w1659
            tunnel: [w1664 w1668] -> w1658
            frame False {
              # "20240710: Se o ACS não estiver\nesperando EXPOSE, manda reiniciar\na aquisição."
              n551 = call-dynamic "Write cmd.vi"("error in (no error)"=w1667, "cmd"="RESUME_ACQUISITION", "Device in"=w1666) -> ("error out"=w1664:errorcluster, "Device out"=w1665:refnum<class "Channel.lvclass">)  [unwired: 7 in]
            }
            frame True {
            }
          }
          n552 = call-dynamic "Write resp.vi"("error in (no error)"=w1658, "resp"="", "Device in"=w1659) -> ("error out"=w1657:errorcluster, "Device out"=w1656:refnum<class "Channel.lvclass">)  [unwired: 7 in]
          n553 = Increment(x=w1660) -> (x+1=w1661:i32)
        }
        frame 97 {
          w1672 = "DONE"
          # "No estado 500 de S4GUI:HandleObservationSync.vi e S4GUI:HandleObservationAsync.vi\né feita a verificação se o canal foi pra repouso (estados 0,56,57 de Channel:Run.vi). \nSe foi, o estado de retorno do canal é recarregado e o processo continua de onde parou."
          n554 = call-dynamic "Read resp.vi"("error in (no error)"=w1676, "Device in"=w1677) -> ("error out"=w1671:errorcluster, "resp"=w1674:string, "Device out"=w1675:refnum<class "Channel.lvclass">)  [unwired: 7 in]
          "resp RESUME" <- w1674
          n555 = Match Pattern(string=w1674, regular expression=w1672) -> (match substring=w1673:string)  [unwired: 1 in, 3 out]
          n556 = Equal?(x=w1673, y=w1672) -> ()  [unwired: 1 out]
        }
        frame 100 {
          (unwired) "S4ACS C1/C2/C3/C4 NIMAGES " ("cmd")
          n557 = call-dynamic "Write cmd.vi"("error in (no error)"=w1683, "cmd"="INIT", "Device in"=w1681) -> ("error out"=w1682:errorcluster, "Device out"=w1684:refnum<class "Channel.lvclass">)  [unwired: 7 in]
          n558 = Increment(x=w1679) -> (x+1=w1680:i32)
        }
        frame 101 {
          w1686 = "\r\n"
          n559 = call-dynamic "Read resp.vi"("error in (no error)"=w1694, "Device in"=w1695) -> ("error out"=w1691:errorcluster, "resp"=w1685:string, "Device out"=w1688:refnum<class "Channel.lvclass">)  [unwired: 7 in]
          n560 = Match Pattern(string=w1685, regular expression=w1686) -> (match substring=w1689:string)  [unwired: 1 in, 3 out]
          n561 = Equal?(x=w1689, y=w1686) -> (x = y?=w1693:bool)
          n562 = case shown="False" w1693 {
            tunnel: [w1696 u8 0] -> w1692
            tunnel: w1690 -> [w1696 _]
            tunnel: w1688 -> [w1697 w1701]
            tunnel: [w1697 w1700] -> w1687
            tunnel: w1685 -> [_ w1699]
            frame False {
            }
            frame True {
              n563 = Bundle By Name(cluster=w1701, "lastStatus"=w1699) -> (w1700:refnum<class "Channel.lvclass">)
            }
          }
        }
        frame 102 {
          w1709 = "EXPTIME "
          n564 = Unbundle By Name(w1703) -> ("lastStatus"=w1704:string)
          n565 = Match Pattern(string=w1704, regular expression=w1709) -> (match substring=w1708:string, after substring=w1706:string)  [unwired: 1 in, 2 out]
          n566 = Equal?(x=w1708, y=w1709) -> (x = y?=w1712:bool)
          n567 = case shown="True" w1712 {
            tunnel: [w1713 w1715] -> w1711
            tunnel: w1710 -> [w1713 w1715]
            tunnel: w1703 -> [w1714 w1721]
            tunnel: [w1714 w1719] -> w1707
            tunnel: w1706 -> [_ w1717]
            frame False {
            }
            frame True {
              n568 = call <vilib>:"Space Constant.vi"() -> ("String"=w1718:string)
              n569 = Match Pattern(string=w1717, regular expression=w1718) -> (before substring=w1716:string)  [unwired: 1 in, 3 out]
              n570 = Fract/Exp String To Number(string=w1716) -> (number=w1720:dbl)  [unwired: 3 in, 1 out]
              n571 = Bundle By Name(cluster=w1721, "Texp"=w1720) -> (w1719:refnum<class "Channel.lvclass">)
            }
          }
          n572 = Increment(x=w1711) -> (x+1=w1702:i32)
        }
        frame 103 {
          w1729 = "NIMAGES "
          n573 = Unbundle By Name(w1723) -> ("lastStatus"=w1724:string)
          n574 = Match Pattern(string=w1724, regular expression=w1729) -> (match substring=w1728:string, after substring=w1726:string)  [unwired: 1 in, 2 out]
          n575 = Equal?(x=w1728, y=w1729) -> (x = y?=w1732:bool)
          n576 = case shown="True" w1732 {
            tunnel: [w1733 w1735] -> w1731
            tunnel: w1730 -> [w1733 w1735]
            tunnel: w1723 -> [w1734 w1741]
            tunnel: [w1734 w1739] -> w1727
            tunnel: w1726 -> [_ w1737]
            frame False {
            }
            frame True {
              n577 = call <vilib>:"Space Constant.vi"() -> ("String"=w1738:string)
              n578 = Match Pattern(string=w1737, regular expression=w1738) -> (before substring=w1736:string)  [unwired: 1 in, 3 out]
              n579 = Fract/Exp String To Number(string=w1736) -> (number=w1740:dbl)  [unwired: 3 in, 1 out]
              n580 = Bundle By Name(cluster=w1741, "Nimages"=w1740) -> (w1739:refnum<class "Channel.lvclass">)
            }
          }
          n581 = Increment(x=w1731) -> (x+1=w1722:i32)
        }
        frame 104 {
          w1749 = "INITIAL_LINE "
          n582 = Unbundle By Name(w1743) -> ("lastStatus"=w1744:string)
          n583 = Match Pattern(string=w1744, regular expression=w1749) -> (match substring=w1748:string, after substring=w1746:string)  [unwired: 1 in, 2 out]
          n584 = Equal?(x=w1748, y=w1749) -> (x = y?=w1752:bool)
          n585 = case shown="True" w1752 {
            tunnel: [w1753 w1755] -> w1751
            tunnel: w1750 -> [w1753 w1755]
            tunnel: w1743 -> [w1754 w1761]
            tunnel: [w1754 w1759] -> w1747
            tunnel: w1746 -> [_ w1757]
            frame False {
            }
            frame True {
              n586 = call <vilib>:"Space Constant.vi"() -> ("String"=w1758:string)
              n587 = Match Pattern(string=w1757, regular expression=w1758) -> (before substring=w1756:string)  [unwired: 1 in, 3 out]
              n588 = Fract/Exp String To Number(string=w1756) -> (number=w1760:dbl)  [unwired: 3 in, 1 out]
              n589 = Bundle By Name(cluster=w1761, "InitialLine"=w1760) -> (w1759:refnum<class "Channel.lvclass">)
            }
          }
          n590 = Increment(x=w1751) -> (x+1=w1742:i32)
        }
        frame 105 {
          w1769 = "FINAL_LINE "
          n591 = Unbundle By Name(w1763) -> ("lastStatus"=w1764:string)
          n592 = Match Pattern(string=w1764, regular expression=w1769) -> (match substring=w1768:string, after substring=w1766:string)  [unwired: 1 in, 2 out]
          n593 = Equal?(x=w1768, y=w1769) -> (x = y?=w1772:bool)
          n594 = case shown="True" w1772 {
            tunnel: [w1773 w1775] -> w1771
            tunnel: w1770 -> [w1773 w1775]
            tunnel: w1763 -> [w1774 w1781]
            tunnel: [w1774 w1779] -> w1767
            tunnel: w1766 -> [_ w1777]
            frame False {
            }
            frame True {
              n595 = call <vilib>:"Space Constant.vi"() -> ("String"=w1778:string)
              n596 = Match Pattern(string=w1777, regular expression=w1778) -> (before substring=w1776:string)  [unwired: 1 in, 3 out]
              n597 = Fract/Exp String To Number(string=w1776) -> (number=w1780:dbl)  [unwired: 3 in, 1 out]
              n598 = Bundle By Name(cluster=w1781, "FinalLine"=w1780) -> (w1779:refnum<class "Channel.lvclass">)
            }
          }
          n599 = Increment(x=w1771) -> (x+1=w1762:i32)
        }
        frame 106 {
          w1789 = "INITIAL_COLUMN "
          n600 = Unbundle By Name(w1783) -> ("lastStatus"=w1784:string)
          n601 = Match Pattern(string=w1784, regular expression=w1789) -> (match substring=w1788:string, after substring=w1786:string)  [unwired: 1 in, 2 out]
          n602 = Equal?(x=w1788, y=w1789) -> (x = y?=w1792:bool)
          n603 = case shown="True" w1792 {
            tunnel: [w1793 w1795] -> w1791
            tunnel: w1790 -> [w1793 w1795]
            tunnel: w1783 -> [w1794 w1801]
            tunnel: [w1794 w1799] -> w1787
            tunnel: w1786 -> [_ w1797]
            frame False {
            }
            frame True {
              n604 = call <vilib>:"Space Constant.vi"() -> ("String"=w1798:string)
              n605 = Match Pattern(string=w1797, regular expression=w1798) -> (before substring=w1796:string)  [unwired: 1 in, 3 out]
              n606 = Fract/Exp String To Number(string=w1796) -> (number=w1800:dbl)  [unwired: 3 in, 1 out]
              n607 = Bundle By Name(cluster=w1801, "InitialColumn"=w1800) -> (w1799:refnum<class "Channel.lvclass">)
            }
          }
          n608 = Increment(x=w1791) -> (x+1=w1782:i32)
        }
        frame 107 {
          w1809 = "FINAL_COLUMN "
          n609 = Unbundle By Name(w1803) -> ("lastStatus"=w1804:string)
          n610 = Match Pattern(string=w1804, regular expression=w1809) -> (match substring=w1808:string, after substring=w1806:string)  [unwired: 1 in, 2 out]
          n611 = Equal?(x=w1808, y=w1809) -> (x = y?=w1812:bool)
          n612 = case shown="True" w1812 {
            tunnel: [w1813 w1815] -> w1811
            tunnel: w1810 -> [w1813 w1815]
            tunnel: w1803 -> [w1814 w1821]
            tunnel: [w1814 w1819] -> w1807
            tunnel: w1806 -> [_ w1817]
            frame False {
            }
            frame True {
              n613 = call <vilib>:"Space Constant.vi"() -> ("String"=w1818:string)
              n614 = Match Pattern(string=w1817, regular expression=w1818) -> (before substring=w1816:string)  [unwired: 1 in, 3 out]
              n615 = Fract/Exp String To Number(string=w1816) -> (number=w1820:dbl)  [unwired: 3 in, 1 out]
              n616 = Bundle By Name(cluster=w1821, "FinalColumn"=w1820) -> (w1819:refnum<class "Channel.lvclass">)
            }
          }
          n617 = Increment(x=w1811) -> (x+1=w1802:i32)
        }
        frame 108 {
          w1829 = "EM_GAIN "
          n618 = Unbundle By Name(w1823) -> ("lastStatus"=w1824:string)
          n619 = Match Pattern(string=w1824, regular expression=w1829) -> (match substring=w1828:string, after substring=w1826:string)  [unwired: 1 in, 2 out]
          n620 = Equal?(x=w1828, y=w1829) -> (x = y?=w1832:bool)
          n621 = case shown="True" w1832 {
            tunnel: [w1833 w1835] -> w1831
            tunnel: w1830 -> [w1833 w1835]
            tunnel: w1823 -> [w1834 w1841]
            tunnel: [w1834 w1839] -> w1827
            tunnel: w1826 -> [_ w1837]
            frame False {
            }
            frame True {
              n622 = call <vilib>:"Space Constant.vi"() -> ("String"=w1838:string)
              n623 = Match Pattern(string=w1837, regular expression=w1838) -> (before substring=w1836:string)  [unwired: 1 in, 3 out]
              n624 = Fract/Exp String To Number(string=w1836) -> (number=w1840:dbl)  [unwired: 3 in, 1 out]
              n625 = Bundle By Name(cluster=w1841, "EmGain"=w1840) -> (w1839:refnum<class "Channel.lvclass">)
            }
          }
          n626 = Increment(x=w1831) -> (x+1=w1822:i32)
        }
        frame 109 {
          w1849 = "COOLER "
          n627 = Unbundle By Name(w1843) -> ("lastStatus"=w1844:string)
          n628 = Match Pattern(string=w1844, regular expression=w1849) -> (match substring=w1848:string, after substring=w1846:string)  [unwired: 1 in, 2 out]
          n629 = Equal?(x=w1848, y=w1849) -> (x = y?=w1852:bool)
          n630 = case shown="True" w1852 {
            tunnel: [w1853 w1855] -> w1851
            tunnel: w1850 -> [w1853 w1855]
            tunnel: w1843 -> [w1854 w1862]
            tunnel: [w1854 w1861] -> w1847
            tunnel: w1846 -> [_ w1859]
            frame False {
            }
            frame True {
              n631 = call <vilib>:"Space Constant.vi"() -> ("String"=w1860:string)
              n632 = Match Pattern(string=w1859, regular expression=w1860) -> (before substring=w1858:string)  [unwired: 1 in, 3 out]
              n633 = Equal?(x=w1858, y="ON") -> (x = y?=w1856:bool)
              n634 = Bundle By Name(cluster=w1862, "Cooler Off"=w1856) -> (w1861:refnum<class "Channel.lvclass">)
            }
          }
          n635 = Increment(x=w1851) -> (x+1=w1842:i32)
        }
        frame 110 {
        }
        frame 200 {
          n636 = Unbundle By Name(w1874) -> ("Interface.lvclass"=w1873:refnum<class "Interface.lvclass">)
          n637 = call "Read Camera Setup.vi"("Interface in"=w1873) -> ("Camera Setup"=w1867:T4)  [unwired: 8 in, 2 out]
          n638 = Unbundle By Name(w1867) -> ("EXPTIME"=w1866:dbl)
          n639 = Number To Fractional String(number=w1866) -> (F-format string=w1868:string)  [unwired: 3 in]
          n640 = Concatenate Strings("SET EXPTIME " ("cmd"), w1868) -> (w1872:string)
          n641 = call-dynamic "Write cmd.vi"("error in (no error)"=w1876, "cmd"=w1872, "Device in"=w1874) -> ("error out"=w1875:errorcluster, "Device out"=w1877:refnum<class "Channel.lvclass">)  [unwired: 7 in]
          n642 = Increment(x=w1870) -> (x+1=w1871:i32)
        }
        frame 201 {
          n643 = call-dynamic "Read resp.vi"("error in (no error)"=w1885, "Device in"=w1886) -> ("error out"=w1879:errorcluster, "resp"=w1884:string, "Device out"=w1880:refnum<class "Channel.lvclass">)  [unwired: 7 in]
          n644 = Equal?(x=w1884, y="DONE") -> (x = y?=w1882:bool)
          n645 = case shown="True" w1882 {
            tunnel: [w1887 w1888] -> w1881
            tunnel: w1878 -> [w1887 w1889]
            frame False {
            }
            frame True {
              n646 = Increment(x=w1889) -> (x+1=w1888:i32)
            }
          }
        }
        frame 202 {
          n647 = call-dynamic "Write cmd.vi"("error in (no error)"=w1895, "cmd"="GET EXPTIME", "Device in"=w1893) -> ("error out"=w1894:errorcluster, "Device out"=w1896:refnum<class "Channel.lvclass">)  [unwired: 7 in]
          n648 = Increment(x=w1891) -> (x+1=w1892:i32)
        }
        frame 203 {
          n649 = call-dynamic "Read resp.vi"("error in (no error)"=w1907, "Device in"=w1908) -> ("error out"=w1905:errorcluster, "resp"=w1900:string, "Device out"=w1903:refnum<class "Channel.lvclass">)  [unwired: 7 in]
          n650 = Fract/Exp String To Number(string=w1900) -> (number=w1897:dbl)  [unwired: 3 in, 1 out]
          n651 = Unbundle By Name(w1903) -> ("Interface.lvclass"=w1902:refnum<class "Interface.lvclass">)
          n652 = call "Read Camera Setup.vi"("Interface in"=w1902) -> ("Camera Setup"=w1901:T4)  [unwired: 8 in, 2 out]
          n653 = Unbundle By Name(w1901) -> ("EXPTIME"=w1898:dbl)
          n654 = Equal?(x=w1898, y=w1897) -> (x = y?=w1899:bool)
          n655 = disable-structure shown="Enabled" {
            disable-tunnel: [w1911 224 ("State")] -> w1906
            disable-tunnel: w1904 -> [w1910 _]
            disable-tunnel: w1899 -> [w1909 _]
            frame Disabled {
              n656 = case shown="True" w1909 {
                tunnel: [w1912 w1913] -> w1911
                tunnel: w1910 -> [w1912 w1914]
                frame False {
                }
                frame True {
                  n657 = Increment(x=w1914) -> (x+1=w1913:i32)
                }
              }
            }
            frame Enabled {
            }
          }
        }
        frame 204 {
          n658 = Unbundle By Name(w1924) -> ("Interface.lvclass"=w1923:refnum<class "Interface.lvclass">)
          n659 = call "Read Camera Setup.vi"("Interface in"=w1923) -> ("Camera Setup"=w1917:T4)  [unwired: 8 in, 2 out]
          n660 = Unbundle By Name(w1917) -> ("#FRAMES"=w1916:u32)
          n661 = Number To Fractional String(number=w1916) -> (F-format string=w1918:string)  [unwired: 3 in]
          n662 = Concatenate Strings("SET #FRAMES " ("cmd"), w1918) -> (w1922:string)
          n663 = call-dynamic "Write cmd.vi"("error in (no error)"=w1926, "cmd"=w1922, "Device in"=w1924) -> ("error out"=w1925:errorcluster, "Device out"=w1927:refnum<class "Channel.lvclass">)  [unwired: 7 in]
          n664 = Increment(x=w1920) -> (x+1=w1921:i32)
        }
        frame 205 {
          n665 = call-dynamic "Read resp.vi"("error in (no error)"=w1935, "Device in"=w1936) -> ("error out"=w1929:errorcluster, "resp"=w1934:string, "Device out"=w1930:refnum<class "Channel.lvclass">)  [unwired: 7 in]
          n666 = Equal?(x=w1934, y="DONE") -> (x = y?=w1932:bool)
          n667 = case shown="True" w1932 {
            tunnel: [w1937 w1938] -> w1931
            tunnel: w1928 -> [w1937 w1939]
            frame False {
            }
            frame True {
              n668 = Increment(x=w1939) -> (x+1=w1938:i32)
            }
          }
        }
        frame 206 {
          n669 = call-dynamic "Write cmd.vi"("error in (no error)"=w1945, "cmd"="GET #FRAMES", "Device in"=w1943) -> ("error out"=w1944:errorcluster, "Device out"=w1946:refnum<class "Channel.lvclass">)  [unwired: 7 in]
          n670 = Increment(x=w1941) -> (x+1=w1942:i32)
        }
        frame 207 {
          n671 = call-dynamic "Read resp.vi"("error in (no error)"=w1958, "Device in"=w1959) -> ("error out"=w1956:errorcluster, "resp"=w1951:string, "Device out"=w1954:refnum<class "Channel.lvclass">)  [unwired: 7 in]
          n672 = Decimal String To Number(string=w1951) -> (number=w1949:i32)  [unwired: 2 in, 1 out]
          n673 = Unbundle By Name(w1954) -> ("Interface.lvclass"=w1953:refnum<class "Interface.lvclass">)
          n674 = call "Read Camera Setup.vi"("Interface in"=w1953) -> ("Camera Setup"=w1952:T4)  [unwired: 8 in, 2 out]
          n675 = To Unsigned Long Integer(number=w1949) -> (unsigned 32bit integer=w1947:u32)
          n676 = Unbundle By Name(w1952) -> ("#FRAMES"=w1948:u32)
          n677 = Equal?(x=w1948, y=w1947) -> (x = y?=w1950:bool)
          n678 = case shown="True" w1950 {
            tunnel: [w1960 w1961] -> w1957
            tunnel: w1955 -> [w1960 w1962]
            frame False {
            }
            frame True {
              n679 = Increment(x=w1962) -> (x+1=w1961:i32)
            }
          }
        }
        frame 208 {
          n680 = Unbundle By Name(w1971) -> ("Interface.lvclass"=w1970:refnum<class "Interface.lvclass">)
          n681 = call "Read Camera Setup.vi"("Interface in"=w1970) -> ("Camera Setup"=w1964:T4)  [unwired: 8 in, 2 out]
          n682 = Unbundle By Name(w1964) -> ("TRIGGER_MODE"=w1963:u8)
          n683 = Number To Fractional String(number=w1963) -> (F-format string=w1965:string)  [unwired: 3 in]
          n684 = Concatenate Strings("SET TRIGGER_MODE " ("cmd"), w1965) -> (w1969:string)
          n685 = call-dynamic "Write cmd.vi"("error in (no error)"=w1973, "cmd"=w1969, "Device in"=w1971) -> ("error out"=w1972:errorcluster, "Device out"=w1974:refnum<class "Channel.lvclass">)  [unwired: 7 in]
          n686 = Increment(x=w1967) -> (x+1=w1968:i32)
        }
        frame 209 {
          n687 = call-dynamic "Read resp.vi"("error in (no error)"=w1982, "Device in"=w1983) -> ("error out"=w1976:errorcluster, "resp"=w1981:string, "Device out"=w1977:refnum<class "Channel.lvclass">)  [unwired: 7 in]
          n688 = Equal?(x=w1981, y="DONE") -> (x = y?=w1979:bool)
          n689 = case shown="True" w1979 {
            tunnel: [w1984 w1985] -> w1978
            tunnel: w1975 -> [w1984 w1986]
            frame False {
            }
            frame True {
              n690 = Increment(x=w1986) -> (x+1=w1985:i32)
            }
          }
        }
        frame 210 {
          n691 = call-dynamic "Write cmd.vi"("error in (no error)"=w1992, "cmd"="GET TRIGGER_MODE", "Device in"=w1990) -> ("error out"=w1991:errorcluster, "Device out"=w1993:refnum<class "Channel.lvclass">)  [unwired: 7 in]
          n692 = Increment(x=w1988) -> (x+1=w1989:i32)
        }
        frame 211 {
          n693 = call-dynamic "Read resp.vi"("error in (no error)"=w2004, "Device in"=w2005) -> ("error out"=w2002:errorcluster, "resp"=w1997:string, "Device out"=w2000:refnum<class "Channel.lvclass">)  [unwired: 7 in]
          n694 = Fract/Exp String To Number(string=w1997) -> (number=w1995:dbl)  [unwired: 3 in, 1 out]
          n695 = Unbundle By Name(w2000) -> ("Interface.lvclass"=w1999:refnum<class "Interface.lvclass">)
          n696 = call "Read Camera Setup.vi"("Interface in"=w1999) -> ("Camera Setup"=w1998:T4)  [unwired: 8 in, 2 out]
          n697 = Unbundle By Name(w1998) -> ("TRIGGER_MODE"=w1994:u8)
          n698 = Equal?(x=w1994, y=w1995) -> (x = y?=w1996:bool)
          n699 = case shown="False" w1996 {
            tunnel: [w2006 w2007] -> w2003
            tunnel: w2001 -> [w2006 w2008]
            frame False {
            }
            frame True {
              n700 = Increment(x=w2008) -> (x+1=w2007:i32)
            }
          }
        }
        frame 212 {
          n701 = Unbundle By Name(w2017) -> ("Interface.lvclass"=w2016:refnum<class "Interface.lvclass">)
          n702 = call "Read Camera Setup.vi"("Interface in"=w2016) -> ("Camera Setup"=w2010:T4)  [unwired: 8 in, 2 out]
          n703 = Unbundle By Name(w2010) -> ("READ_MODE"=w2009:u8)
          n704 = Number To Fractional String(number=w2009) -> (F-format string=w2011:string)  [unwired: 3 in]
          n705 = Concatenate Strings("SET READ_MODE " ("cmd"), w2011) -> (w2015:string)
          n706 = call-dynamic "Write cmd.vi"("error in (no error)"=w2019, "cmd"=w2015, "Device in"=w2017) -> ("error out"=w2018:errorcluster, "Device out"=w2020:refnum<class "Channel.lvclass">)  [unwired: 7 in]
          n707 = Increment(x=w2013) -> (x+1=w2014:i32)
        }
        frame 213 {
          n708 = call-dynamic "Read resp.vi"("error in (no error)"=w2028, "Device in"=w2029) -> ("error out"=w2022:errorcluster, "resp"=w2027:string, "Device out"=w2023:refnum<class "Channel.lvclass">)  [unwired: 7 in]
          n709 = Equal?(x=w2027, y="DONE") -> (x = y?=w2025:bool)
          n710 = case shown="True" w2025 {
            tunnel: [w2030 w2031] -> w2024
            tunnel: w2021 -> [w2030 w2032]
            frame False {
            }
            frame True {
              n711 = Increment(x=w2032) -> (x+1=w2031:i32)
            }
          }
        }
        frame 214 {
          n712 = call-dynamic "Write cmd.vi"("error in (no error)"=w2038, "cmd"="GET READ_MODE", "Device in"=w2036) -> ("error out"=w2037:errorcluster, "Device out"=w2039:refnum<class "Channel.lvclass">)  [unwired: 7 in]
          n713 = Increment(x=w2034) -> (x+1=w2035:i32)
        }
        frame 215 {
          n714 = call-dynamic "Read resp.vi"("error in (no error)"=w2050, "Device in"=w2051) -> ("error out"=w2048:errorcluster, "resp"=w2043:string, "Device out"=w2046:refnum<class "Channel.lvclass">)  [unwired: 7 in]
          n715 = Fract/Exp String To Number(string=w2043) -> (number=w2041:dbl)  [unwired: 3 in, 1 out]
          n716 = Unbundle By Name(w2046) -> ("Interface.lvclass"=w2045:refnum<class "Interface.lvclass">)
          n717 = call "Read Camera Setup.vi"("Interface in"=w2045) -> ("Camera Setup"=w2044:T4)  [unwired: 8 in, 2 out]
          n718 = Unbundle By Name(w2044) -> ("READ_MODE"=w2040:u8)
          n719 = Equal?(x=w2040, y=w2041) -> (x = y?=w2042:bool)
          n720 = case shown="True" w2042 {
            tunnel: [w2052 w2053] -> w2049
            tunnel: w2047 -> [w2052 w2054]
            frame False {
            }
            frame True {
              n721 = Increment(x=w2054) -> (x+1=w2053:i32)
            }
          }
        }
        frame 216 {
          n722 = Unbundle By Name(w2063) -> ("Interface.lvclass"=w2062:refnum<class "Interface.lvclass">)
          n723 = call "Read Camera Setup.vi"("Interface in"=w2062) -> ("Camera Setup"=w2056:T4)  [unwired: 8 in, 2 out]
          n724 = Unbundle By Name(w2056) -> ("READOUT_RATE"=w2055:u8)
          n725 = Number To Fractional String(number=w2055) -> (F-format string=w2057:string)  [unwired: 3 in]
          n726 = Concatenate Strings("SET READOUT_RATE " ("cmd"), w2057) -> (w2061:string)
          n727 = call-dynamic "Write cmd.vi"("error in (no error)"=w2065, "cmd"=w2061, "Device in"=w2063) -> ("error out"=w2064:errorcluster, "Device out"=w2066:refnum<class "Channel.lvclass">)  [unwired: 7 in]
          n728 = Increment(x=w2059) -> (x+1=w2060:i32)
        }
        frame 217 {
          n729 = call-dynamic "Read resp.vi"("error in (no error)"=w2074, "Device in"=w2075) -> ("error out"=w2068:errorcluster, "resp"=w2073:string, "Device out"=w2069:refnum<class "Channel.lvclass">)  [unwired: 7 in]
          n730 = Equal?(x=w2073, y="DONE") -> (x = y?=w2071:bool)
          n731 = case shown="True" w2071 {
            tunnel: [w2076 w2077] -> w2070
            tunnel: w2067 -> [w2076 w2078]
            frame False {
            }
            frame True {
              n732 = Increment(x=w2078) -> (x+1=w2077:i32)
            }
          }
        }
        frame 218 {
          n733 = call-dynamic "Write cmd.vi"("error in (no error)"=w2084, "cmd"="GET READOUT_RATE", "Device in"=w2082) -> ("error out"=w2083:errorcluster, "Device out"=w2085:refnum<class "Channel.lvclass">)  [unwired: 7 in]
          n734 = Increment(x=w2080) -> (x+1=w2081:i32)
        }
        frame 219 {
          n735 = call-dynamic "Read resp.vi"("error in (no error)"=w2096, "Device in"=w2097) -> ("error out"=w2094:errorcluster, "resp"=w2089:string, "Device out"=w2092:refnum<class "Channel.lvclass">)  [unwired: 7 in]
          n736 = Fract/Exp String To Number(string=w2089) -> (number=w2087:dbl)  [unwired: 3 in, 1 out]
          n737 = Unbundle By Name(w2092) -> ("Interface.lvclass"=w2091:refnum<class "Interface.lvclass">)
          n738 = call "Read Camera Setup.vi"("Interface in"=w2091) -> ("Camera Setup"=w2090:T4)  [unwired: 8 in, 2 out]
          n739 = Unbundle By Name(w2090) -> ("READOUT_RATE"=w2086:u8)
          n740 = Equal?(x=w2086, y=w2087) -> (x = y?=w2088:bool)
          n741 = case shown="True" w2088 {
            tunnel: [w2098 w2099] -> w2095
            tunnel: w2093 -> [w2098 w2100]
            frame False {
            }
            frame True {
              n742 = Increment(x=w2100) -> (x+1=w2099:i32)
            }
          }
        }
        frame 220 {
          n743 = Unbundle By Name(w2109) -> ("Interface.lvclass"=w2108:refnum<class "Interface.lvclass">)
          n744 = call "Read Camera Setup.vi"("Interface in"=w2108) -> ("Camera Setup"=w2102:T4)  [unwired: 8 in, 2 out]
          n745 = Unbundle By Name(w2102) -> ("VERTICAL_SHIFT_SPEED"=w2101:u8)
          n746 = Number To Fractional String(number=w2101) -> (F-format string=w2103:string)  [unwired: 3 in]
          n747 = Concatenate Strings("SET VERTICAL_SHIFT_SPEED " ("cmd"), w2103) -> (w2107:string)
          n748 = call-dynamic "Write cmd.vi"("error in (no error)"=w2111, "cmd"=w2107, "Device in"=w2109) -> ("error out"=w2110:errorcluster, "Device out"=w2112:refnum<class "Channel.lvclass">)  [unwired: 7 in]
          n749 = Increment(x=w2105) -> (x+1=w2106:i32)
        }
        frame 221 {
          n750 = call-dynamic "Read resp.vi"("error in (no error)"=w2120, "Device in"=w2121) -> ("error out"=w2114:errorcluster, "resp"=w2119:string, "Device out"=w2115:refnum<class "Channel.lvclass">)  [unwired: 7 in]
          n751 = Equal?(x=w2119, y="DONE") -> (x = y?=w2117:bool)
          n752 = case shown="True" w2117 {
            tunnel: [w2122 w2123] -> w2116
            tunnel: w2113 -> [w2122 w2124]
            frame False {
            }
            frame True {
              n753 = Increment(x=w2124) -> (x+1=w2123:i32)
            }
          }
        }
        frame 222 {
          n754 = call-dynamic "Write cmd.vi"("error in (no error)"=w2130, "cmd"="GET VERTICAL_SHIFT_SPEED", "Device in"=w2128) -> ("error out"=w2129:errorcluster, "Device out"=w2131:refnum<class "Channel.lvclass">)  [unwired: 7 in]
          n755 = Increment(x=w2126) -> (x+1=w2127:i32)
        }
        frame 223 {
          n756 = call-dynamic "Read resp.vi"("error in (no error)"=w2142, "Device in"=w2143) -> ("error out"=w2140:errorcluster, "resp"=w2135:string, "Device out"=w2138:refnum<class "Channel.lvclass">)  [unwired: 7 in]
          n757 = Fract/Exp String To Number(string=w2135) -> (number=w2133:dbl)  [unwired: 3 in, 1 out]
          n758 = Unbundle By Name(w2138) -> ("Interface.lvclass"=w2137:refnum<class "Interface.lvclass">)
          n759 = call "Read Camera Setup.vi"("Interface in"=w2137) -> ("Camera Setup"=w2136:T4)  [unwired: 8 in, 2 out]
          n760 = Unbundle By Name(w2136) -> ("VERTICAL_SHIFT_SPEED"=w2132:u8)
          n761 = Equal?(x=w2132, y=w2133) -> (x = y?=w2134:bool)
          n762 = case shown="True" w2134 {
            tunnel: [w2144 w2145] -> w2141
            tunnel: w2139 -> [w2144 w2146]
            frame False {
            }
            frame True {
              n763 = Increment(x=w2146) -> (x+1=w2145:i32)
            }
          }
        }
        frame 224 {
          n764 = Unbundle By Name(w2155) -> ("Interface.lvclass"=w2154:refnum<class "Interface.lvclass">)
          n765 = call "Read Camera Setup.vi"("Interface in"=w2154) -> ("Camera Setup"=w2148:T4)  [unwired: 8 in, 2 out]
          n766 = Unbundle By Name(w2148) -> ("PREAMP"=w2147:u8)
          n767 = Number To Fractional String(number=w2147) -> (F-format string=w2149:string)  [unwired: 3 in]
          n768 = Concatenate Strings("SET PREAMP " ("cmd"), w2149) -> (w2153:string)
          n769 = call-dynamic "Write cmd.vi"("error in (no error)"=w2157, "cmd"=w2153, "Device in"=w2155) -> ("error out"=w2156:errorcluster, "Device out"=w2158:refnum<class "Channel.lvclass">)  [unwired: 7 in]
          n770 = Increment(x=w2151) -> (x+1=w2152:i32)
        }
        frame 225 {
          n771 = call-dynamic "Read resp.vi"("error in (no error)"=w2166, "Device in"=w2167) -> ("error out"=w2160:errorcluster, "resp"=w2165:string, "Device out"=w2161:refnum<class "Channel.lvclass">)  [unwired: 7 in]
          n772 = Equal?(x=w2165, y="DONE") -> (x = y?=w2163:bool)
          n773 = case shown="True" w2163 {
            tunnel: [w2168 w2169] -> w2162
            tunnel: w2159 -> [w2168 w2170]
            frame False {
            }
            frame True {
              n774 = Increment(x=w2170) -> (x+1=w2169:i32)
            }
          }
        }
        frame 226 {
          n775 = call-dynamic "Write cmd.vi"("error in (no error)"=w2176, "cmd"="GET PREAMP", "Device in"=w2174) -> ("error out"=w2175:errorcluster, "Device out"=w2177:refnum<class "Channel.lvclass">)  [unwired: 7 in]
          n776 = Increment(x=w2172) -> (x+1=w2173:i32)
        }
        frame 227 {
          n777 = call-dynamic "Read resp.vi"("error in (no error)"=w2188, "Device in"=w2189) -> ("error out"=w2186:errorcluster, "resp"=w2181:string, "Device out"=w2184:refnum<class "Channel.lvclass">)  [unwired: 7 in]
          n778 = Fract/Exp String To Number(string=w2181) -> (number=w2179:dbl)  [unwired: 3 in, 1 out]
          n779 = Unbundle By Name(w2184) -> ("Interface.lvclass"=w2183:refnum<class "Interface.lvclass">)
          n780 = call "Read Camera Setup.vi"("Interface in"=w2183) -> ("Camera Setup"=w2182:T4)  [unwired: 8 in, 2 out]
          n781 = Unbundle By Name(w2182) -> ("PREAMP"=w2178:u8)
          n782 = Equal?(x=w2178, y=w2179) -> (x = y?=w2180:bool)
          n783 = case shown="True" w2180 {
            tunnel: [w2190 w2191] -> w2187
            tunnel: w2185 -> [w2190 w2192]
            frame False {
            }
            frame True {
              n784 = Increment(x=w2192) -> (x+1=w2191:i32)
            }
          }
        }
        frame 228 {
          n785 = Unbundle By Name(w2201) -> ("Interface.lvclass"=w2200:refnum<class "Interface.lvclass">)
          n786 = call "Read Camera Setup.vi"("Interface in"=w2200) -> ("Camera Setup"=w2194:T4)  [unwired: 8 in, 2 out]
          n787 = Unbundle By Name(w2194) -> ("EM_MODE"=w2193:u8)
          n788 = Number To Fractional String(number=w2193) -> (F-format string=w2195:string)  [unwired: 3 in]
          n789 = Concatenate Strings("SET EM_MODE " ("cmd"), w2195) -> (w2199:string)
          n790 = call-dynamic "Write cmd.vi"("error in (no error)"=w2203, "cmd"=w2199, "Device in"=w2201) -> ("error out"=w2202:errorcluster, "Device out"=w2204:refnum<class "Channel.lvclass">)  [unwired: 7 in]
          n791 = Increment(x=w2197) -> (x+1=w2198:i32)
        }
        frame 229 {
          n792 = call-dynamic "Read resp.vi"("error in (no error)"=w2212, "Device in"=w2213) -> ("error out"=w2206:errorcluster, "resp"=w2211:string, "Device out"=w2207:refnum<class "Channel.lvclass">)  [unwired: 7 in]
          n793 = Equal?(x=w2211, y="DONE") -> (x = y?=w2209:bool)
          n794 = case shown="True" w2209 {
            tunnel: [w2214 w2215] -> w2208
            tunnel: w2205 -> [w2214 w2216]
            frame False {
            }
            frame True {
              n795 = Increment(x=w2216) -> (x+1=w2215:i32)
            }
          }
        }
        frame 230 {
          n796 = call-dynamic "Write cmd.vi"("error in (no error)"=w2222, "cmd"="GET EM_MODE", "Device in"=w2220) -> ("error out"=w2221:errorcluster, "Device out"=w2223:refnum<class "Channel.lvclass">)  [unwired: 7 in]
          n797 = Increment(x=w2218) -> (x+1=w2219:i32)
        }
        frame 231 {
          n798 = call-dynamic "Read resp.vi"("error in (no error)"=w2234, "Device in"=w2235) -> ("error out"=w2232:errorcluster, "resp"=w2227:string, "Device out"=w2230:refnum<class "Channel.lvclass">)  [unwired: 7 in]
          n799 = Fract/Exp String To Number(string=w2227) -> (number=w2225:dbl)  [unwired: 3 in, 1 out]
          n800 = Unbundle By Name(w2230) -> ("Interface.lvclass"=w2229:refnum<class "Interface.lvclass">)
          n801 = call "Read Camera Setup.vi"("Interface in"=w2229) -> ("Camera Setup"=w2228:T4)  [unwired: 8 in, 2 out]
          n802 = Unbundle By Name(w2228) -> ("EM_MODE"=w2224:u8)
          n803 = Equal?(x=w2224, y=w2225) -> (x = y?=w2226:bool)
          n804 = case shown="True" w2226 {
            tunnel: [w2236 w2237] -> w2233
            tunnel: w2231 -> [w2236 w2238]
            frame False {
            }
            frame True {
              n805 = Increment(x=w2238) -> (x+1=w2237:i32)
            }
          }
        }
        frame 232 {
          n806 = Unbundle By Name(w2247) -> ("Interface.lvclass"=w2246:refnum<class "Interface.lvclass">)
          n807 = call "Read Camera Setup.vi"("Interface in"=w2246) -> ("Camera Setup"=w2240:T4)  [unwired: 8 in, 2 out]
          n808 = Unbundle By Name(w2240) -> ("EM_GAIN"=w2239:u16)
          n809 = Number To Fractional String(number=w2239) -> (F-format string=w2241:string)  [unwired: 3 in]
          n810 = Concatenate Strings("SET EM_GAIN " ("cmd"), w2241) -> (w2245:string)
          n811 = call-dynamic "Write cmd.vi"("error in (no error)"=w2249, "cmd"=w2245, "Device in"=w2247) -> ("error out"=w2248:errorcluster, "Device out"=w2250:refnum<class "Channel.lvclass">)  [unwired: 7 in]
          n812 = Increment(x=w2243) -> (x+1=w2244:i32)
        }
        frame 233 {
          n813 = call-dynamic "Read resp.vi"("error in (no error)"=w2258, "Device in"=w2259) -> ("error out"=w2252:errorcluster, "resp"=w2257:string, "Device out"=w2253:refnum<class "Channel.lvclass">)  [unwired: 7 in]
          n814 = Equal?(x=w2257, y="DONE") -> (x = y?=w2255:bool)
          n815 = case shown="True" w2255 {
            tunnel: [w2260 w2261] -> w2254
            tunnel: w2251 -> [w2260 w2262]
            frame False {
            }
            frame True {
              n816 = Increment(x=w2262) -> (x+1=w2261:i32)
            }
          }
        }
        frame 234 {
          n817 = call-dynamic "Write cmd.vi"("error in (no error)"=w2268, "cmd"="GET EM_GAIN", "Device in"=w2266) -> ("error out"=w2267:errorcluster, "Device out"=w2269:refnum<class "Channel.lvclass">)  [unwired: 7 in]
          n818 = Increment(x=w2264) -> (x+1=w2265:i32)
        }
        frame 235 {
          n819 = call-dynamic "Read resp.vi"("error in (no error)"=w2280, "Device in"=w2281) -> ("error out"=w2278:errorcluster, "resp"=w2273:string, "Device out"=w2276:refnum<class "Channel.lvclass">)  [unwired: 7 in]
          n820 = Fract/Exp String To Number(string=w2273) -> (number=w2271:dbl)  [unwired: 3 in, 1 out]
          n821 = Unbundle By Name(w2276) -> ("Interface.lvclass"=w2275:refnum<class "Interface.lvclass">)
          n822 = call "Read Camera Setup.vi"("Interface in"=w2275) -> ("Camera Setup"=w2274:T4)  [unwired: 8 in, 2 out]
          n823 = Unbundle By Name(w2274) -> ("EM_GAIN"=w2270:u16)
          n824 = Equal?(x=w2270, y=w2271) -> (x = y?=w2272:bool)
          n825 = disable-structure shown="Enabled" {
            disable-tunnel: [w2284 264 ("State")] -> w2279
            disable-tunnel: w2277 -> [w2283 _]
            disable-tunnel: w2272 -> [w2282 _]
            frame Disabled {
              n826 = case shown="True" w2282 {
                tunnel: [w2285 w2286] -> w2284
                tunnel: w2283 -> [w2285 w2287]
                frame False {
                }
                frame True {
                  n827 = Increment(x=w2287) -> (x+1=w2286:i32)
                }
              }
            }
            frame Enabled {
            }
          }
        }
        frame 236 {
          n828 = Unbundle By Name(w2297) -> ("Interface.lvclass"=w2296:refnum<class "Interface.lvclass">)
          n829 = call "Read Camera Setup.vi"("Interface in"=w2296) -> ("Camera Setup"=w2290:T4)  [unwired: 8 in, 2 out]
          n830 = Unbundle By Name(w2290) -> ("ACQUISITION_MODE"=w2289:u8)
          n831 = Number To Fractional String(number=w2289) -> (F-format string=w2291:string)  [unwired: 3 in]
          n832 = Concatenate Strings("SET ACQUISITION_MODE " ("cmd"), w2291) -> (w2295:string)
          n833 = call-dynamic "Write cmd.vi"("error in (no error)"=w2299, "cmd"=w2295, "Device in"=w2297) -> ("error out"=w2298:errorcluster, "Device out"=w2300:refnum<class "Channel.lvclass">)  [unwired: 7 in]
          n834 = Increment(x=w2293) -> (x+1=w2294:i32)
        }
        frame 237 {
          n835 = call-dynamic "Read resp.vi"("error in (no error)"=w2308, "Device in"=w2309) -> ("error out"=w2302:errorcluster, "resp"=w2307:string, "Device out"=w2303:refnum<class "Channel.lvclass">)  [unwired: 7 in]
          n836 = Equal?(x=w2307, y="DONE") -> (x = y?=w2305:bool)
          n837 = case shown="True" w2305 {
            tunnel: [w2310 w2311] -> w2304
            tunnel: w2301 -> [w2310 w2312]
            frame False {
            }
            frame True {
              n838 = Increment(x=w2312) -> (x+1=w2311:i32)
            }
          }
        }
        frame 238 {
          n839 = call-dynamic "Write cmd.vi"("error in (no error)"=w2318, "cmd"="GET ACQUISITION_MODE", "Device in"=w2316) -> ("error out"=w2317:errorcluster, "Device out"=w2319:refnum<class "Channel.lvclass">)  [unwired: 7 in]
          n840 = Increment(x=w2314) -> (x+1=w2315:i32)
        }
        frame 239 {
          n841 = call-dynamic "Read resp.vi"("error in (no error)"=w2330, "Device in"=w2331) -> ("error out"=w2328:errorcluster, "resp"=w2323:string, "Device out"=w2326:refnum<class "Channel.lvclass">)  [unwired: 7 in]
          n842 = Fract/Exp String To Number(string=w2323) -> (number=w2321:dbl)  [unwired: 3 in, 1 out]
          n843 = Unbundle By Name(w2326) -> ("Interface.lvclass"=w2325:refnum<class "Interface.lvclass">)
          n844 = call "Read Camera Setup.vi"("Interface in"=w2325) -> ("Camera Setup"=w2324:T4)  [unwired: 8 in, 2 out]
          n845 = Unbundle By Name(w2324) -> ("ACQUISITION_MODE"=w2320:u8)
          n846 = Equal?(x=w2320, y=w2321) -> (x = y?=w2322:bool)
          n847 = case shown="True" w2322 {
            tunnel: [w2332 w2333] -> w2329
            tunnel: w2327 -> [w2332 w2334]
            frame False {
            }
            frame True {
              n848 = Increment(x=w2334) -> (x+1=w2333:i32)
            }
          }
        }
        frame 240 {
          n849 = Unbundle By Name(w2343) -> ("Interface.lvclass"=w2342:refnum<class "Interface.lvclass">)
          n850 = call "Read Camera Setup.vi"("Interface in"=w2342) -> ("Camera Setup"=w2336:T4)  [unwired: 8 in, 2 out]
          n851 = Unbundle By Name(w2336) -> ("SHUTTER_MODE"=w2335:u8)
          n852 = Number To Fractional String(number=w2335) -> (F-format string=w2337:string)  [unwired: 3 in]
          n853 = Concatenate Strings("SET SHUTTER_MODE " ("cmd"), w2337) -> (w2341:string)
          n854 = call-dynamic "Write cmd.vi"("error in (no error)"=w2345, "cmd"=w2341, "Device in"=w2343) -> ("error out"=w2344:errorcluster, "Device out"=w2346:refnum<class "Channel.lvclass">)  [unwired: 7 in]
          n855 = Increment(x=w2339) -> (x+1=w2340:i32)
        }
        frame 241 {
          n856 = call-dynamic "Read resp.vi"("error in (no error)"=w2354, "Device in"=w2355) -> ("error out"=w2348:errorcluster, "resp"=w2353:string, "Device out"=w2349:refnum<class "Channel.lvclass">)  [unwired: 7 in]
          n857 = Equal?(x=w2353, y="DONE") -> (x = y?=w2351:bool)
          n858 = case shown="True" w2351 {
            tunnel: [w2356 w2357] -> w2350
            tunnel: w2347 -> [w2356 w2358]
            frame False {
            }
            frame True {
              n859 = Increment(x=w2358) -> (x+1=w2357:i32)
            }
          }
        }
        frame 242 {
          n860 = call-dynamic "Write cmd.vi"("error in (no error)"=w2364, "cmd"="GET SHUTTER_MODE", "Device in"=w2362) -> ("error out"=w2363:errorcluster, "Device out"=w2365:refnum<class "Channel.lvclass">)  [unwired: 7 in]
          n861 = Increment(x=w2360) -> (x+1=w2361:i32)
        }
        frame 243 {
          n862 = call-dynamic "Read resp.vi"("error in (no error)"=w2376, "Device in"=w2377) -> ("error out"=w2374:errorcluster, "resp"=w2369:string, "Device out"=w2372:refnum<class "Channel.lvclass">)  [unwired: 7 in]
          n863 = Fract/Exp String To Number(string=w2369) -> (number=w2367:dbl)  [unwired: 3 in, 1 out]
          n864 = Unbundle By Name(w2372) -> ("Interface.lvclass"=w2371:refnum<class "Interface.lvclass">)
          n865 = call "Read Camera Setup.vi"("Interface in"=w2371) -> ("Camera Setup"=w2370:T4)  [unwired: 8 in, 2 out]
          n866 = Unbundle By Name(w2370) -> ("SHUTTER_MODE"=w2366:u8)
          n867 = Equal?(x=w2366, y=w2367) -> (x = y?=w2368:bool)
          n868 = case shown="True" w2368 {
            tunnel: [w2378 w2379] -> w2375
            tunnel: w2373 -> [w2378 w2380]
            frame False {
            }
            frame True {
              n869 = Increment(x=w2380) -> (x+1=w2379:i32)
            }
          }
        }
        frame 244 {
          n870 = Unbundle By Name(w2389) -> ("Interface.lvclass"=w2388:refnum<class "Interface.lvclass">)
          n871 = call "Read Camera Setup.vi"("Interface in"=w2388) -> ("Camera Setup"=w2382:T4)  [unwired: 8 in, 2 out]
          n872 = Unbundle By Name(w2382) -> ("SHUTTER_TTL"=w2381:u8)
          n873 = Number To Fractional String(number=w2381) -> (F-format string=w2383:string)  [unwired: 3 in]
          n874 = Concatenate Strings("SET SHUTTER_TTL " ("cmd"), w2383) -> (w2387:string)
          n875 = call-dynamic "Write cmd.vi"("error in (no error)"=w2391, "cmd"=w2387, "Device in"=w2389) -> ("error out"=w2390:errorcluster, "Device out"=w2392:refnum<class "Channel.lvclass">)  [unwired: 7 in]
          n876 = Increment(x=w2385) -> (x+1=w2386:i32)
        }
        frame 245 {
          n877 = call-dynamic "Read resp.vi"("error in (no error)"=w2400, "Device in"=w2401) -> ("error out"=w2394:errorcluster, "resp"=w2399:string, "Device out"=w2395:refnum<class "Channel.lvclass">)  [unwired: 7 in]
          n878 = Equal?(x=w2399, y="DONE") -> (x = y?=w2397:bool)
          n879 = case shown="True" w2397 {
            tunnel: [w2402 w2403] -> w2396
            tunnel: w2393 -> [w2402 w2404]
            frame False {
            }
            frame True {
              n880 = Increment(x=w2404) -> (x+1=w2403:i32)
            }
          }
        }
        frame 246 {
          n881 = call-dynamic "Write cmd.vi"("error in (no error)"=w2410, "cmd"="GET SHUTTER_TTL", "Device in"=w2408) -> ("error out"=w2409:errorcluster, "Device out"=w2411:refnum<class "Channel.lvclass">)  [unwired: 7 in]
          n882 = Increment(x=w2406) -> (x+1=w2407:i32)
        }
        frame 247 {
          n883 = call-dynamic "Read resp.vi"("error in (no error)"=w2422, "Device in"=w2423) -> ("error out"=w2420:errorcluster, "resp"=w2415:string, "Device out"=w2418:refnum<class "Channel.lvclass">)  [unwired: 7 in]
          n884 = Fract/Exp String To Number(string=w2415) -> (number=w2413:dbl)  [unwired: 3 in, 1 out]
          n885 = Unbundle By Name(w2418) -> ("Interface.lvclass"=w2417:refnum<class "Interface.lvclass">)
          n886 = call "Read Camera Setup.vi"("Interface in"=w2417) -> ("Camera Setup"=w2416:T4)  [unwired: 8 in, 2 out]
          n887 = Unbundle By Name(w2416) -> ("SHUTTER_TTL"=w2412:u8)
          n888 = Equal?(x=w2412, y=w2413) -> (x = y?=w2414:bool)
          n889 = case shown="True" w2414 {
            tunnel: [w2424 w2425] -> w2421
            tunnel: w2419 -> [w2424 w2426]
            frame False {
            }
            frame True {
              n890 = Increment(x=w2426) -> (x+1=w2425:i32)
            }
          }
        }
        frame 248 {
          n891 = Unbundle By Name(w2435) -> ("Interface.lvclass"=w2434:refnum<class "Interface.lvclass">)
          n892 = call "Read Camera Setup.vi"("Interface in"=w2434) -> ("Camera Setup"=w2428:T4)  [unwired: 8 in, 2 out]
          n893 = Unbundle By Name(w2428) -> ("SHUTTER_OPENNING_TIME"=w2427:u16)
          n894 = Number To Fractional String(number=w2427) -> (F-format string=w2429:string)  [unwired: 3 in]
          n895 = Concatenate Strings("SET SHUTTER_OPENNING_TIME " ("cmd"), w2429) -> (w2433:string)
          n896 = call-dynamic "Write cmd.vi"("error in (no error)"=w2437, "cmd"=w2433, "Device in"=w2435) -> ("error out"=w2436:errorcluster, "Device out"=w2438:refnum<class "Channel.lvclass">)  [unwired: 7 in]
          n897 = Increment(x=w2431) -> (x+1=w2432:i32)
        }
        frame 249 {
          n898 = call-dynamic "Read resp.vi"("error in (no error)"=w2446, "Device in"=w2447) -> ("error out"=w2440:errorcluster, "resp"=w2445:string, "Device out"=w2441:refnum<class "Channel.lvclass">)  [unwired: 7 in]
          n899 = Equal?(x=w2445, y="DONE") -> (x = y?=w2443:bool)
          n900 = case shown="True" w2443 {
            tunnel: [w2448 w2449] -> w2442
            tunnel: w2439 -> [w2448 w2450]
            frame False {
            }
            frame True {
              n901 = Increment(x=w2450) -> (x+1=w2449:i32)
            }
          }
        }
        frame 250 {
          n902 = call-dynamic "Write cmd.vi"("error in (no error)"=w2456, "cmd"="GET SHUTTER_OPENNING_TIME", "Device in"=w2454) -> ("error out"=w2455:errorcluster, "Device out"=w2457:refnum<class "Channel.lvclass">)  [unwired: 7 in]
          n903 = Increment(x=w2452) -> (x+1=w2453:i32)
        }
        frame 251 {
          n904 = call-dynamic "Read resp.vi"("error in (no error)"=w2468, "Device in"=w2469) -> ("error out"=w2466:errorcluster, "resp"=w2461:string, "Device out"=w2464:refnum<class "Channel.lvclass">)  [unwired: 7 in]
          n905 = Fract/Exp String To Number(string=w2461) -> (number=w2459:dbl)  [unwired: 3 in, 1 out]
          n906 = Unbundle By Name(w2464) -> ("Interface.lvclass"=w2463:refnum<class "Interface.lvclass">)
          n907 = call "Read Camera Setup.vi"("Interface in"=w2463) -> ("Camera Setup"=w2462:T4)  [unwired: 8 in, 2 out]
          n908 = Unbundle By Name(w2462) -> ("SHUTTER_OPENNING_TIME"=w2458:u16)
          n909 = Equal?(x=w2458, y=w2459) -> (x = y?=w2460:bool)
          n910 = case shown="True" w2460 {
            tunnel: [w2470 w2471] -> w2467
            tunnel: w2465 -> [w2470 w2472]
            frame False {
            }
            frame True {
              n911 = Increment(x=w2472) -> (x+1=w2471:i32)
            }
          }
        }
        frame 252 {
          n912 = Unbundle By Name(w2481) -> ("Interface.lvclass"=w2480:refnum<class "Interface.lvclass">)
          n913 = call "Read Camera Setup.vi"("Interface in"=w2480) -> ("Camera Setup"=w2474:T4)  [unwired: 8 in, 2 out]
          n914 = Unbundle By Name(w2474) -> ("SHUTTER_CLOSING_TIME"=w2473:u16)
          n915 = Number To Fractional String(number=w2473) -> (F-format string=w2475:string)  [unwired: 3 in]
          n916 = Concatenate Strings("SET SHUTTER_CLOSING_TIME " ("cmd"), w2475) -> (w2479:string)
          n917 = call-dynamic "Write cmd.vi"("error in (no error)"=w2483, "cmd"=w2479, "Device in"=w2481) -> ("error out"=w2482:errorcluster, "Device out"=w2484:refnum<class "Channel.lvclass">)  [unwired: 7 in]
          n918 = Increment(x=w2477) -> (x+1=w2478:i32)
        }
        frame 253 {
          n919 = call-dynamic "Read resp.vi"("error in (no error)"=w2492, "Device in"=w2493) -> ("error out"=w2486:errorcluster, "resp"=w2491:string, "Device out"=w2487:refnum<class "Channel.lvclass">)  [unwired: 7 in]
          n920 = Equal?(x=w2491, y="DONE") -> (x = y?=w2489:bool)
          n921 = case shown="True" w2489 {
            tunnel: [w2494 w2495] -> w2488
            tunnel: w2485 -> [w2494 w2496]
            frame False {
            }
            frame True {
              n922 = Increment(x=w2496) -> (x+1=w2495:i32)
            }
          }
        }
        frame 254 {
          n923 = call-dynamic "Write cmd.vi"("error in (no error)"=w2502, "cmd"="GET SHUTTER_CLOSING_TIME", "Device in"=w2500) -> ("error out"=w2501:errorcluster, "Device out"=w2503:refnum<class "Channel.lvclass">)  [unwired: 7 in]
          n924 = Increment(x=w2498) -> (x+1=w2499:i32)
        }
        frame 255 {
          n925 = call-dynamic "Read resp.vi"("error in (no error)"=w2514, "Device in"=w2515) -> ("error out"=w2512:errorcluster, "resp"=w2507:string, "Device out"=w2510:refnum<class "Channel.lvclass">)  [unwired: 7 in]
          n926 = Fract/Exp String To Number(string=w2507) -> (number=w2505:dbl)  [unwired: 3 in, 1 out]
          n927 = Unbundle By Name(w2510) -> ("Interface.lvclass"=w2509:refnum<class "Interface.lvclass">)
          n928 = call "Read Camera Setup.vi"("Interface in"=w2509) -> ("Camera Setup"=w2508:T4)  [unwired: 8 in, 2 out]
          n929 = Unbundle By Name(w2508) -> ("SHUTTER_CLOSING_TIME"=w2504:u16)
          n930 = Equal?(x=w2504, y=w2505) -> (x = y?=w2506:bool)
          n931 = case shown="True" w2506 {
            tunnel: [w2516 w2517] -> w2513
            tunnel: w2511 -> [w2516 w2518]
            frame False {
            }
            frame True {
              n932 = Increment(x=w2518) -> (x+1=w2517:i32)
            }
          }
        }
        frame 256 {
          n933 = Unbundle By Name(w2527) -> ("Interface.lvclass"=w2526:refnum<class "Interface.lvclass">)
          n934 = call "Read Camera Setup.vi"("Interface in"=w2526) -> ("Camera Setup"=w2520:T4)  [unwired: 8 in, 2 out]
          n935 = Unbundle By Name(w2520) -> ("HBIN"=w2519:u16)
          n936 = Number To Fractional String(number=w2519) -> (F-format string=w2521:string)  [unwired: 3 in]
          n937 = Concatenate Strings("SET HBIN " ("cmd"), w2521) -> (w2525:string)
          n938 = call-dynamic "Write cmd.vi"("error in (no error)"=w2529, "cmd"=w2525, "Device in"=w2527) -> ("error out"=w2528:errorcluster, "Device out"=w2530:refnum<class "Channel.lvclass">)  [unwired: 7 in]
          n939 = Increment(x=w2523) -> (x+1=w2524:i32)
        }
        frame 257 {
          n940 = call-dynamic "Read resp.vi"("error in (no error)"=w2538, "Device in"=w2539) -> ("error out"=w2532:errorcluster, "resp"=w2537:string, "Device out"=w2533:refnum<class "Channel.lvclass">)  [unwired: 7 in]
          n941 = Equal?(x=w2537, y="DONE") -> (x = y?=w2535:bool)
          n942 = case shown="True" w2535 {
            tunnel: [w2540 w2541] -> w2534
            tunnel: w2531 -> [w2540 w2542]
            frame False {
            }
            frame True {
              n943 = Increment(x=w2542) -> (x+1=w2541:i32)
            }
          }
        }
        frame 258 {
          n944 = call-dynamic "Write cmd.vi"("error in (no error)"=w2548, "cmd"="GET HBIN", "Device in"=w2546) -> ("error out"=w2547:errorcluster, "Device out"=w2549:refnum<class "Channel.lvclass">)  [unwired: 7 in]
          n945 = Increment(x=w2544) -> (x+1=w2545:i32)
        }
        frame 259 {
          n946 = call-dynamic "Read resp.vi"("error in (no error)"=w2560, "Device in"=w2561) -> ("error out"=w2558:errorcluster, "resp"=w2553:string, "Device out"=w2556:refnum<class "Channel.lvclass">)  [unwired: 7 in]
          n947 = Fract/Exp String To Number(string=w2553) -> (number=w2551:dbl)  [unwired: 3 in, 1 out]
          n948 = Unbundle By Name(w2556) -> ("Interface.lvclass"=w2555:refnum<class "Interface.lvclass">)
          n949 = call "Read Camera Setup.vi"("Interface in"=w2555) -> ("Camera Setup"=w2554:T4)  [unwired: 8 in, 2 out]
          n950 = Unbundle By Name(w2554) -> ("HBIN"=w2550:u16)
          n951 = Equal?(x=w2550, y=w2551) -> (x = y?=w2552:bool)
          n952 = case shown="True" w2552 {
            tunnel: [w2562 w2563] -> w2559
            tunnel: w2557 -> [w2562 w2564]
            frame False {
            }
            frame True {
              n953 = Increment(x=w2564) -> (x+1=w2563:i32)
            }
          }
        }
        frame 260 {
          n954 = Unbundle By Name(w2573) -> ("Interface.lvclass"=w2572:refnum<class "Interface.lvclass">)
          n955 = call "Read Camera Setup.vi"("Interface in"=w2572) -> ("Camera Setup"=w2566:T4)  [unwired: 8 in, 2 out]
          n956 = Unbundle By Name(w2566) -> ("VBIN"=w2565:u16)
          n957 = Number To Fractional String(number=w2565) -> (F-format string=w2567:string)  [unwired: 3 in]
          n958 = Concatenate Strings("SET VBIN " ("cmd"), w2567) -> (w2571:string)
          n959 = call-dynamic "Write cmd.vi"("error in (no error)"=w2575, "cmd"=w2571, "Device in"=w2573) -> ("error out"=w2574:errorcluster, "Device out"=w2576:refnum<class "Channel.lvclass">)  [unwired: 7 in]
          n960 = Increment(x=w2569) -> (x+1=w2570:i32)
        }
        frame 261 {
          n961 = call-dynamic "Read resp.vi"("error in (no error)"=w2584, "Device in"=w2585) -> ("error out"=w2578:errorcluster, "resp"=w2583:string, "Device out"=w2579:refnum<class "Channel.lvclass">)  [unwired: 7 in]
          n962 = Equal?(x=w2583, y="DONE") -> (x = y?=w2581:bool)
          n963 = case shown="True" w2581 {
            tunnel: [w2586 w2587] -> w2580
            tunnel: w2577 -> [w2586 w2588]
            frame False {
            }
            frame True {
              n964 = Increment(x=w2588) -> (x+1=w2587:i32)
            }
          }
        }
        frame 262 {
          n965 = call-dynamic "Write cmd.vi"("error in (no error)"=w2594, "cmd"="GET VBIN", "Device in"=w2592) -> ("error out"=w2593:errorcluster, "Device out"=w2595:refnum<class "Channel.lvclass">)  [unwired: 7 in]
          n966 = Increment(x=w2590) -> (x+1=w2591:i32)
        }
        frame 263 {
          n967 = call-dynamic "Read resp.vi"("error in (no error)"=w2606, "Device in"=w2607) -> ("error out"=w2604:errorcluster, "resp"=w2599:string, "Device out"=w2602:refnum<class "Channel.lvclass">)  [unwired: 7 in]
          n968 = Fract/Exp String To Number(string=w2599) -> (number=w2597:dbl)  [unwired: 3 in, 1 out]
          n969 = Unbundle By Name(w2602) -> ("Interface.lvclass"=w2601:refnum<class "Interface.lvclass">)
          n970 = call "Read Camera Setup.vi"("Interface in"=w2601) -> ("Camera Setup"=w2600:T4)  [unwired: 8 in, 2 out]
          n971 = Unbundle By Name(w2600) -> ("VBIN"=w2596:u16)
          n972 = Equal?(x=w2596, y=w2597) -> (x = y?=w2598:bool)
          n973 = case shown="True" w2598 {
            tunnel: [w2608 w2609] -> w2605
            tunnel: w2603 -> [w2608 w2610]
            frame False {
            }
            frame True {
              n974 = Increment(x=w2610) -> (x+1=w2609:i32)
            }
          }
        }
        frame 264 {
          n975 = Unbundle By Name(w2619) -> ("Interface.lvclass"=w2618:refnum<class "Interface.lvclass">)
          n976 = call "Read Camera Setup.vi"("Interface in"=w2618) -> ("Camera Setup"=w2612:T4)  [unwired: 8 in, 2 out]
          n977 = Unbundle By Name(w2612) -> ("INITIAL_LINE"=w2611:u16)
          n978 = Number To Fractional String(number=w2611) -> (F-format string=w2613:string)  [unwired: 3 in]
          n979 = Concatenate Strings("SET INITIAL_LINE " ("cmd"), w2613) -> (w2617:string)
          n980 = call-dynamic "Write cmd.vi"("error in (no error)"=w2621, "cmd"=w2617, "Device in"=w2619) -> ("error out"=w2620:errorcluster, "Device out"=w2622:refnum<class "Channel.lvclass">)  [unwired: 7 in]
          n981 = Increment(x=w2615) -> (x+1=w2616:i32)
        }
        frame 265 {
          n982 = call-dynamic "Read resp.vi"("error in (no error)"=w2630, "Device in"=w2631) -> ("error out"=w2624:errorcluster, "resp"=w2629:string, "Device out"=w2625:refnum<class "Channel.lvclass">)  [unwired: 7 in]
          n983 = Equal?(x=w2629, y="DONE") -> (x = y?=w2627:bool)
          n984 = case shown="True" w2627 {
            tunnel: [w2632 w2633] -> w2626
            tunnel: w2623 -> [w2632 w2634]
            frame False {
            }
            frame True {
              n985 = Increment(x=w2634) -> (x+1=w2633:i32)
            }
          }
        }
        frame 266 {
          n986 = call-dynamic "Write cmd.vi"("error in (no error)"=w2640, "cmd"="GET INITIAL_LINE", "Device in"=w2638) -> ("error out"=w2639:errorcluster, "Device out"=w2641:refnum<class "Channel.lvclass">)  [unwired: 7 in]
          n987 = Increment(x=w2636) -> (x+1=w2637:i32)
        }
        frame 267 {
          n988 = call-dynamic "Read resp.vi"("error in (no error)"=w2652, "Device in"=w2653) -> ("error out"=w2650:errorcluster, "resp"=w2645:string, "Device out"=w2648:refnum<class "Channel.lvclass">)  [unwired: 7 in]
          n989 = Fract/Exp String To Number(string=w2645) -> (number=w2643:dbl)  [unwired: 3 in, 1 out]
          n990 = Unbundle By Name(w2648) -> ("Interface.lvclass"=w2647:refnum<class "Interface.lvclass">)
          n991 = call "Read Camera Setup.vi"("Interface in"=w2647) -> ("Camera Setup"=w2646:T4)  [unwired: 8 in, 2 out]
          n992 = Unbundle By Name(w2646) -> ("INITIAL_LINE"=w2642:u16)
          n993 = Equal?(x=w2642, y=w2643) -> (x = y?=w2644:bool)
          n994 = case shown="True" w2644 {
            tunnel: [w2654 w2655] -> w2651
            tunnel: w2649 -> [w2654 w2656]
            frame False {
            }
            frame True {
              n995 = Increment(x=w2656) -> (x+1=w2655:i32)
            }
          }
        }
        frame 268 {
          n996 = Unbundle By Name(w2665) -> ("Interface.lvclass"=w2664:refnum<class "Interface.lvclass">)
          n997 = call "Read Camera Setup.vi"("Interface in"=w2664) -> ("Camera Setup"=w2658:T4)  [unwired: 8 in, 2 out]
          n998 = Unbundle By Name(w2658) -> ("INITIAL_COLUMN"=w2657:u16)
          n999 = Number To Fractional String(number=w2657) -> (F-format string=w2659:string)  [unwired: 3 in]
          n1000 = Concatenate Strings("SET INITIAL_COLUMN " ("cmd"), w2659) -> (w2663:string)
          n1001 = call-dynamic "Write cmd.vi"("error in (no error)"=w2667, "cmd"=w2663, "Device in"=w2665) -> ("error out"=w2666:errorcluster, "Device out"=w2668:refnum<class "Channel.lvclass">)  [unwired: 7 in]
          n1002 = Increment(x=w2661) -> (x+1=w2662:i32)
        }
        frame 269 {
          n1003 = call-dynamic "Read resp.vi"("error in (no error)"=w2676, "Device in"=w2677) -> ("error out"=w2670:errorcluster, "resp"=w2675:string, "Device out"=w2671:refnum<class "Channel.lvclass">)  [unwired: 7 in]
          n1004 = Equal?(x=w2675, y="DONE") -> (x = y?=w2673:bool)
          n1005 = case shown="True" w2673 {
            tunnel: [w2678 w2679] -> w2672
            tunnel: w2669 -> [w2678 w2680]
            frame False {
            }
            frame True {
              n1006 = Increment(x=w2680) -> (x+1=w2679:i32)
            }
          }
        }
        frame 270 {
          n1007 = call-dynamic "Write cmd.vi"("error in (no error)"=w2686, "cmd"="GET INITIAL_COLUMN", "Device in"=w2684) -> ("error out"=w2685:errorcluster, "Device out"=w2687:refnum<class "Channel.lvclass">)  [unwired: 7 in]
          n1008 = Increment(x=w2682) -> (x+1=w2683:i32)
        }
        frame 271 {
          n1009 = call-dynamic "Read resp.vi"("error in (no error)"=w2698, "Device in"=w2699) -> ("error out"=w2696:errorcluster, "resp"=w2691:string, "Device out"=w2694:refnum<class "Channel.lvclass">)  [unwired: 7 in]
          n1010 = Fract/Exp String To Number(string=w2691) -> (number=w2689:dbl)  [unwired: 3 in, 1 out]
          n1011 = Unbundle By Name(w2694) -> ("Interface.lvclass"=w2693:refnum<class "Interface.lvclass">)
          n1012 = call "Read Camera Setup.vi"("Interface in"=w2693) -> ("Camera Setup"=w2692:T4)  [unwired: 8 in, 2 out]
          n1013 = Unbundle By Name(w2692) -> ("INITIAL_COLUMN"=w2688:u16)
          n1014 = Equal?(x=w2688, y=w2689) -> (x = y?=w2690:bool)
          n1015 = case shown="True" w2690 {
            tunnel: [w2700 w2701] -> w2697
            tunnel: w2695 -> [w2700 w2702]
            frame False {
            }
            frame True {
              n1016 = Increment(x=w2702) -> (x+1=w2701:i32)
            }
          }
        }
        frame 272 {
          n1017 = Unbundle By Name(w2711) -> ("Interface.lvclass"=w2710:refnum<class "Interface.lvclass">)
          n1018 = call "Read Camera Setup.vi"("Interface in"=w2710) -> ("Camera Setup"=w2704:T4)  [unwired: 8 in, 2 out]
          n1019 = Unbundle By Name(w2704) -> ("FINAL_LINE"=w2703:u16)
          n1020 = Number To Fractional String(number=w2703) -> (F-format string=w2705:string)  [unwired: 3 in]
          n1021 = Concatenate Strings("SET FINAL_LINE " ("cmd"), w2705) -> (w2709:string)
          n1022 = call-dynamic "Write cmd.vi"("error in (no error)"=w2713, "cmd"=w2709, "Device in"=w2711) -> ("error out"=w2712:errorcluster, "Device out"=w2714:refnum<class "Channel.lvclass">)  [unwired: 7 in]
          n1023 = Increment(x=w2707) -> (x+1=w2708:i32)
        }
        frame 273 {
          n1024 = call-dynamic "Read resp.vi"("error in (no error)"=w2722, "Device in"=w2723) -> ("error out"=w2716:errorcluster, "resp"=w2721:string, "Device out"=w2717:refnum<class "Channel.lvclass">)  [unwired: 7 in]
          n1025 = Equal?(x=w2721, y="DONE") -> (x = y?=w2719:bool)
          n1026 = case shown="True" w2719 {
            tunnel: [w2724 w2725] -> w2718
            tunnel: w2715 -> [w2724 w2726]
            frame False {
            }
            frame True {
              n1027 = Increment(x=w2726) -> (x+1=w2725:i32)
            }
          }
        }
        frame 274 {
          n1028 = call-dynamic "Write cmd.vi"("error in (no error)"=w2732, "cmd"="GET FINAL_LINE", "Device in"=w2730) -> ("error out"=w2731:errorcluster, "Device out"=w2733:refnum<class "Channel.lvclass">)  [unwired: 7 in]
          n1029 = Increment(x=w2728) -> (x+1=w2729:i32)
        }
        frame 275 {
          n1030 = call-dynamic "Read resp.vi"("error in (no error)"=w2744, "Device in"=w2745) -> ("error out"=w2742:errorcluster, "resp"=w2737:string, "Device out"=w2740:refnum<class "Channel.lvclass">)  [unwired: 7 in]
          n1031 = Fract/Exp String To Number(string=w2737) -> (number=w2735:dbl)  [unwired: 3 in, 1 out]
          n1032 = Unbundle By Name(w2740) -> ("Interface.lvclass"=w2739:refnum<class "Interface.lvclass">)
          n1033 = call "Read Camera Setup.vi"("Interface in"=w2739) -> ("Camera Setup"=w2738:T4)  [unwired: 8 in, 2 out]
          n1034 = Unbundle By Name(w2738) -> ("FINAL_LINE"=w2734:u16)
          n1035 = Equal?(x=w2734, y=w2735) -> (x = y?=w2736:bool)
          n1036 = case shown="True" w2736 {
            tunnel: [w2746 w2747] -> w2743
            tunnel: w2741 -> [w2746 w2748]
            frame False {
            }
            frame True {
              n1037 = Increment(x=w2748) -> (x+1=w2747:i32)
            }
          }
        }
        frame 276 {
          n1038 = Unbundle By Name(w2757) -> ("Interface.lvclass"=w2756:refnum<class "Interface.lvclass">)
          n1039 = call "Read Camera Setup.vi"("Interface in"=w2756) -> ("Camera Setup"=w2750:T4)  [unwired: 8 in, 2 out]
          n1040 = Unbundle By Name(w2750) -> ("FINAL_COLUMN"=w2749:u16)
          n1041 = Number To Fractional String(number=w2749) -> (F-format string=w2751:string)  [unwired: 3 in]
          n1042 = Concatenate Strings("SET FINAL_COLUMN " ("cmd"), w2751) -> (w2755:string)
          n1043 = call-dynamic "Write cmd.vi"("error in (no error)"=w2759, "cmd"=w2755, "Device in"=w2757) -> ("error out"=w2758:errorcluster, "Device out"=w2760:refnum<class "Channel.lvclass">)  [unwired: 7 in]
          n1044 = Increment(x=w2753) -> (x+1=w2754:i32)
        }
        frame 277 {
          n1045 = call-dynamic "Read resp.vi"("error in (no error)"=w2768, "Device in"=w2769) -> ("error out"=w2762:errorcluster, "resp"=w2767:string, "Device out"=w2763:refnum<class "Channel.lvclass">)  [unwired: 7 in]
          n1046 = Equal?(x=w2767, y="DONE") -> (x = y?=w2765:bool)
          n1047 = case shown="True" w2765 {
            tunnel: [w2770 w2771] -> w2764
            tunnel: w2761 -> [w2770 w2772]
            frame False {
            }
            frame True {
              n1048 = Increment(x=w2772) -> (x+1=w2771:i32)
            }
          }
        }
        frame 278 {
          n1049 = call-dynamic "Write cmd.vi"("error in (no error)"=w2778, "cmd"="GET FINAL_COLUMN", "Device in"=w2776) -> ("error out"=w2777:errorcluster, "Device out"=w2779:refnum<class "Channel.lvclass">)  [unwired: 7 in]
          n1050 = Increment(x=w2774) -> (x+1=w2775:i32)
        }
        frame 279 {
          n1051 = call-dynamic "Read resp.vi"("error in (no error)"=w2790, "Device in"=w2791) -> ("error out"=w2788:errorcluster, "resp"=w2783:string, "Device out"=w2786:refnum<class "Channel.lvclass">)  [unwired: 7 in]
          n1052 = Fract/Exp String To Number(string=w2783) -> (number=w2781:dbl)  [unwired: 3 in, 1 out]
          n1053 = Unbundle By Name(w2786) -> ("Interface.lvclass"=w2785:refnum<class "Interface.lvclass">)
          n1054 = call "Read Camera Setup.vi"("Interface in"=w2785) -> ("Camera Setup"=w2784:T4)  [unwired: 8 in, 2 out]
          n1055 = Unbundle By Name(w2784) -> ("FINAL_COLUMN"=w2780:u16)
          n1056 = Equal?(x=w2780, y=w2781) -> (x = y?=w2782:bool)
          n1057 = disable-structure shown="Enabled" {
            disable-tunnel: [w2794 0 ("State")] -> w2789
            disable-tunnel: w2787 -> [w2793 _]
            disable-tunnel: w2782 -> [w2792 _]
            frame Disabled {
              n1058 = case shown="True" w2792 {
                tunnel: [w2795 w2796] -> w2794
                tunnel: w2793 -> [w2795 w2797]
                frame False {
                }
                frame True {
                  n1059 = Increment(x=w2797) -> (x+1=w2796:i32)
                }
              }
            }
            frame Enabled {
            }
          }
        }
        frame 280 {
          n1060 = Unbundle By Name(w2807) -> ("Interface.lvclass"=w2806:refnum<class "Interface.lvclass">)
          n1061 = call "Read Camera Setup.vi"("Interface in"=w2806) -> ("Camera Setup"=w2800:T4)  [unwired: 8 in, 2 out]
          n1062 = Unbundle By Name(w2800) -> ("VERTICAL_CLOCK_VOLTAGE"=w2799:u8)
          n1063 = Number To Fractional String(number=w2799) -> (F-format string=w2801:string)  [unwired: 3 in]
          n1064 = Concatenate Strings("SET VERTICAL_CLOCK_VOLTAGE " ("cmd"), w2801) -> (w2805:string)
          n1065 = call-dynamic "Write cmd.vi"("error in (no error)"=w2809, "cmd"=w2805, "Device in"=w2807) -> ("error out"=w2808:errorcluster, "Device out"=w2810:refnum<class "Channel.lvclass">)  [unwired: 7 in]
          n1066 = Increment(x=w2803) -> (x+1=w2804:i32)
        }
        frame 281 {
          n1067 = call-dynamic "Read resp.vi"("error in (no error)"=w2818, "Device in"=w2819) -> ("error out"=w2812:errorcluster, "resp"=w2817:string, "Device out"=w2813:refnum<class "Channel.lvclass">)  [unwired: 7 in]
          n1068 = Equal?(x=w2817, y="DONE") -> (x = y?=w2815:bool)
          n1069 = case shown="True" w2815 {
            tunnel: [w2820 w2821] -> w2814
            tunnel: w2811 -> [w2820 w2822]
            frame False {
            }
            frame True {
              n1070 = Increment(x=w2822) -> (x+1=w2821:i32)
            }
          }
        }
        frame 282 {
          n1071 = call-dynamic "Write cmd.vi"("error in (no error)"=w2828, "cmd"="GET VERTICAL_CLOCK_VOLTAGE", "Device in"=w2826) -> ("error out"=w2827:errorcluster, "Device out"=w2829:refnum<class "Channel.lvclass">)  [unwired: 7 in]
          n1072 = Increment(x=w2824) -> (x+1=w2825:i32)
        }
        frame 283 {
          n1073 = call-dynamic "Read resp.vi"("error in (no error)"=w2840, "Device in"=w2841) -> ("error out"=w2838:errorcluster, "resp"=w2833:string, "Device out"=w2836:refnum<class "Channel.lvclass">)  [unwired: 7 in]
          n1074 = Fract/Exp String To Number(string=w2833) -> (number=w2831:dbl)  [unwired: 3 in, 1 out]
          n1075 = Unbundle By Name(w2836) -> ("Interface.lvclass"=w2835:refnum<class "Interface.lvclass">)
          n1076 = call "Read Camera Setup.vi"("Interface in"=w2835) -> ("Camera Setup"=w2834:T4)  [unwired: 8 in, 2 out]
          n1077 = Unbundle By Name(w2834) -> ("VERTICAL_CLOCK_VOLTAGE"=w2830:u8)
          n1078 = Equal?(x=w2830, y=w2831) -> (x = y?=w2832:bool)
          n1079 = case shown="True" w2832 {
            tunnel: [w2842 w2843] -> w2839
            tunnel: w2837 -> [w2842 w2844]
            frame False {
            }
            frame True {
              n1080 = Increment(x=w2844) -> (x+1=w2843:i32)
            }
          }
        }
        frame 284 {
          n1081 = Unbundle By Name(w2853) -> ("Interface.lvclass"=w2852:refnum<class "Interface.lvclass">)
          n1082 = call "Read Camera Setup.vi"("Interface in"=w2852) -> ("Camera Setup"=w2847:T4)  [unwired: 8 in, 2 out]
          n1083 = Unbundle By Name(w2847) -> ("FRAME_TRANSFER"=w2846:bool)
          n1084 = case shown="True" w2846 {
            tunnel: ["T" ("cmd") "F" ("cmd")] -> w2845
            frame True {
            }
            frame False {
            }
          }
          n1085 = Concatenate Strings("SET FRAME_TRANSFER " ("cmd"), w2845) -> (w2851:string)
          n1086 = call-dynamic "Write cmd.vi"("error in (no error)"=w2855, "cmd"=w2851, "Device in"=w2853) -> ("error out"=w2854:errorcluster, "Device out"=w2856:refnum<class "Channel.lvclass">)  [unwired: 7 in]
          n1087 = Increment(x=w2849) -> (x+1=w2850:i32)
        }
        frame 285 {
          n1088 = call-dynamic "Read resp.vi"("error in (no error)"=w2866, "Device in"=w2867) -> ("error out"=w2860:errorcluster, "resp"=w2865:string, "Device out"=w2861:refnum<class "Channel.lvclass">)  [unwired: 7 in]
          n1089 = Equal?(x=w2865, y="DONE") -> (x = y?=w2863:bool)
          n1090 = case shown="True" w2863 {
            tunnel: [w2868 w2869] -> w2862
            tunnel: w2859 -> [w2868 w2870]
            frame False {
            }
            frame True {
              n1091 = Increment(x=w2870) -> (x+1=w2869:i32)
            }
          }
        }
        frame 286 {
          n1092 = call-dynamic "Write cmd.vi"("error in (no error)"=w2876, "cmd"="GET FRAME_TRANSFER", "Device in"=w2874) -> ("error out"=w2875:errorcluster, "Device out"=w2877:refnum<class "Channel.lvclass">)  [unwired: 7 in]
          n1093 = Increment(x=w2872) -> (x+1=w2873:i32)
        }
        frame 287 {
          n1094 = call-dynamic "Read resp.vi"("error in (no error)"=w2888, "Device in"=w2889) -> ("error out"=w2886:errorcluster, "resp"=w2880:string, "Device out"=w2884:refnum<class "Channel.lvclass">)  [unwired: 7 in]
          n1095 = Unbundle By Name(w2884) -> ("Interface.lvclass"=w2883:refnum<class "Interface.lvclass">)
          n1096 = call "Read Camera Setup.vi"("Interface in"=w2883) -> ("Camera Setup"=w2882:T4)  [unwired: 8 in, 2 out]
          n1097 = Unbundle By Name(w2882) -> ("FRAME_TRANSFER"=w2879:bool)
          n1098 = case shown="True" w2879 {
            tunnel: ["T" "F"] -> w2878
            frame True {
            }
            frame False {
            }
          }
          n1099 = Equal?(x=w2878, y=w2880) -> (x = y?=w2881:bool)
          n1100 = case shown="True" w2881 {
            tunnel: [w2892 w2893] -> w2887
            tunnel: w2885 -> [w2892 w2894]
            frame False {
            }
            frame True {
              n1101 = Increment(x=w2894) -> (x+1=w2893:i32)
            }
          }
        }
        frame 288 {
          n1102 = Unbundle By Name(w2903) -> ("Interface.lvclass"=w2902:refnum<class "Interface.lvclass">)
          n1103 = call "Read Camera Setup.vi"("Interface in"=w2902) -> ("Camera Setup"=w2896:T4)  [unwired: 8 in, 2 out]
          n1104 = Unbundle By Name(w2896) -> ("AD_CHANNEL"=w2895:u32)
          n1105 = Number To Fractional String(number=w2895) -> (F-format string=w2897:string)  [unwired: 3 in]
          n1106 = Concatenate Strings("SET AD_CHANNEL " ("cmd"), w2897) -> (w2901:string)
          n1107 = call-dynamic "Write cmd.vi"("error in (no error)"=w2905, "cmd"=w2901, "Device in"=w2903) -> ("error out"=w2904:errorcluster, "Device out"=w2906:refnum<class "Channel.lvclass">)  [unwired: 7 in]
          n1108 = Increment(x=w2899) -> (x+1=w2900:i32)
        }
        frame 289 {
          n1109 = call-dynamic "Read resp.vi"("error in (no error)"=w2914, "Device in"=w2915) -> ("error out"=w2908:errorcluster, "resp"=w2913:string, "Device out"=w2909:refnum<class "Channel.lvclass">)  [unwired: 7 in]
          n1110 = Equal?(x=w2913, y="DONE") -> (x = y?=w2911:bool)
          n1111 = case shown="True" w2911 {
            tunnel: [w2916 w2917] -> w2910
            tunnel: w2907 -> [w2916 w2918]
            frame False {
            }
            frame True {
              n1112 = Increment(x=w2918) -> (x+1=w2917:i32)
            }
          }
        }
        frame 290 {
          n1113 = call-dynamic "Write cmd.vi"("error in (no error)"=w2924, "cmd"="GET AD_CHANNEL", "Device in"=w2922) -> ("error out"=w2923:errorcluster, "Device out"=w2925:refnum<class "Channel.lvclass">)  [unwired: 7 in]
          n1114 = Increment(x=w2920) -> (x+1=w2921:i32)
        }
        frame 291 {
          n1115 = call-dynamic "Read resp.vi"("error in (no error)"=w2936, "Device in"=w2937) -> ("error out"=w2934:errorcluster, "resp"=w2929:string, "Device out"=w2932:refnum<class "Channel.lvclass">)  [unwired: 7 in]
          n1116 = Fract/Exp String To Number(string=w2929) -> (number=w2927:dbl)  [unwired: 3 in, 1 out]
          n1117 = Unbundle By Name(w2932) -> ("Interface.lvclass"=w2931:refnum<class "Interface.lvclass">)
          n1118 = call "Read Camera Setup.vi"("Interface in"=w2931) -> ("Camera Setup"=w2930:T4)  [unwired: 8 in, 2 out]
          n1119 = Unbundle By Name(w2930) -> ("AD_CHANNEL"=w2926:u32)
          n1120 = Equal?(x=w2926, y=w2927) -> (x = y?=w2928:bool)
          n1121 = case shown="True" w2928 {
            tunnel: [w2938 w2939] -> w2935
            tunnel: w2933 -> [w2938 w2940]
            frame False {
            }
            frame True {
              n1122 = Increment(x=w2940) -> (x+1=w2939:i32)
            }
          }
        }
        frame 300 {
          # "suffix"
          n1123 = call-dynamic "Write Timer.vi"("error in (no error)"=w2946, "Timer"=u32 200, "State Machine in"=w2949) -> ("error out"=w2950:errorcluster, "State Machine out"=w2944:refnum<class "State Machine.lvclass">)  [unwired: 7 in]
          n1124 = call-dynamic "Write State Machine.vi"("error in (no error)"=w2950, "State Machine.lvclass"=w2944, "Device in"=w2947) -> ("error out"=w2945:errorcluster, "Device out"=w2943:refnum<class "Channel.lvclass">)  [unwired: 7 in]
          n1125 = Bundle By Name(cluster=w2943, "config"=TRUE) -> (w2942:refnum<class "Channel.lvclass">)
          n1126 = Unbundle By Name(w2942) -> ("Interface.lvclass"=w2956:refnum<class "Interface.lvclass">)
          n1127 = call-dynamic "Read Suffix.vi"("Interface in"=w2956) -> ("Suffix"=w2951:string)  [unwired: 8 in, 2 out]
          n1128 = Concatenate Strings("SET SUFFIX " ("cmd"), w2951) -> (w2955:string)
          n1129 = call-dynamic "Write cmd.vi"("error in (no error)"=w2945, "cmd"=w2955, "Device in"=w2942) -> ("error out"=w2957:errorcluster, "Device out"=w2958:refnum<class "Channel.lvclass">)  [unwired: 7 in]
          n1130 = Increment(x=w2953) -> (x+1=w2954:i32)
        }
        frame 301 {
          # "Compara o parametro enviado com\no parametro no Acquisition Configuration\nda msg de STATUS do ACS."
          # "Verifica timeout para ACS responder.\nSe estourar timeout é porque o ACS não \nrespondeu e este canal volta para o estado 0\npara não \"travar\" os outros canais no \nS4ACS_GUI:HandleObservation.vi."
          n1131 = call "Verify Timer.vi"("error in (no error)"=w2990, "State Machine in"=w2992) -> ("error out"=w2989:errorcluster, "timeout"=w2987:bool, "State Machine out"=w2991:refnum<class "State Machine.lvclass">)  [unwired: 7 in]
          n1132 = call-dynamic "Write State Machine.vi"("error in (no error)"=w2989, "State Machine.lvclass"=w2991, "Device in"=w2993) -> ("error out"=w2988:errorcluster, "Device out"=w2984:refnum<class "Channel.lvclass">)  [unwired: 7 in]
          n1133 = call-dynamic "Read resp.vi"("error in (no error)"=w2988, "Device in"=w2984) -> ("error out"=w2978:errorcluster, "resp"=w2962:string, "Device out"=w2983:refnum<class "Channel.lvclass">)  [unwired: 7 in]
          n1134 = Unbundle By Name(w2983) -> ("Interface.lvclass"=w2982:refnum<class "Interface.lvclass">)
          n1135 = call-dynamic "UpdateACQconf.vi"("error in (no error)"=w2978, "status"=w2962, "Interface in"=w2982) -> ("error out"=w2977:errorcluster, "ACQ conf rx"=w2980:T2, "Interface out"=w2981:refnum<class "Interface.lvclass">)  [unwired: 6 in]
          n1136 = Unbundle By Name(w2980) -> ("suffix"=w2979:string)
          n1137 = call-dynamic "Read Suffix.vi"("error in (no error)"=w2977, "Interface in"=w2981) -> ("error out"=w2961:errorcluster, "Suffix"=w2976:string, "Interface out"=w2964:refnum<class "Interface.lvclass">)  [unwired: 7 in]
          n1138 = Equal?(x=w2976, y=w2979) -> (x = y?=w2975:bool)
          n1139 = call-dynamic "UpdateS4GUI_JSON_string.vi"("error in (no error)"=w2961, "status"=w2962, "Interface in"=w2964) -> ("error out"=w2960:errorcluster, "S4GUI JSON string rx"=w2959:T5, "Interface out"=w2963:refnum<class "Interface.lvclass">)  [unwired: 6 in]
          n1140 = Unbundle By Name(w2959) -> ("OBSTYPE"=w2968:string, "OBJECT"=w2967:string)
          n1141 = call-dynamic "Read ObsType.vi"("error in (no error)"=w2960, "Interface in"=w2963) -> ("error out"=w2973:errorcluster, "ObsType"=w2970:string, "Interface out"=w2971:refnum<class "Interface.lvclass">)  [unwired: 7 in]
          n1142 = call-dynamic "Read Object.vi"("error in (no error)"=w2973, "Interface in"=w2971) -> ("error out"=w2972:errorcluster, "Object"=w2969:string)  [unwired: 7 in, 1 out]
          n1143 = Equal?(x=w2970, y=w2968) -> (x = y?=w2966:bool)
          n1144 = Equal?(x=w2969, y=w2967) -> (x = y?=w2965:bool)
          n1145 = disable-structure shown="Enabled" {
            disable-tunnel: w2975 -> [w2997 w2998]
            disable-tunnel: [w2996 w2998] -> w2974
            disable-tunnel: w2966 -> [w2995 _]
            disable-tunnel: w2965 -> [w2994 _]
            frame Enabled {
              n1146 = Compound Arithmetic op=AND(w2997, w2995, w2994) -> (w2996:bool)
            }
            frame Disabled {
            }
          }
          n1147 = case shown="True" w2987 {
            tunnel: [w3000 27] -> w2985
            tunnel: w2986 -> [w3001 _]
            tunnel: w2974 -> [w2999 _]
            frame False {
              n1148 = case shown="True" w2999 {
                tunnel: [w3002 w3003] -> w3000
                tunnel: w3001 -> [w3002 w3004]
                frame False {
                }
                frame True {
                  n1149 = Increment(x=w3004) -> (x+1=w3003:i32)
                }
              }
            }
            frame True {
              # "ERRO"
            }
          }
        }
        frame 302 {
          # "Não espera nada."
          # "2024-03-20:\nSó envia o SUFFIX por comando SET.\nO resto dos parametros estão na  \npublicação do STATUS do S4GUI.\nVai para 40 configurar o EXPOSE mode"
          n1150 = call "Verify Timer.vi"("error in (no error)"=w3014, "State Machine in"=w3015) -> ("error out"=w3011:errorcluster, "State Machine out"=w3012:refnum<class "State Machine.lvclass">)  [unwired: 7 in, 1 out]
          n1151 = call-dynamic "Write State Machine.vi"("error in (no error)"=w3011, "State Machine.lvclass"=w3012, "Device in"=w3013) -> ("error out"=w3010:errorcluster, "Device out"=w3009:refnum<class "Channel.lvclass">)  [unwired: 7 in]
          n1152 = case shown="True" TRUE {
            tunnel: [w3016 0 ("State")] -> w3008
            tunnel: w3007 -> [w3016 _]
            frame False {
            }
            frame True {
              (unwired) 40 ("State")
            }
          }
        }
        frame 305 {
          # "Comando enviado para ajustar ExpTime quando se troca de abas em TabAcqType (chamado por S4GUI.vi - evento \"Tab Acq Type: Value Change\""
          # "Vai pra 20 validar\no ACK."
          # "Carrega timeout de 200 ciclos\npara resposta do ACS e salva\no proximo estado como estado \nde retorno."
          n1153 = call-dynamic "Write Timer.vi"("error in (no error)"=w3037, "Timer"=u32 200, "State Machine in"=w3036) -> ("error out"=w3027:errorcluster, "State Machine out"=w3029:refnum<class "State Machine.lvclass">)  [unwired: 7 in]
          n1154 = Increment(x=w3025) -> (x+1=w3024:i32)
          n1155 = call-dynamic "Write Return State.vi"("error in (no error)"=w3027, "Return State"=w3024, "State Machine in"=w3029) -> ("error out"=w3026:errorcluster, "State Machine out"=w3028:refnum<class "State Machine.lvclass">)  [unwired: 7 in]
          n1156 = call-dynamic "Write State Machine.vi"("error in (no error)"=w3026, "State Machine.lvclass"=w3028, "Device in"=w3035) -> ("error out"=w3033:errorcluster, "Device out"=w3032:refnum<class "Channel.lvclass">)  [unwired: 7 in]
          n1157 = Bundle By Name(cluster=w3032, "config"=TRUE) -> (w3031:refnum<class "Channel.lvclass">)
          n1158 = Unbundle By Name(w3031) -> ("Interface.lvclass"=w3023:refnum<class "Interface.lvclass">)
          n1159 = call "Read Exposure Time.vi"("Interface in"=w3023) -> ("Exposure Time"=w3022:dbl)  [unwired: 8 in, 2 out]
          n1160 = Number To Fractional String(use system decimal point (T)=FALSE, number=w3022) -> (F-format string=w3021:string)  [unwired: 2 in]
          n1161 = Concatenate Strings("SET EXPTIME " ("cmd"), w3021) -> (w3020:string)
          n1162 = call-dynamic "Write cmd.vi"("error in (no error)"=w3033, "cmd"=w3020, "Device in"=w3031) -> ("error out"=w3039:errorcluster, "Device out"=w3040:refnum<class "Channel.lvclass">)  [unwired: 7 in]
        }
        frame 306 {
          # "Compara o parametro enviado com\no parametro no Acquisition Configuration\nda msg de STATUS do ACS."
          # "Verifica timeout para ACS responder.\nSe estourar timeout é porque o ACS não \nrespondeu e este canal vai para 28 para \nque o erro seja detectado em\nS4ACS_GUI:HandleObservation.vi."
          n1163 = call "Verify Timer.vi"("error in (no error)"=w3058, "State Machine in"=w3060) -> ("error out"=w3057:errorcluster, "timeout"=w3055:bool, "State Machine out"=w3059:refnum<class "State Machine.lvclass">)  [unwired: 7 in]
          n1164 = call-dynamic "Write State Machine.vi"("error in (no error)"=w3057, "State Machine.lvclass"=w3059, "Device in"=w3061) -> ("error out"=w3056:errorcluster, "Device out"=w3052:refnum<class "Channel.lvclass">)  [unwired: 7 in]
          n1165 = call-dynamic "Read resp.vi"("error in (no error)"=w3056, "Device in"=w3052) -> ("error out"=w3043:errorcluster, "resp"=w3051:string, "Device out"=w3050:refnum<class "Channel.lvclass">)  [unwired: 7 in]
          n1166 = Unbundle By Name(w3050) -> ("Interface.lvclass"=w3049:refnum<class "Interface.lvclass">)
          n1167 = call-dynamic "UpdateACQconf.vi"("error in (no error)"=w3043, "status"=w3051, "Interface in"=w3049) -> ("error out"=w3042:errorcluster, "ACQ conf rx"=w3047:T2, "Interface out"=w3048:refnum<class "Interface.lvclass">)  [unwired: 6 in]
          n1168 = Unbundle By Name(w3047) -> ("EXPTIME"=w3045:dbl)
          n1169 = call "Read Exposure Time.vi"("error in (no error)"=w3042, "Interface in"=w3048) -> ("error out"=w3041:errorcluster, "Exposure Time"=w3046:dbl)  [unwired: 7 in, 1 out]
          n1170 = Equal?(x=w3046, y=w3045) -> (x = y?=w3044:bool)
          n1171 = case shown="False" w3055 {
            tunnel: [w3063 27] -> w3053
            tunnel: w3054 -> [w3064 _]
            tunnel: w3044 -> [w3062 _]
            frame False {
              n1172 = case shown="True" w3062 {
                tunnel: [w3065 0 ("State")] -> w3063
                tunnel: w3064 -> [w3065 _]
                frame False {
                }
                frame True {
                }
              }
            }
            frame True {
              # "ERRO"
            }
          }
        }
        frame 312 {
          # "filter"
          n1173 = call-dynamic "Write Timer.vi"("error in (no error)"=w3073, "Timer"=u32 50, "State Machine in"=w3071) -> ("error out"=w3078:errorcluster, "State Machine out"=w3076:refnum<class "State Machine.lvclass">)  [unwired: 7 in]
          n1174 = call-dynamic "Write State Machine.vi"("error in (no error)"=w3078, "State Machine.lvclass"=w3076, "Device in"=w3075) -> ("error out"=w3068:errorcluster, "Device out"=w3074:refnum<class "Channel.lvclass">)  [unwired: 7 in]
          n1175 = Unbundle By Name(w3074) -> ("Filter"=w3070:u8)
          n1176 = case shown="0, Default" w3070 {
            tunnel: ["U" ("cmd") "B" ("cmd") "V" ("cmd") "R" ("cmd") "I" ("cmd") "CLEAR" ("cmd")] -> w3069
            frame 1 {
            }
            frame 2 {
            }
            frame 3 {
            }
            frame 4 {
            }
            frame 5 {
            }
            frame 0, Default {
            }
          }
          n1177 = Concatenate Strings("SET FILTER " ("cmd"), w3069) -> (w3081:string)
          n1178 = call-dynamic "Write cmd.vi"("error in (no error)"=w3068, "cmd"=w3081, "Device in"=w3074) -> ("error out"=w3082:errorcluster, "Device out"=w3083:refnum<class "Channel.lvclass">)  [unwired: 7 in]
          n1179 = Increment(x=w3079) -> (x+1=w3080:i32)
        }
        frame 313 {
          n1180 = call "Verify Timer.vi"("error in (no error)"=w3098, "State Machine in"=w3096) -> ("error out"=w3097:errorcluster, "timeout"=w3093:bool, "State Machine out"=w3100:refnum<class "State Machine.lvclass">)  [unwired: 7 in]
          n1181 = call-dynamic "Write State Machine.vi"("error in (no error)"=w3097, "State Machine.lvclass"=w3100, "Device in"=w3099) -> ("error out"=w3094:errorcluster, "Device out"=w3095:refnum<class "Channel.lvclass">)  [unwired: 7 in]
          n1182 = call-dynamic "Read resp.vi"("error in (no error)"=w3094, "Device in"=w3095) -> ("error out"=w3101:errorcluster, "resp"=w3104:string, "Device out"=w3102:refnum<class "Channel.lvclass">)  [unwired: 7 in]
          n1183 = Equal?(x=w3104, y="DONE") -> (x = y?=w3091:bool)
          n1184 = case shown="False" w3093 {
            tunnel: [w3106 0] -> w3090
            tunnel: w3092 -> [w3107 _]
            tunnel: w3091 -> [w3105 _]
            frame False {
              n1185 = case shown="True" w3105 {
                tunnel: w3107 -> [w3108 w3110]
                tunnel: [w3108 w3109] -> w3106
                frame False {
                }
                frame True {
                  n1186 = Increment(x=w3110) -> (x+1=w3109:i32)
                }
              }
            }
            frame True {
            }
          }
        }
        frame 314 {
          n1187 = call-dynamic "Write Timer.vi"("error in (no error)"=w3115, "Timer"=u32 50, "State Machine in"=w3114) -> ("error out"=w3120:errorcluster, "State Machine out"=w3118:refnum<class "State Machine.lvclass">)  [unwired: 7 in]
          n1188 = call-dynamic "Write State Machine.vi"("error in (no error)"=w3120, "State Machine.lvclass"=w3118, "Device in"=w3117) -> ("error out"=w3113:errorcluster, "Device out"=w3116:refnum<class "Channel.lvclass">)  [unwired: 7 in]
          n1189 = call-dynamic "Write cmd.vi"("error in (no error)"=w3113, "cmd"="SET CTRLINTE S4GUI", "Device in"=w3116) -> ("error out"=w3123:errorcluster, "Device out"=w3124:refnum<class "Channel.lvclass">)  [unwired: 7 in]
          n1190 = Increment(x=w3121) -> (x+1=w3122:i32)
        }
        frame 315 {
          n1191 = call "Verify Timer.vi"("error in (no error)"=w3133, "State Machine in"=w3131) -> ("error out"=w3132:errorcluster, "timeout"=w3128:bool, "State Machine out"=w3135:refnum<class "State Machine.lvclass">)  [unwired: 7 in]
          n1192 = call-dynamic "Write State Machine.vi"("error in (no error)"=w3132, "State Machine.lvclass"=w3135, "Device in"=w3134) -> ("error out"=w3129:errorcluster, "Device out"=w3130:refnum<class "Channel.lvclass">)  [unwired: 7 in]
          n1193 = call-dynamic "Read resp.vi"("error in (no error)"=w3129, "Device in"=w3130) -> ("error out"=w3136:errorcluster, "resp"=w3139:string, "Device out"=w3137:refnum<class "Channel.lvclass">)  [unwired: 7 in]
          n1194 = Equal?(x=w3139, y="DONE") -> (x = y?=w3126:bool)
          n1195 = case shown="False" w3128 {
            tunnel: [w3141 0] -> w3125
            tunnel: w3127 -> [w3142 _]
            tunnel: w3126 -> [w3140 _]
            frame False {
              n1196 = case shown="True" w3140 {
                tunnel: w3142 -> [w3143 w3145]
                tunnel: [w3143 w3144] -> w3141
                frame False {
                }
                frame True {
                  n1197 = Increment(x=w3145) -> (x+1=w3144:i32)
                }
              }
            }
            frame True {
            }
          }
        }
        frame 316 {
          # "Carrega timeout de 50 ciclos\npara resposta do ACS"
          n1198 = call-dynamic "Write Timer.vi"("error in (no error)"=w3155, "Timer"=u32 50, "State Machine in"=w3154) -> ("error out"=w3157:errorcluster, "State Machine out"=w3159:refnum<class "State Machine.lvclass">)  [unwired: 7 in]
          n1199 = call-dynamic "Write State Machine.vi"("error in (no error)"=w3157, "State Machine.lvclass"=w3159, "Device in"=w3156) -> ("error out"=w3149:errorcluster, "Device out"=w3148:refnum<class "Channel.lvclass">)  [unwired: 7 in]
          n1200 = Unbundle By Name(w3148) -> ("rotator"=w3147:dbl)
          n1201 = Number To Fractional String(number=w3147) -> (F-format string=w3151:string)  [unwired: 3 in]
          n1202 = Concatenate Strings("SET INSTROT " ("cmd"), w3151) -> (w3150:string)
          n1203 = call-dynamic "Write cmd.vi"("error in (no error)"=w3149, "cmd"=w3150, "Device in"=w3148) -> ("error out"=w3161:errorcluster, "Device out"=w3162:refnum<class "Channel.lvclass">)  [unwired: 7 in]
          n1204 = Increment(x=w3153) -> (x+1=w3160:i32)
        }
        frame 317 {
          n1205 = call "Verify Timer.vi"("error in (no error)"=w3167, "State Machine in"=w3168) -> ("error out"=w3172:errorcluster, "timeout"=w3164:bool, "State Machine out"=w3173:refnum<class "State Machine.lvclass">)  [unwired: 7 in]
          n1206 = call-dynamic "Write State Machine.vi"("error in (no error)"=w3172, "State Machine.lvclass"=w3173, "Device in"=w3171) -> ("error out"=w3169:errorcluster, "Device out"=w3170:refnum<class "Channel.lvclass">)  [unwired: 7 in]
          n1207 = call-dynamic "Read resp.vi"("error in (no error)"=w3169, "Device in"=w3170) -> ("error out"=w3174:errorcluster, "resp"=w3177:string, "Device out"=w3175:refnum<class "Channel.lvclass">)  [unwired: 7 in]
          n1208 = Equal?(x=w3177, y="DONE") -> (x = y?=w3163:bool)
          n1209 = case shown="False" w3164 {
            tunnel: [w3179 0] -> w3166
            tunnel: w3165 -> [w3180 _]
            tunnel: w3163 -> [w3178 _]
            frame False {
              n1210 = case shown="True" w3178 {
                tunnel: [w3181 w3182] -> w3179
                tunnel: w3180 -> [w3181 w3183]
                frame False {
                }
                frame True {
                  n1211 = Increment(x=w3183) -> (x+1=w3182:i32)
                }
              }
            }
            frame True {
            }
          }
        }
        frame 318 {
          # "Carrega timeout de 50 ciclos\npara resposta do ACS"
          n1212 = call-dynamic "Write Timer.vi"("error in (no error)"=w3192, "Timer"=u32 50, "State Machine in"=w3191) -> ("error out"=w3194:errorcluster, "State Machine out"=w3196:refnum<class "State Machine.lvclass">)  [unwired: 7 in]
          n1213 = call-dynamic "Write State Machine.vi"("error in (no error)"=w3194, "State Machine.lvclass"=w3196, "Device in"=w3193) -> ("error out"=w3187:errorcluster, "Device out"=w3186:refnum<class "Channel.lvclass">)  [unwired: 7 in]
          n1214 = Unbundle By Name(w3186) -> ("TCS mode"=w3185:string)
          n1215 = Concatenate Strings("SET TCSMODE " ("cmd"), w3185) -> (w3188:string)
          n1216 = call-dynamic "Write cmd.vi"("error in (no error)"=w3187, "cmd"=w3188, "Device in"=w3186) -> ("error out"=w3198:errorcluster, "Device out"=w3199:refnum<class "Channel.lvclass">)  [unwired: 7 in]
          n1217 = Increment(x=w3190) -> (x+1=w3197:i32)
        }
        frame 319 {
          n1218 = call "Verify Timer.vi"("error in (no error)"=w3204, "State Machine in"=w3205) -> ("error out"=w3209:errorcluster, "timeout"=w3201:bool, "State Machine out"=w3210:refnum<class "State Machine.lvclass">)  [unwired: 7 in]
          n1219 = call-dynamic "Write State Machine.vi"("error in (no error)"=w3209, "State Machine.lvclass"=w3210, "Device in"=w3208) -> ("error out"=w3206:errorcluster, "Device out"=w3207:refnum<class "Channel.lvclass">)  [unwired: 7 in]
          n1220 = call-dynamic "Read resp.vi"("error in (no error)"=w3206, "Device in"=w3207) -> ("error out"=w3211:errorcluster, "resp"=w3214:string, "Device out"=w3212:refnum<class "Channel.lvclass">)  [unwired: 7 in]
          n1221 = Equal?(x=w3214, y="DONE") -> (x = y?=w3200:bool)
          n1222 = case shown="False" w3201 {
            tunnel: [w3216 0] -> w3203
            tunnel: w3202 -> [w3217 _]
            tunnel: w3200 -> [w3215 _]
            frame False {
              n1223 = case shown="True" w3215 {
                tunnel: [w3218 w3219] -> w3216
                tunnel: w3217 -> [w3218 w3220]
                frame False {
                }
                frame True {
                  n1224 = Increment(x=w3220) -> (x+1=w3219:i32)
                }
              }
            }
            frame True {
            }
          }
        }
        frame 320 {
          # "Carrega timeout de 50 ciclos\npara resposta do ACS"
          n1225 = call-dynamic "Write Timer.vi"("error in (no error)"=w3229, "Timer"=u32 50, "State Machine in"=w3228) -> ("error out"=w3231:errorcluster, "State Machine out"=w3233:refnum<class "State Machine.lvclass">)  [unwired: 7 in]
          n1226 = call-dynamic "Write State Machine.vi"("error in (no error)"=w3231, "State Machine.lvclass"=w3233, "Device in"=w3230) -> ("error out"=w3224:errorcluster, "Device out"=w3223:refnum<class "Channel.lvclass">)  [unwired: 7 in]
          n1227 = Unbundle By Name(w3223) -> ("ICS mode"=w3222:string)
          n1228 = Concatenate Strings("SET ICSMODE " ("cmd"), w3222) -> (w3225:string)
          n1229 = call-dynamic "Write cmd.vi"("error in (no error)"=w3224, "cmd"=w3225, "Device in"=w3223) -> ("error out"=w3235:errorcluster, "Device out"=w3236:refnum<class "Channel.lvclass">)  [unwired: 7 in]
          n1230 = Increment(x=w3227) -> (x+1=w3234:i32)
        }
        frame 321 {
          n1231 = call "Verify Timer.vi"("error in (no error)"=w3241, "State Machine in"=w3242) -> ("error out"=w3246:errorcluster, "timeout"=w3240:bool, "State Machine out"=w3247:refnum<class "State Machine.lvclass">)  [unwired: 7 in]
          n1232 = call-dynamic "Write State Machine.vi"("error in (no error)"=w3246, "State Machine.lvclass"=w3247, "Device in"=w3245) -> ("error out"=w3243:errorcluster, "Device out"=w3244:refnum<class "Channel.lvclass">)  [unwired: 7 in]
          n1233 = call-dynamic "Read resp.vi"("error in (no error)"=w3243, "Device in"=w3244) -> ("error out"=w3248:errorcluster, "resp"=w3251:string, "Device out"=w3249:refnum<class "Channel.lvclass">)  [unwired: 7 in]
          n1234 = Equal?(x=w3251, y="DONE") -> (x = y?=w3238:bool)
          n1235 = case shown="False" w3240 {
            tunnel: [w3253 w3259] -> w3237
            tunnel: w3239 -> [w3254 _]
            tunnel: w3238 -> [w3252 _]
            frame False {
              n1236 = case shown="True" w3252 {
                tunnel: [w3255 w3256] -> w3253
                tunnel: w3254 -> [w3255 _]
                frame False {
                }
                frame True {
                  n1237 = disable-structure shown="Enabled" {
                    disable-tunnel: [0 ("State") 40] -> w3256
                    frame Disabled {
                    }
                    frame Enabled {
                      # "Configura\nExpMode"
                    }
                  }
                }
              }
            }
            frame True {
              n1238 = disable-structure shown="Enabled" {
                disable-tunnel: [0 40] -> w3259
                frame Enabled {
                }
                frame Disabled {
                  # "Configura\nExpMode"
                }
              }
            }
          }
        }
      }
      n1239 = call-dynamic "Read State Machine.vi"("error in (no error)"=w7, "Device in"=w14) -> ("error out"=w10:errorcluster, "State Machine.lvclass"=w13:refnum<class "State Machine.lvclass">, "Device out"=w12:refnum<class "Channel.lvclass">)  [unwired: 7 in]
      n1240 = call "Next State.vi"("error in (no error)"=w10, "New_State"=w8, "State Machine in"=w13) -> ("error out"=w9:errorcluster, "State Machine out"=w15:refnum<class "State Machine.lvclass">)  [unwired: 7 in]
      n1241 = call-dynamic "Write State Machine.vi"("error in (no error)"=w9, "State Machine.lvclass"=w15, "Device in"=w12) -> ("error out"=w6:errorcluster, "Device out"=w11:refnum<class "Channel.lvclass">)  [unwired: 7 in]
    }
    frame Error {
    }
  }
  "error out" <- w3
  "Channel out" <- w1
